vi "project.vi"() -> ()   [LabVIEW 2017]
panel:
  in  "aOK Button 75":bool
  in  "aOK Button 74":bool
  in  "aOK Button 65":bool
  in  "aOK Button 73":bool
  in  "aOK Button 72":bool
  in  "aOK Button 71":bool
  in  "aOK Button 70":bool
  in  "aOK Button 69":bool
  in  "aOK Button 68":bool
  in  "aOK Button 67":bool
  in  "aOK Button 66":bool
  in  "aOK Button 64":bool
  in  "aOK Button 63":bool
  in  "aOK Button 62":bool
  in  "aOK Button 61":bool
  in  "aOK Button 60":bool
  in  "aOK Button 59":bool
  in  "aOK Button 58":bool
  in  "aOK Button 56":bool
  in  "aOK Button 55":bool
  in  "aOK Button 54":bool
  in  "aOK Button 53":bool
  in  "aOK Button 52":bool
  in  "aOK Button 51":bool
  in  "aOK Button 50":bool
  in  "aOK Button 49":bool
  in  "aOK Button 48":bool
  in  "aOK Button 47":bool
  in  "aOK Button 46":bool
  in  "aOK Button 45":bool
  in  "aOK Button 44":bool
  in  "aOK Button 42":bool
  in  "aOK Button 41":bool
  in  "aOK Button 40":bool
  in  "aOK Button 39":bool
  in  "aOK Button 38":bool
  in  "aOK Button 37":bool
  in  "aOK Button 36":bool
  in  "aOK Button 30":bool
  in  "aOK Button 27":bool
  in  "aOK Button 34":bool
  in  "aOK Button 35":bool
  in  "aOK Button 33":bool
  in  "aOK Button 32":bool
  in  "aOK Button 31":bool
  in  "aOK Button 29":bool
  in  "aOK Button 28":bool
  in  "aOK Button 26":bool
  in  "aOK Button 25":bool
  in  "aOK Button 24":bool
  in  "aOK Button 23":bool
  in  "aOK Button 22":bool
  in  "aOK Button 21":bool
  in  "aOK Button 20":bool
  in  "aOK Button 19":bool
  in  "aOK Button 18":bool
  in  "aOK Button 17":bool
  in  "aOK Button 15":bool
  in  "aOK Button 14":bool
  in  "aOK Button 13":bool
  in  "aOK Button 12":bool
  in  "aOK Button 11":bool
  in  "aOK Button 10":bool
  in  "aOK Button 9":bool
  in  "aOK Button 8":bool
  in  "aOK Button 7":bool
  in  "aOK Button 6":bool
  in  "aOK Button 5":bool
  in  "aOK Button 4":bool
  in  "aOK Button 3":bool
  in  "aOK Button 2":bool
  in  "aOK Button":bool
  out "Boolean 143":bool
  in  "Array 2":bool[][](array[boolean])
  in  "OK Button 165":bool
  in  "OK Button 164":bool
  in  "OK Button 163":bool
  in  "OK Button 162":bool
  in  "OK Button 161":bool
  in  "OK Button 160":bool
  in  "OK Button 159":bool
  in  "OK Button 158":bool
  in  "OK Button 157":bool
  in  "OK Button 156":bool
  in  "OK Button 155":bool
  in  "OK Button 154":bool
  in  "OK Button 153":bool
  in  "OK Button 152":bool
  in  "OK Button 151":bool
  in  "OK Button 150":bool
  in  "OK Button 149":bool
  in  "OK Button 148":bool
  in  "OK Button 147":bool
  in  "OK Button 146":bool
  in  "OK Button 145":bool
  in  "OK Button 144":bool
  in  "OK Button 143":bool
  in  "OK Button 142":bool
  in  "OK Button 141":bool
  in  "OK Button 140":bool
  in  "OK Button 139":bool
  in  "OK Button 138":bool
  in  "OK Button 137":bool
  in  "OK Button 136":bool
  in  "OK Button 135":bool
  in  "OK Button 134":bool
  in  "OK Button 133":bool
  in  "OK Button 132":bool
  in  "OK Button 131":bool
  in  "OK Button 130":bool
  in  "OK Button 129":bool
  in  "OK Button 128":bool
  in  "OK Button 127":bool
  in  "OK Button 126":bool
  in  "OK Button 125":bool
  in  "OK Button 124":bool
  in  "OK Button 122":bool
  in  "OK Button 118":bool
  in  "OK Button 113":bool
  in  "OK Button 104":bool
  in  "OK Button 89":bool
  in  "OK Button 121":bool
  in  "OK Button 117":bool
  in  "OK Button 112":bool
  in  "OK Button 103":bool
  in  "OK Button 88":bool
  in  "OK Button 123":bool
  in  "OK Button 120":bool
  in  "OK Button 119":bool
  in  "OK Button 116":bool
  in  "OK Button 115":bool
  in  "OK Button 114":bool
  in  "OK Button 111":bool
  in  "OK Button 110":bool
  in  "OK Button 109":bool
  in  "OK Button 108":bool
  in  "OK Button 107":bool
  in  "OK Button 105":bool
  in  "OK Button 102":bool
  in  "OK Button 101":bool
  in  "OK Button 100":bool
  in  "OK Button 99":bool
  in  "OK Button 97":bool
  in  "OK Button 96":bool
  in  "OK Button 95":bool
  in  "OK Button 93":bool
  in  "OK Button 92":bool
  in  "OK Button 91":bool
  in  "OK Button 90":bool
  in  "OK Button 87":bool
  in  "OK Button 86":bool
  in  "OK Button 85":bool
  in  "OK Button 84":bool
  in  "OK Button 83":bool
  in  "OK Button 82":bool
  in  "OK Button 81":bool
  in  "OK Button 80":bool
  in  "OK Button 79":bool
  in  "OK Button 78":bool
  in  "OK Button 77":bool
  in  "Array":bool[][](array[boolean])
  out "Boolean 142":bool
  in  "OK Button 76":bool
  in  "OK Button 75":bool
  in  "OK Button 74":bool
  in  "OK Button 73":bool
  in  "OK Button 72":bool
  in  "OK Button 71":bool
  in  "OK Button 70":bool
  in  "OK Button 69":bool
  in  "OK Button 68":bool
  in  "OK Button 59":bool
  in  "OK Button 50":bool
  in  "OK Button 49":bool
  in  "OK Button 67":bool
  in  "OK Button 58":bool
  in  "OK Button 66":bool
  in  "OK Button 48":bool
  in  "OK Button 65":bool
  in  "OK Button 46":bool
  in  "OK Button 45":bool
  in  "OK Button 64":bool
  in  "OK Button 57":bool
  in  "OK Button 44":bool
  in  "OK Button 63":bool
  in  "OK Button 62":bool
  in  "OK Button 61":bool
  in  "OK Button 60":bool
  out "Boolean 141":bool
  in  "OK Button 56":bool
  in  "OK Button 55":bool
  in  "OK Button 54":bool
  in  "OK Button 53":bool
  in  "OK Button 52":bool
  in  "OK Button 51":bool
  in  "OK Button 47":bool
  in  "OK Button 43":bool
  in  "OK Button 42":bool
  in  "OK Button 41":bool
  in  "OK Button 40":bool
  in  "OK Button 39":bool
  in  "OK Button 38":bool
  in  "OK Button 37":bool
  in  "OK Button 36":bool
  in  "OK Button 35":bool
  in  "OK Button 34":bool
  in  "OK Button 33":bool
  in  "OK Button 32":bool
  in  "OK Button 31":bool
  in  "Boolean 140":bool
  in  "Boolean 139":bool
  in  "Boolean 138":bool
  in  "Boolean 137":bool
  in  "Boolean 136":bool
  in  "Boolean 135":bool
  in  "Boolean 134":bool
  in  "Boolean 133":bool
  in  "Boolean 132":bool
  in  "Boolean 131":bool
  in  "Boolean 130":bool
  in  "OK Button 28":bool
  in  "OK Button 27":bool
  in  "OK Button 26":bool
  in  "OK Button 25":bool
  in  "OK Button 24":bool
  in  "OK Button 23":bool
  in  "OK Button 22":bool
  in  "OK Button 21":bool
  in  "OK Button 17":bool
  in  "OK Butto":bool
  in  "Boolean 129":bool
  in  "Boolean 128":bool
  in  "Boolean 127":bool
  in  "Boolean 126":bool
  in  "Boolean 125":bool
  in  "Boolean 124":bool
  in  "Boolean 123":bool
  in  "Boolean 122":bool
  in  "Boolean 121":bool
  in  "Boolean 120":bool
  in  "Boolean 119":bool
  in  "Boolean 118":bool
  in  "Boolean 117":bool
  in  "Boolean 116":bool
  in  "Boolean 115":bool
  in  "Boolean 114":bool
  in  "Boolean 113":bool
  in  "Boolean 112":bool
  in  "Boolean 111":bool
  in  "Boolean 110":bool
  in  "Boolean 109":bool
  in  "Boolean 108":bool
  in  "Boolean 107":bool
  in  "Boolean 106":bool
  in  "Boolean 105":bool
  in  "Boolean 104":bool
  in  "Boolean 103":bool
  in  "Boolean 102":bool
  in  "Boolean 101":bool
  in  "Boolean 100":bool
  in  "Boolean 99":bool
  in  "Boolean 98":bool
  in  "Boolean 97":bool
  in  "Boolean 96":bool
  in  "Boolean 95":bool
  in  "Boolean 94":bool
  in  "Boolean 93":bool
  in  "Boolean 92":bool
  in  "Boolean 91":bool
  in  "Boolean 90":bool
  in  "Boolean 89":bool
  in  "Boolean 88":bool
  in  "Boolean 87":bool
  in  "Boolean 86":bool
  in  "Boolean 85":bool
  in  "Boolean 84":bool
  in  "Boolean 83":bool
  in  "Boolean 82":bool
  in  "Boolean 81":bool
  in  "Boolean 80":bool
  in  "Boolean 79":bool
  in  "Boolean 78":bool
  in  "Boolean 77":bool
  in  "Boolean 76":bool
  in  "Boolean 75":bool
  in  "Boolean 74":bool
  in  "Boolean 73":bool
  in  "Boolean 72":bool
  in  "Boolean 71":bool
  in  "Boolean 70":bool
  in  "Boolean 69":bool
  in  "Boolean 68":bool
  in  "Boolean 67":bool
  in  "Boolean 66":bool
  in  "Boolean 65":bool
  in  "Boolean 64":bool
  in  "Boolean 63":bool
  in  "Boolean 62":bool
  in  "Boolean 61":bool
  in  "Boolean 60":bool
  in  "Boolean 59":bool
  in  "Boolean 58":bool
  in  "Boolean 57":bool
  in  "Boolean 56":bool
  in  "Boolean 55":bool
  in  "Boolean 54":bool
  in  "Boolean 53":bool
  in  "Boolean 52":bool
  in  "Boolean 51":bool
  in  "Boolean 50":bool
  in  "Boolean 49":bool
  in  "Boolean 48":bool
  in  "Boolean 47":bool
  in  "Boolean 46":bool
  in  "Boolean 45":bool
  in  "Boolean 44":bool
  in  "Boolean 41":bool
  in  "Boolean":bool
  out "Boolean 43":bool
  in  "OK Button 16":bool
  in  "OK Button 15":bool
  in  "OK Button 14":bool
  in  "OK Button 13":bool
  in  "OK Button 12":bool
  in  "OK Button 11":bool
  in  "OK Button 10":bool
  in  "OK Button 9":bool
  in  "OK Button 8":bool
  in  "OK Button 7":bool
  in  "OK Button 6":bool
  in  "OK Button 5":bool
  in  "OK Button 4":bool
  in  "OK Button 3":bool
  in  "OK Button 2":bool
  in  "OK Button":bool
  in  "Boolean 42":bool
  in  "Boolean 40":bool
  in  "Boolean 39":bool
  in  "Boolean 38":bool
  in  "Boolean 37":bool
  in  "Boolean 36":bool
  in  "Boolean 35":bool
  in  "Boolean 34":bool
  in  "Boolean 33":bool
  in  "Boolean 32":bool
  in  "Boolean 31":bool
  in  "Boolean 30":bool
  in  "Boolean 29":bool
  in  "Boolean 28":bool
  in  "Boolean 27":bool
  in  "Boolean 26":bool
  in  "Boolean 25":bool
  in  "Boolean 24":bool
  in  "Boolean 23":bool
  in  "Boolean 22":bool
  in  "Boolean 21":bool
  in  "Boolean 20":bool
  in  "Boolean 19":bool
  in  "Boolean 18":bool
  in  "Boolean 17":bool
  in  "Boolean 16":bool
  in  "Boolean 15":bool
  in  "Boolean 14":bool
  in  "Boolean 13":bool
  in  "Boolean 12":bool
  in  "Boolean 11":bool
  in  "Boolean 10":bool
  in  "Boolean 9":bool
  in  "Boolean 8":bool
  in  "Boolean 7":bool
  in  "Boolean 6":bool
  in  "Boolean 5":bool
  in  "Boolean 4":bool
  in  "Boolean 3":bool
  in  "Boolean 2":bool
types:
  T1 = enum16{"menu", "latwy", "trudny", "8x5", "11x9", "12x15", "13x14", "powrot", "koniec"}
  T2 = enum16{"menu", "latwy", "trudny", "8x5", "11x9", "12x15", "13x14", "powrot"}
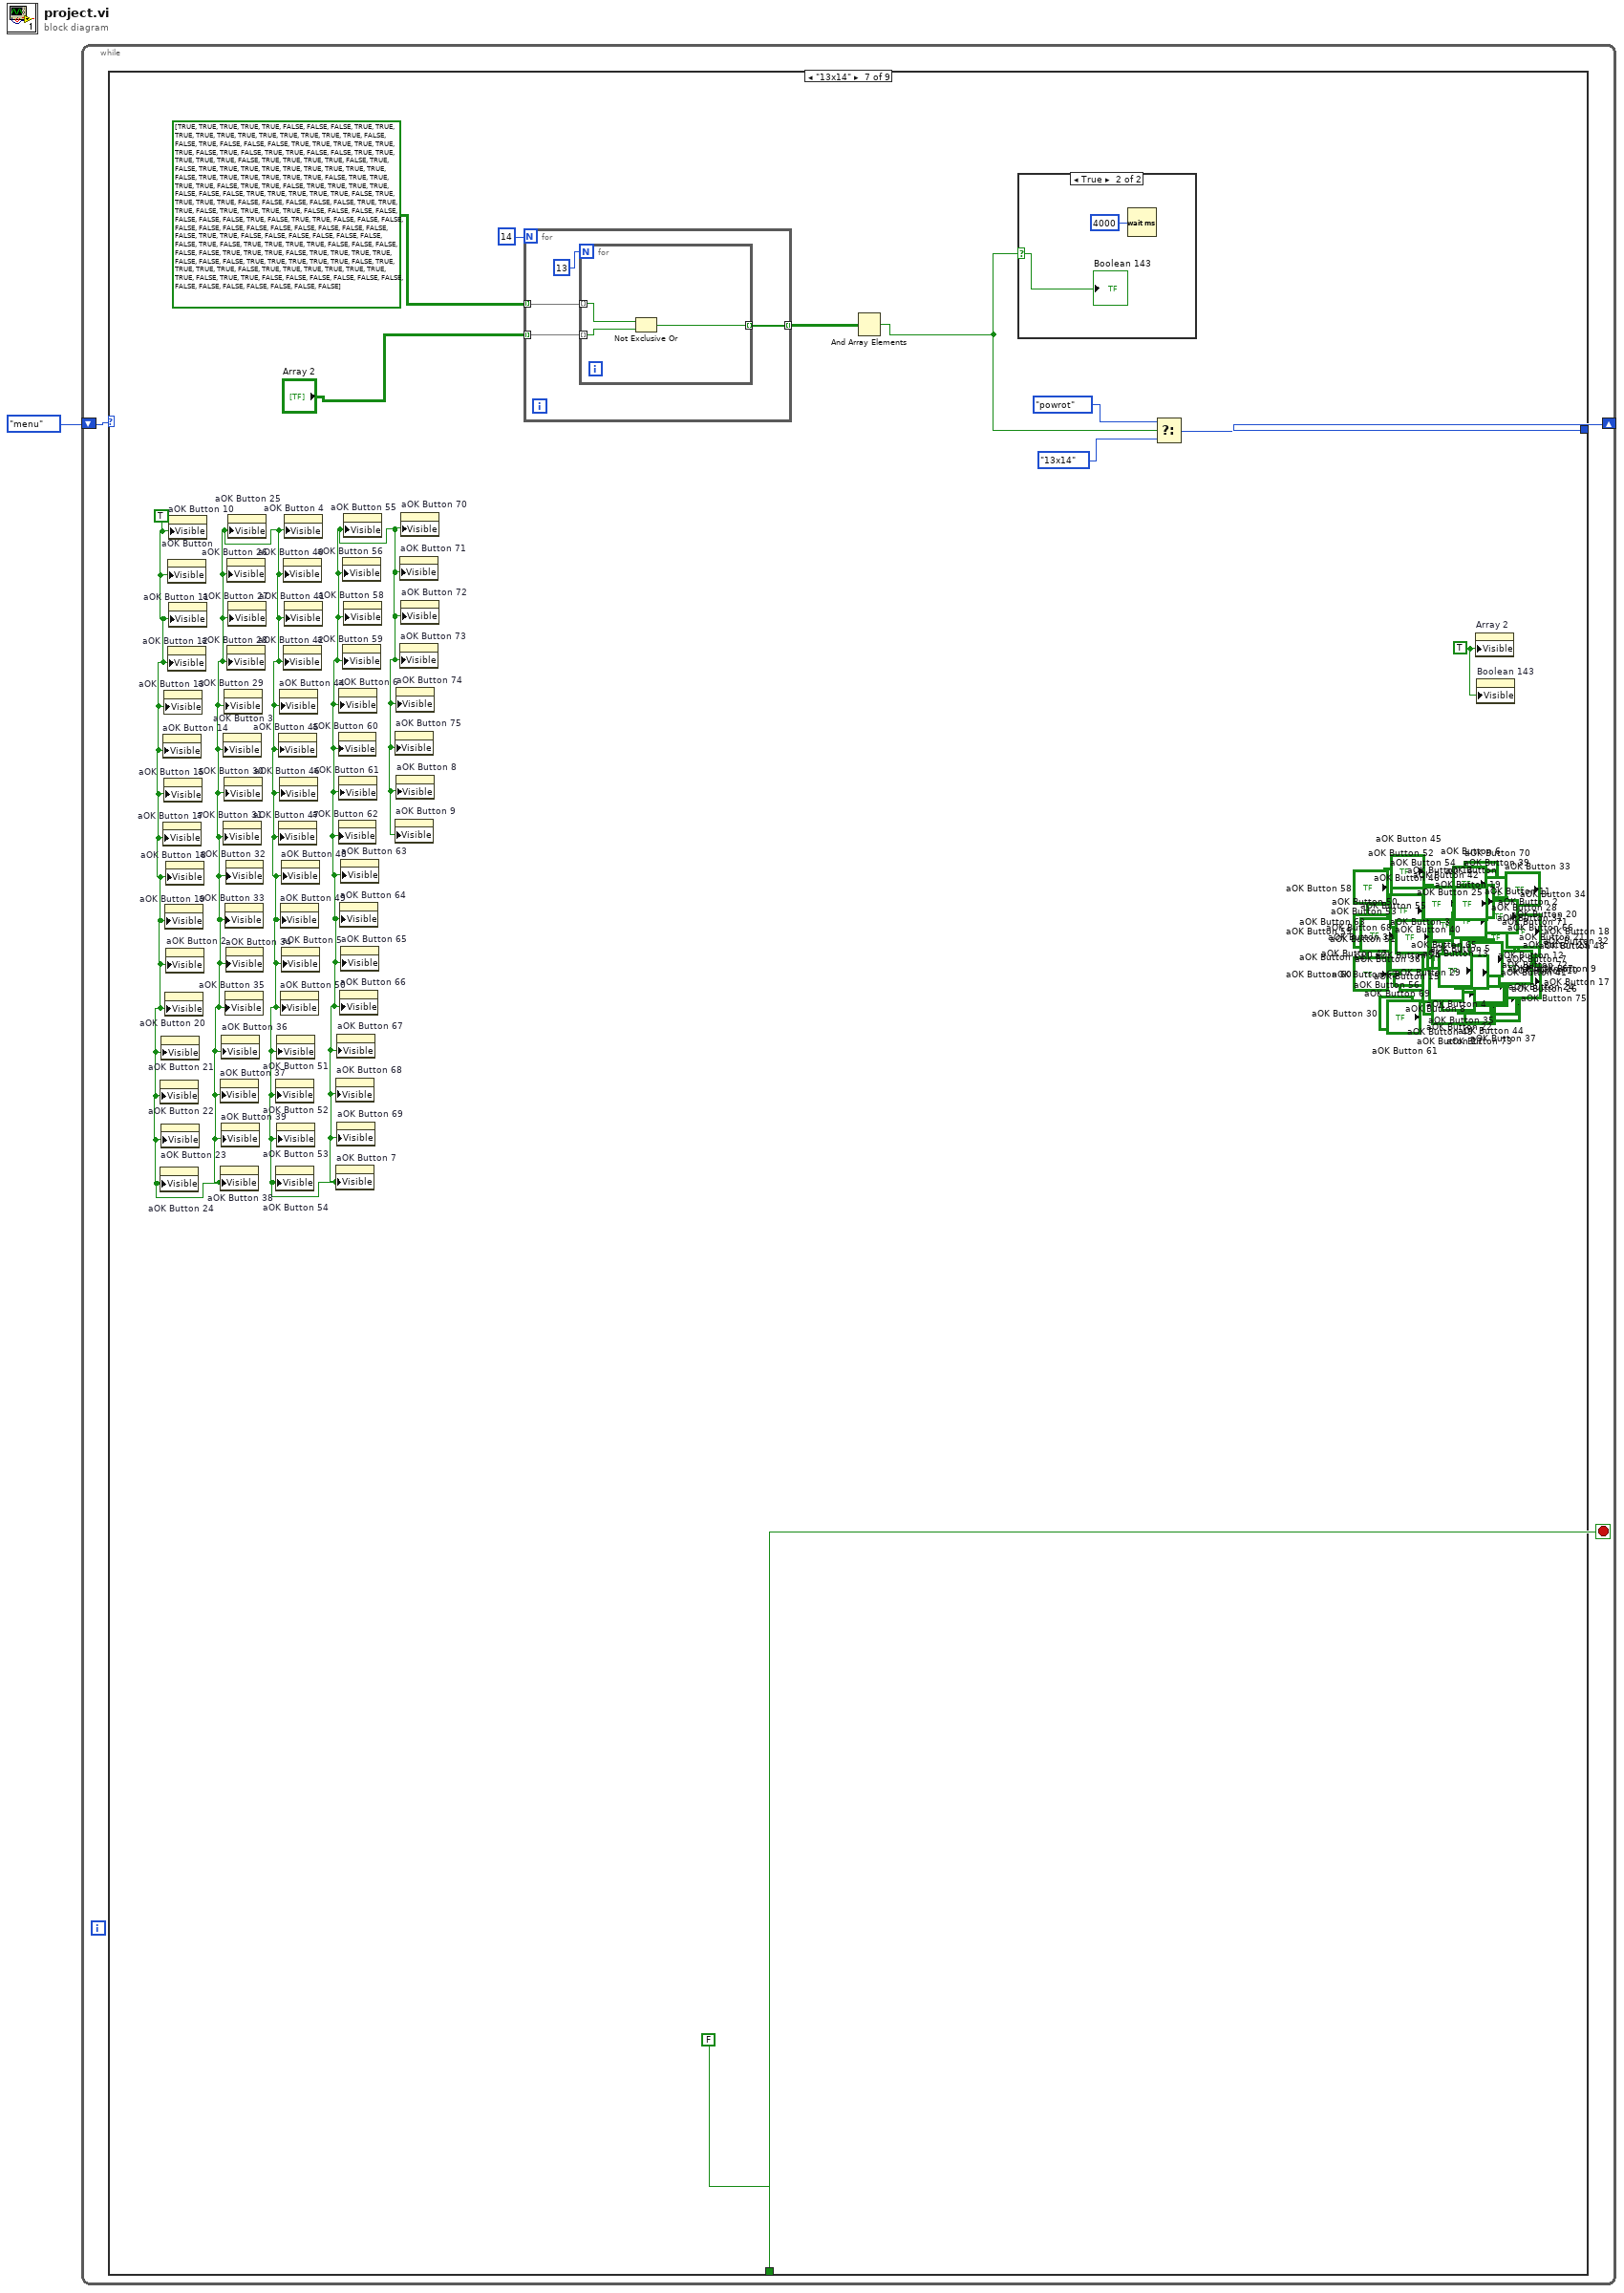
[diagram p0: block diagram]
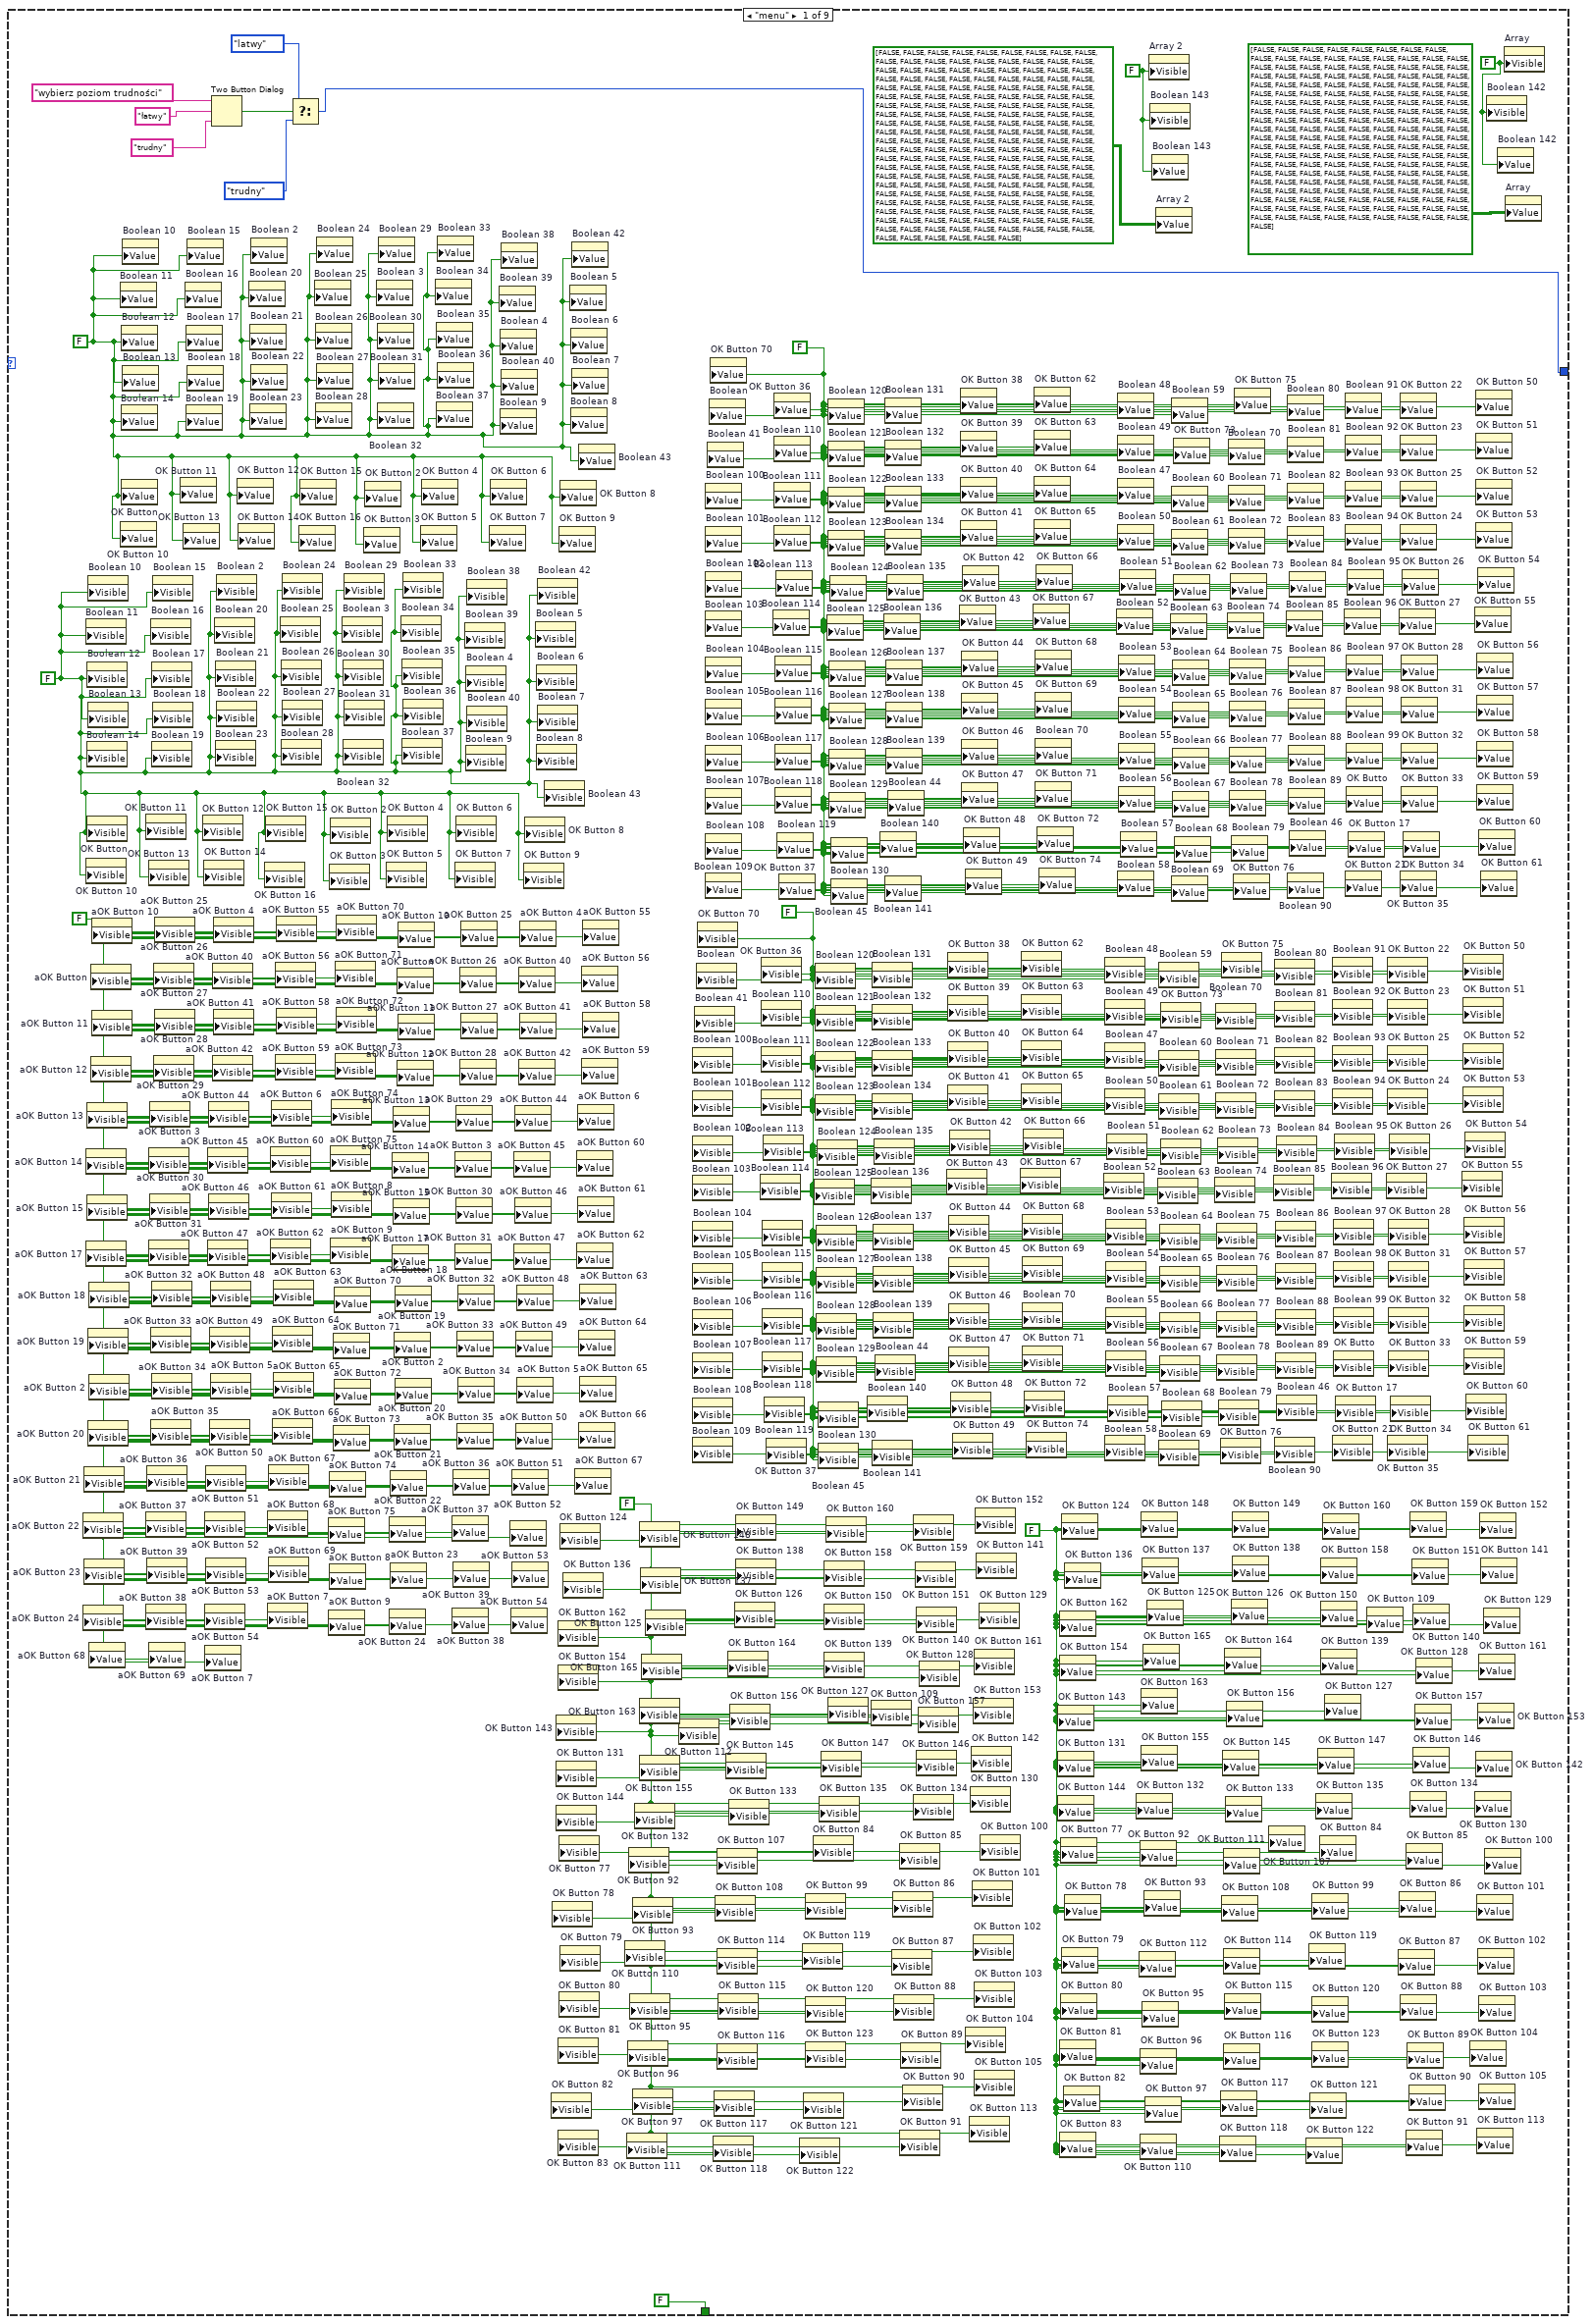
[diagram p2: hidden frame]
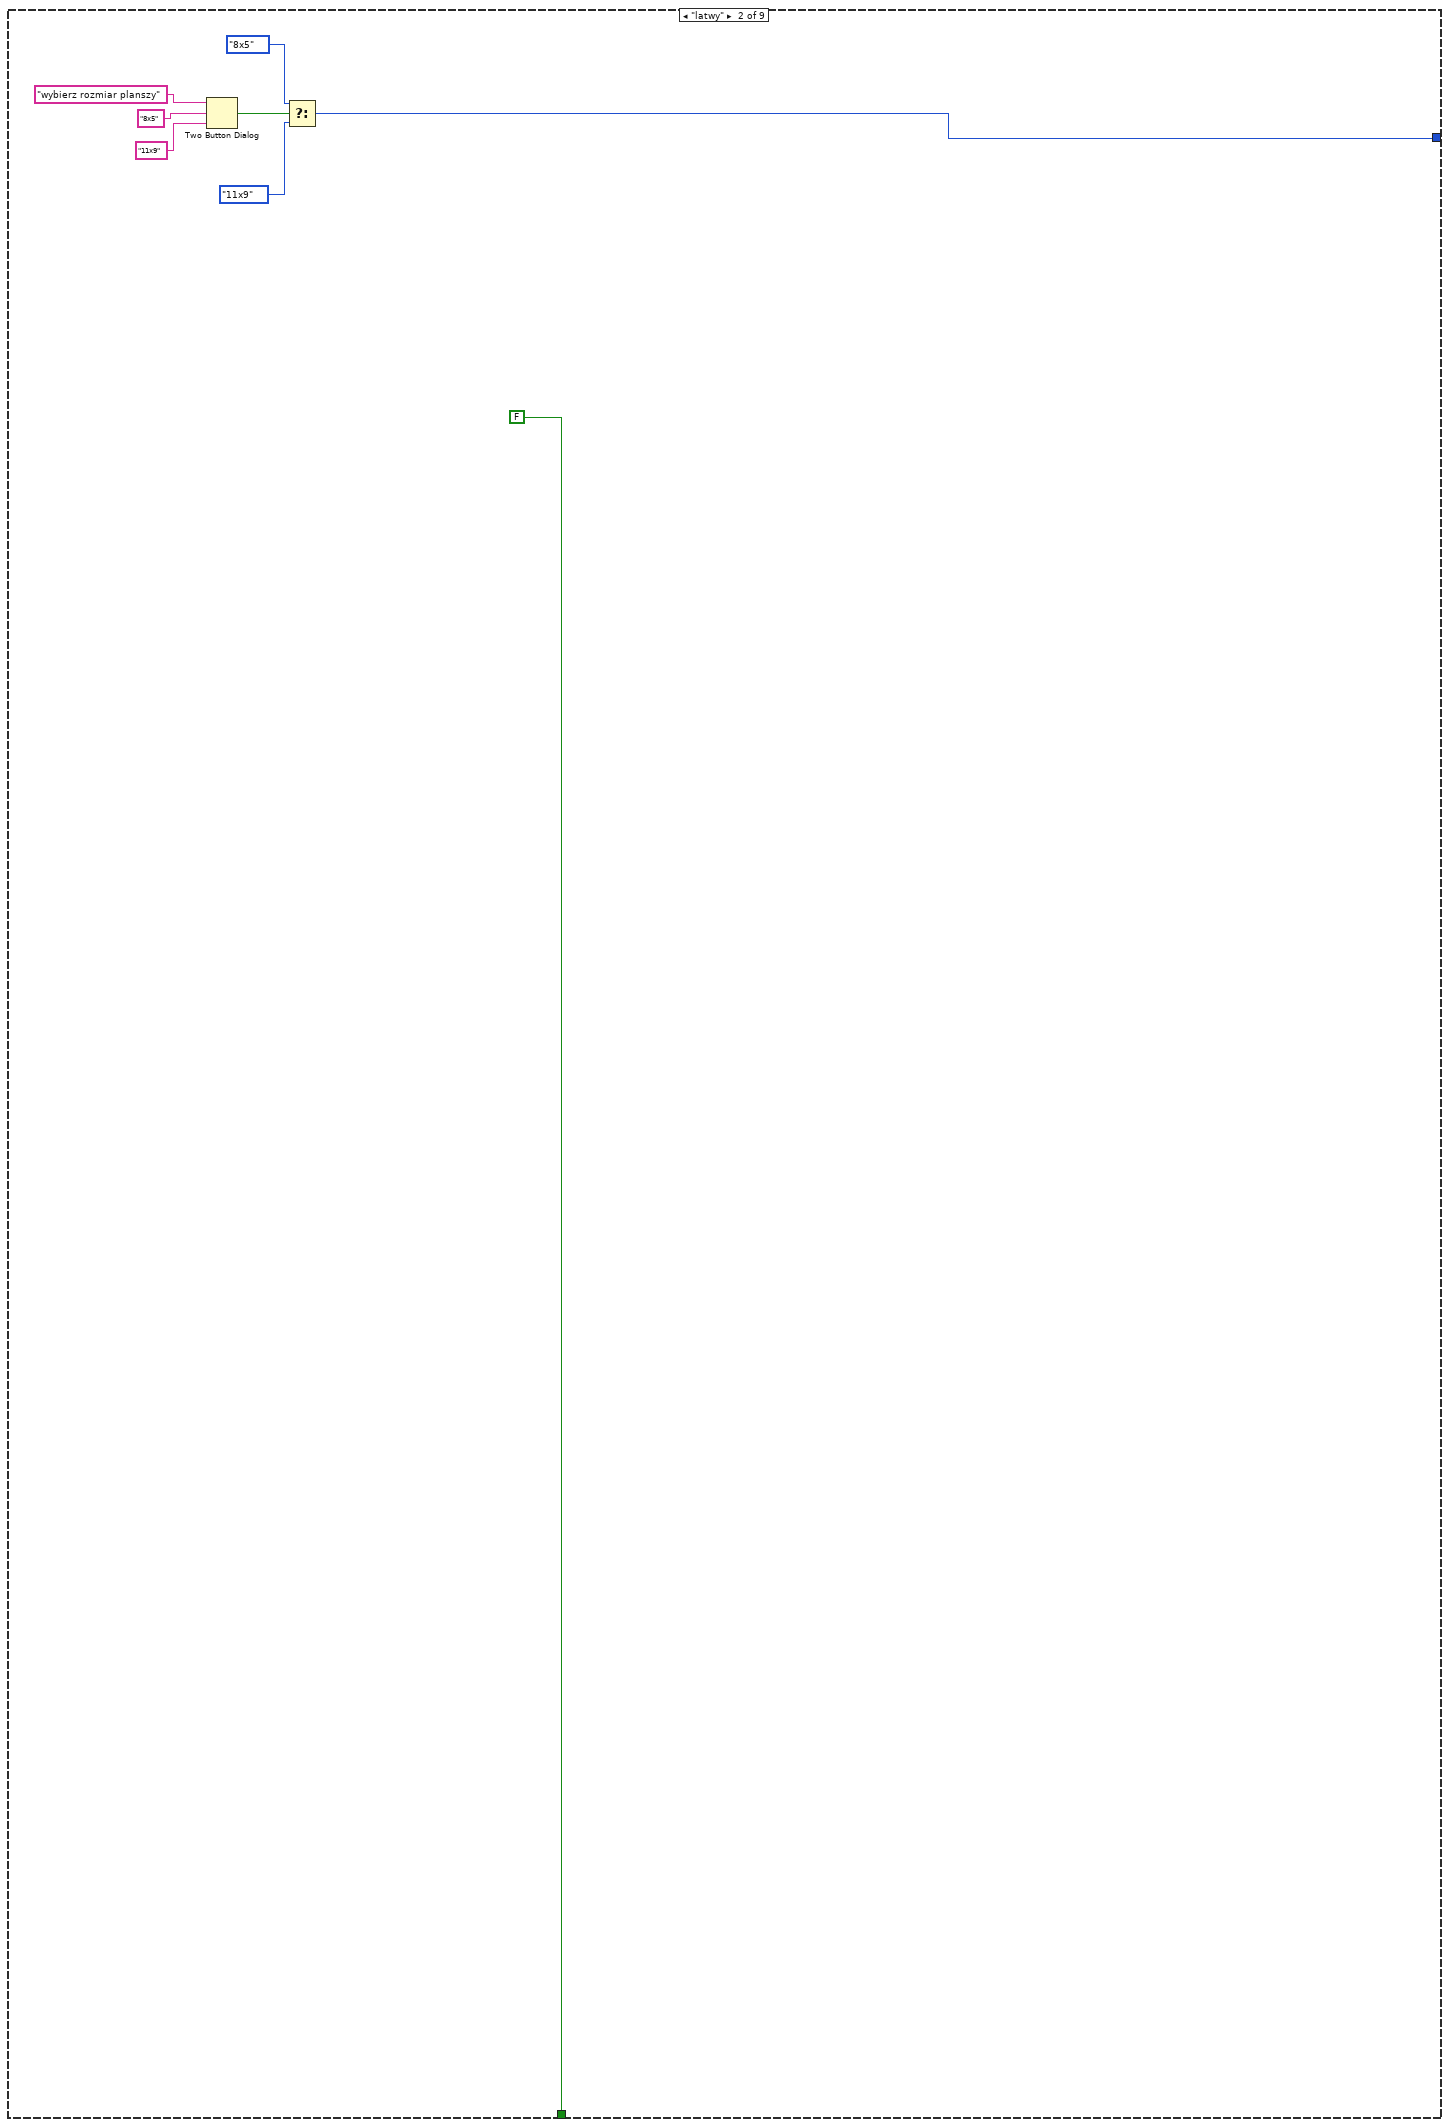
[diagram p3: hidden frame]
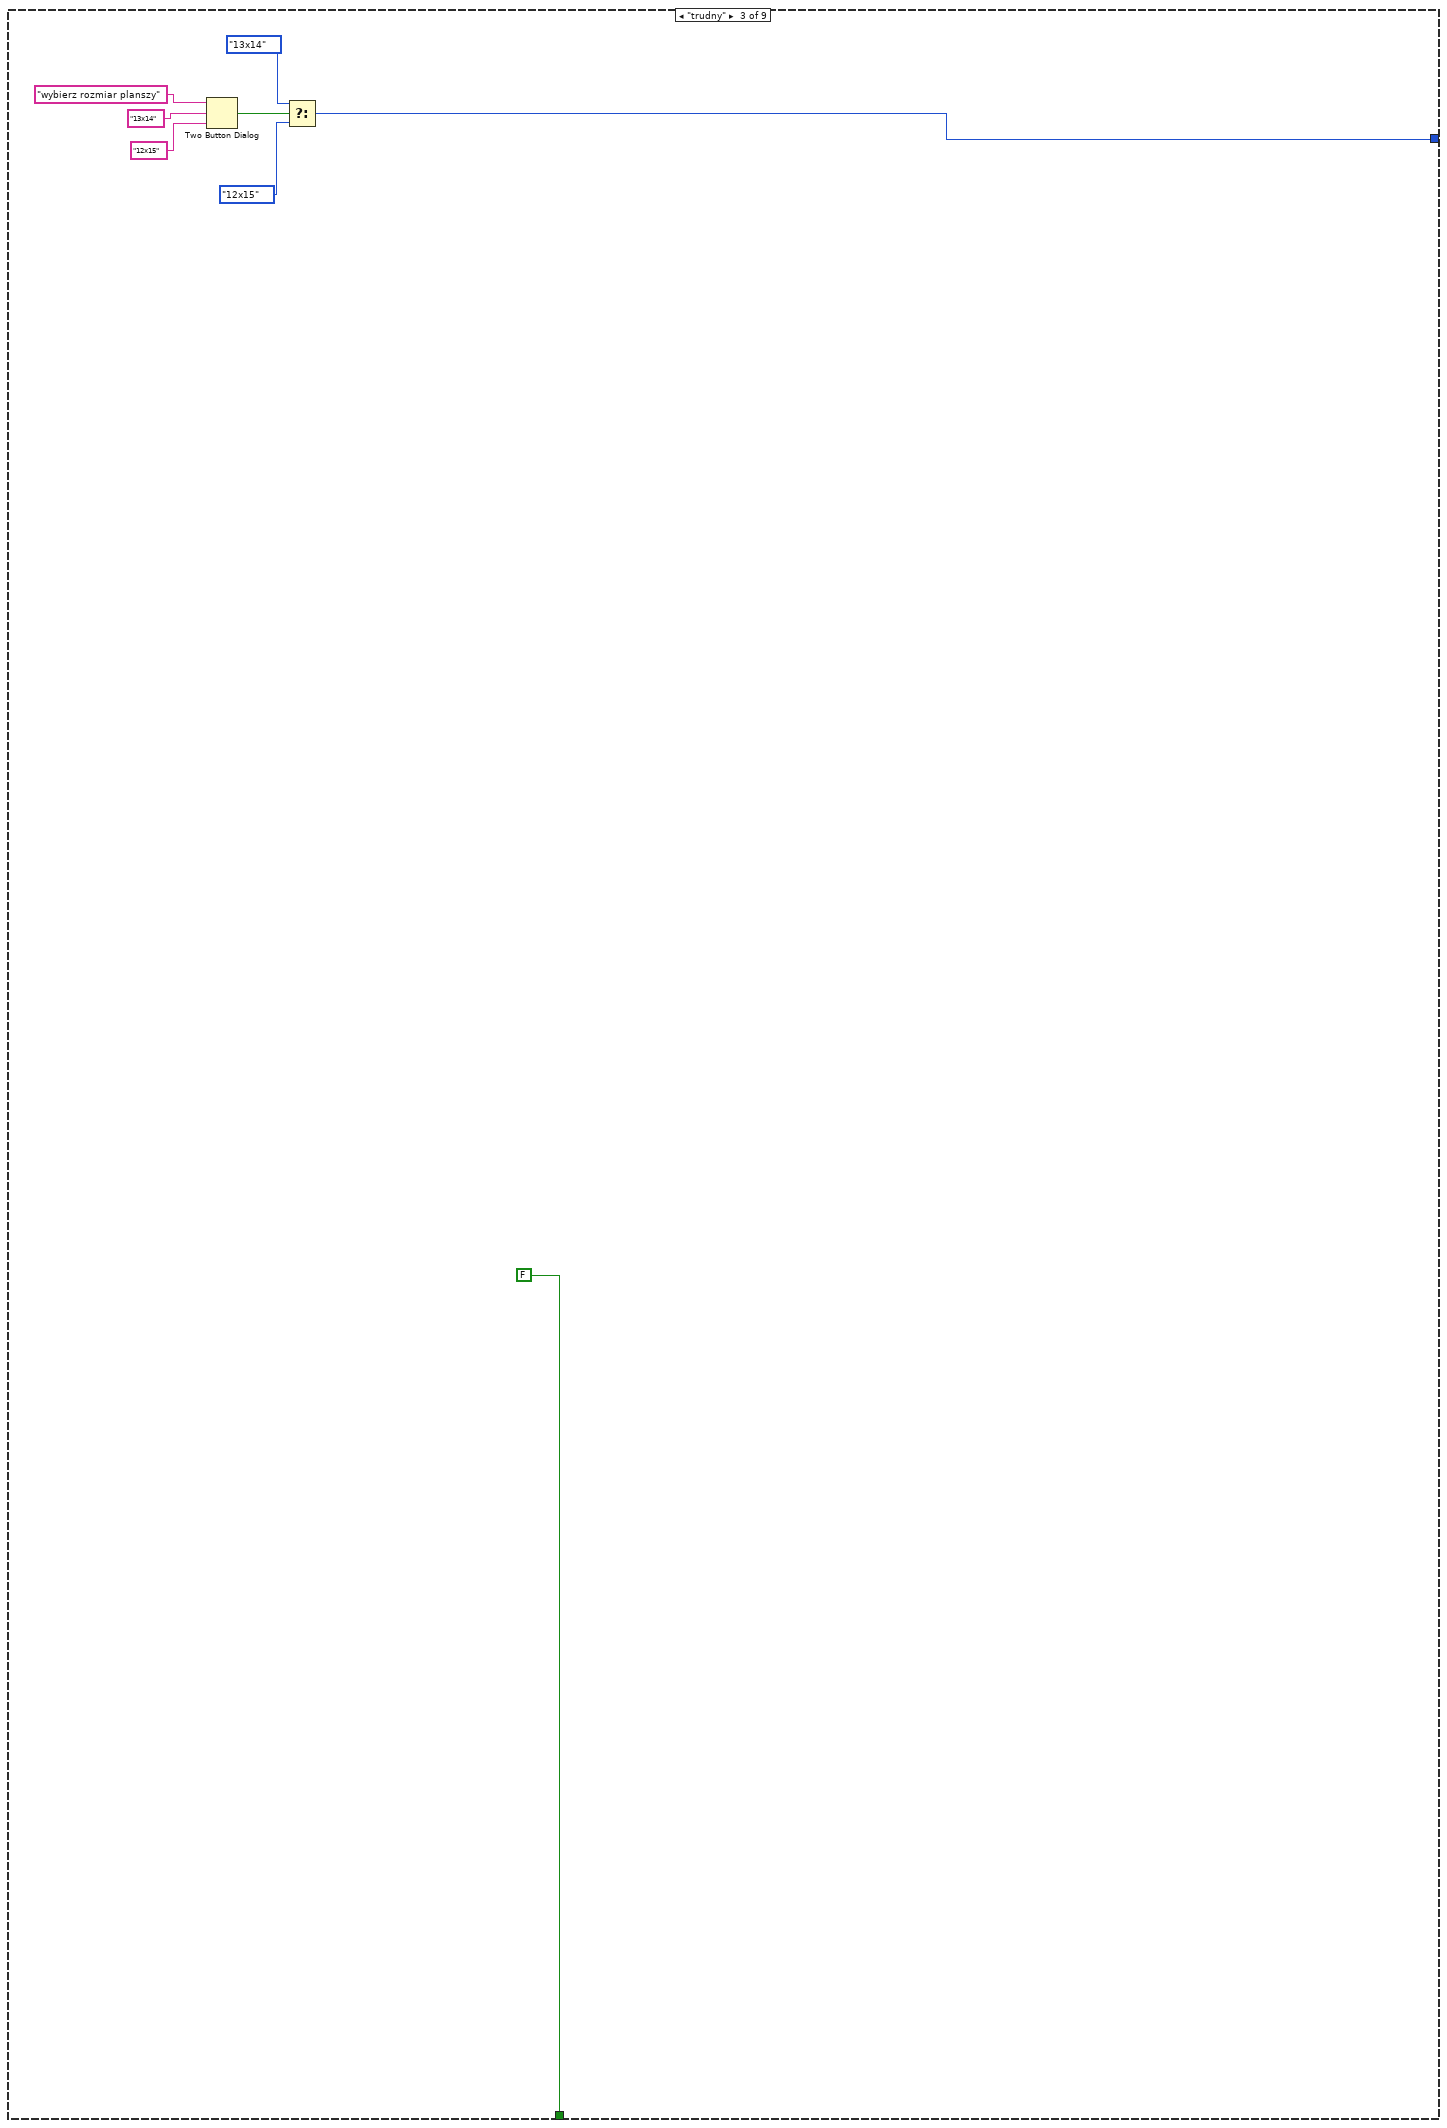
[diagram p4: hidden frame]
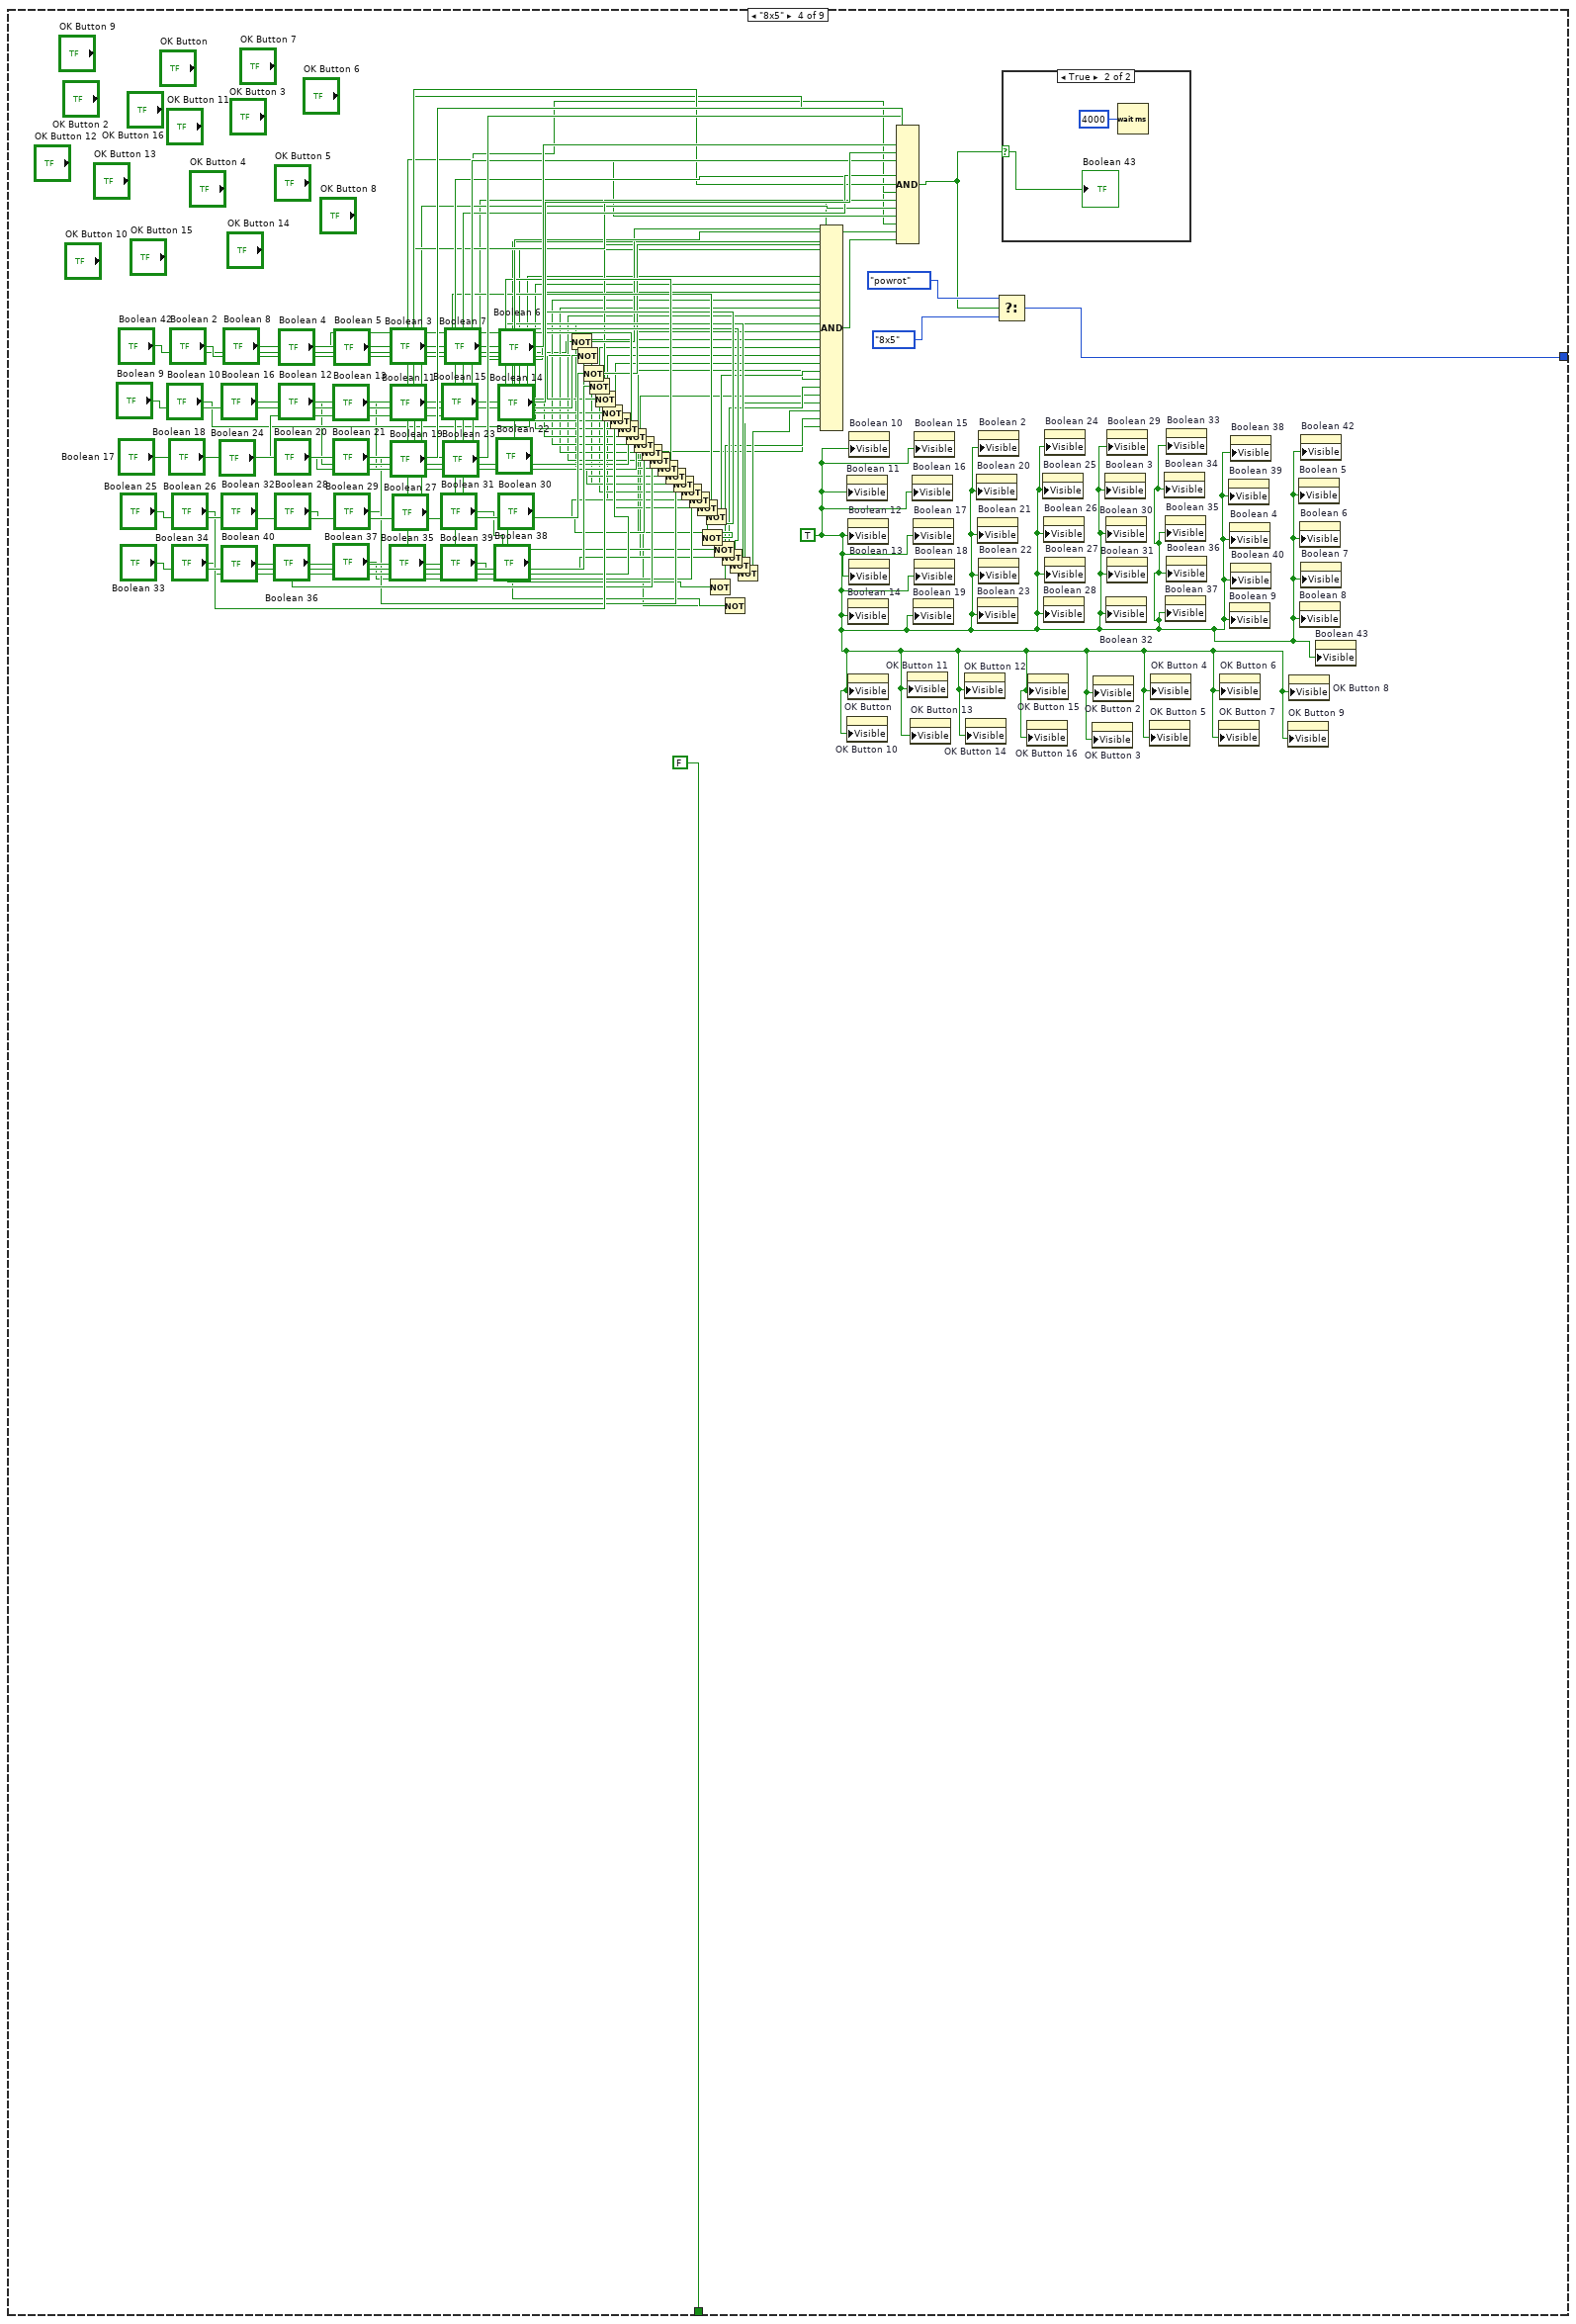
[diagram p5: hidden frame]
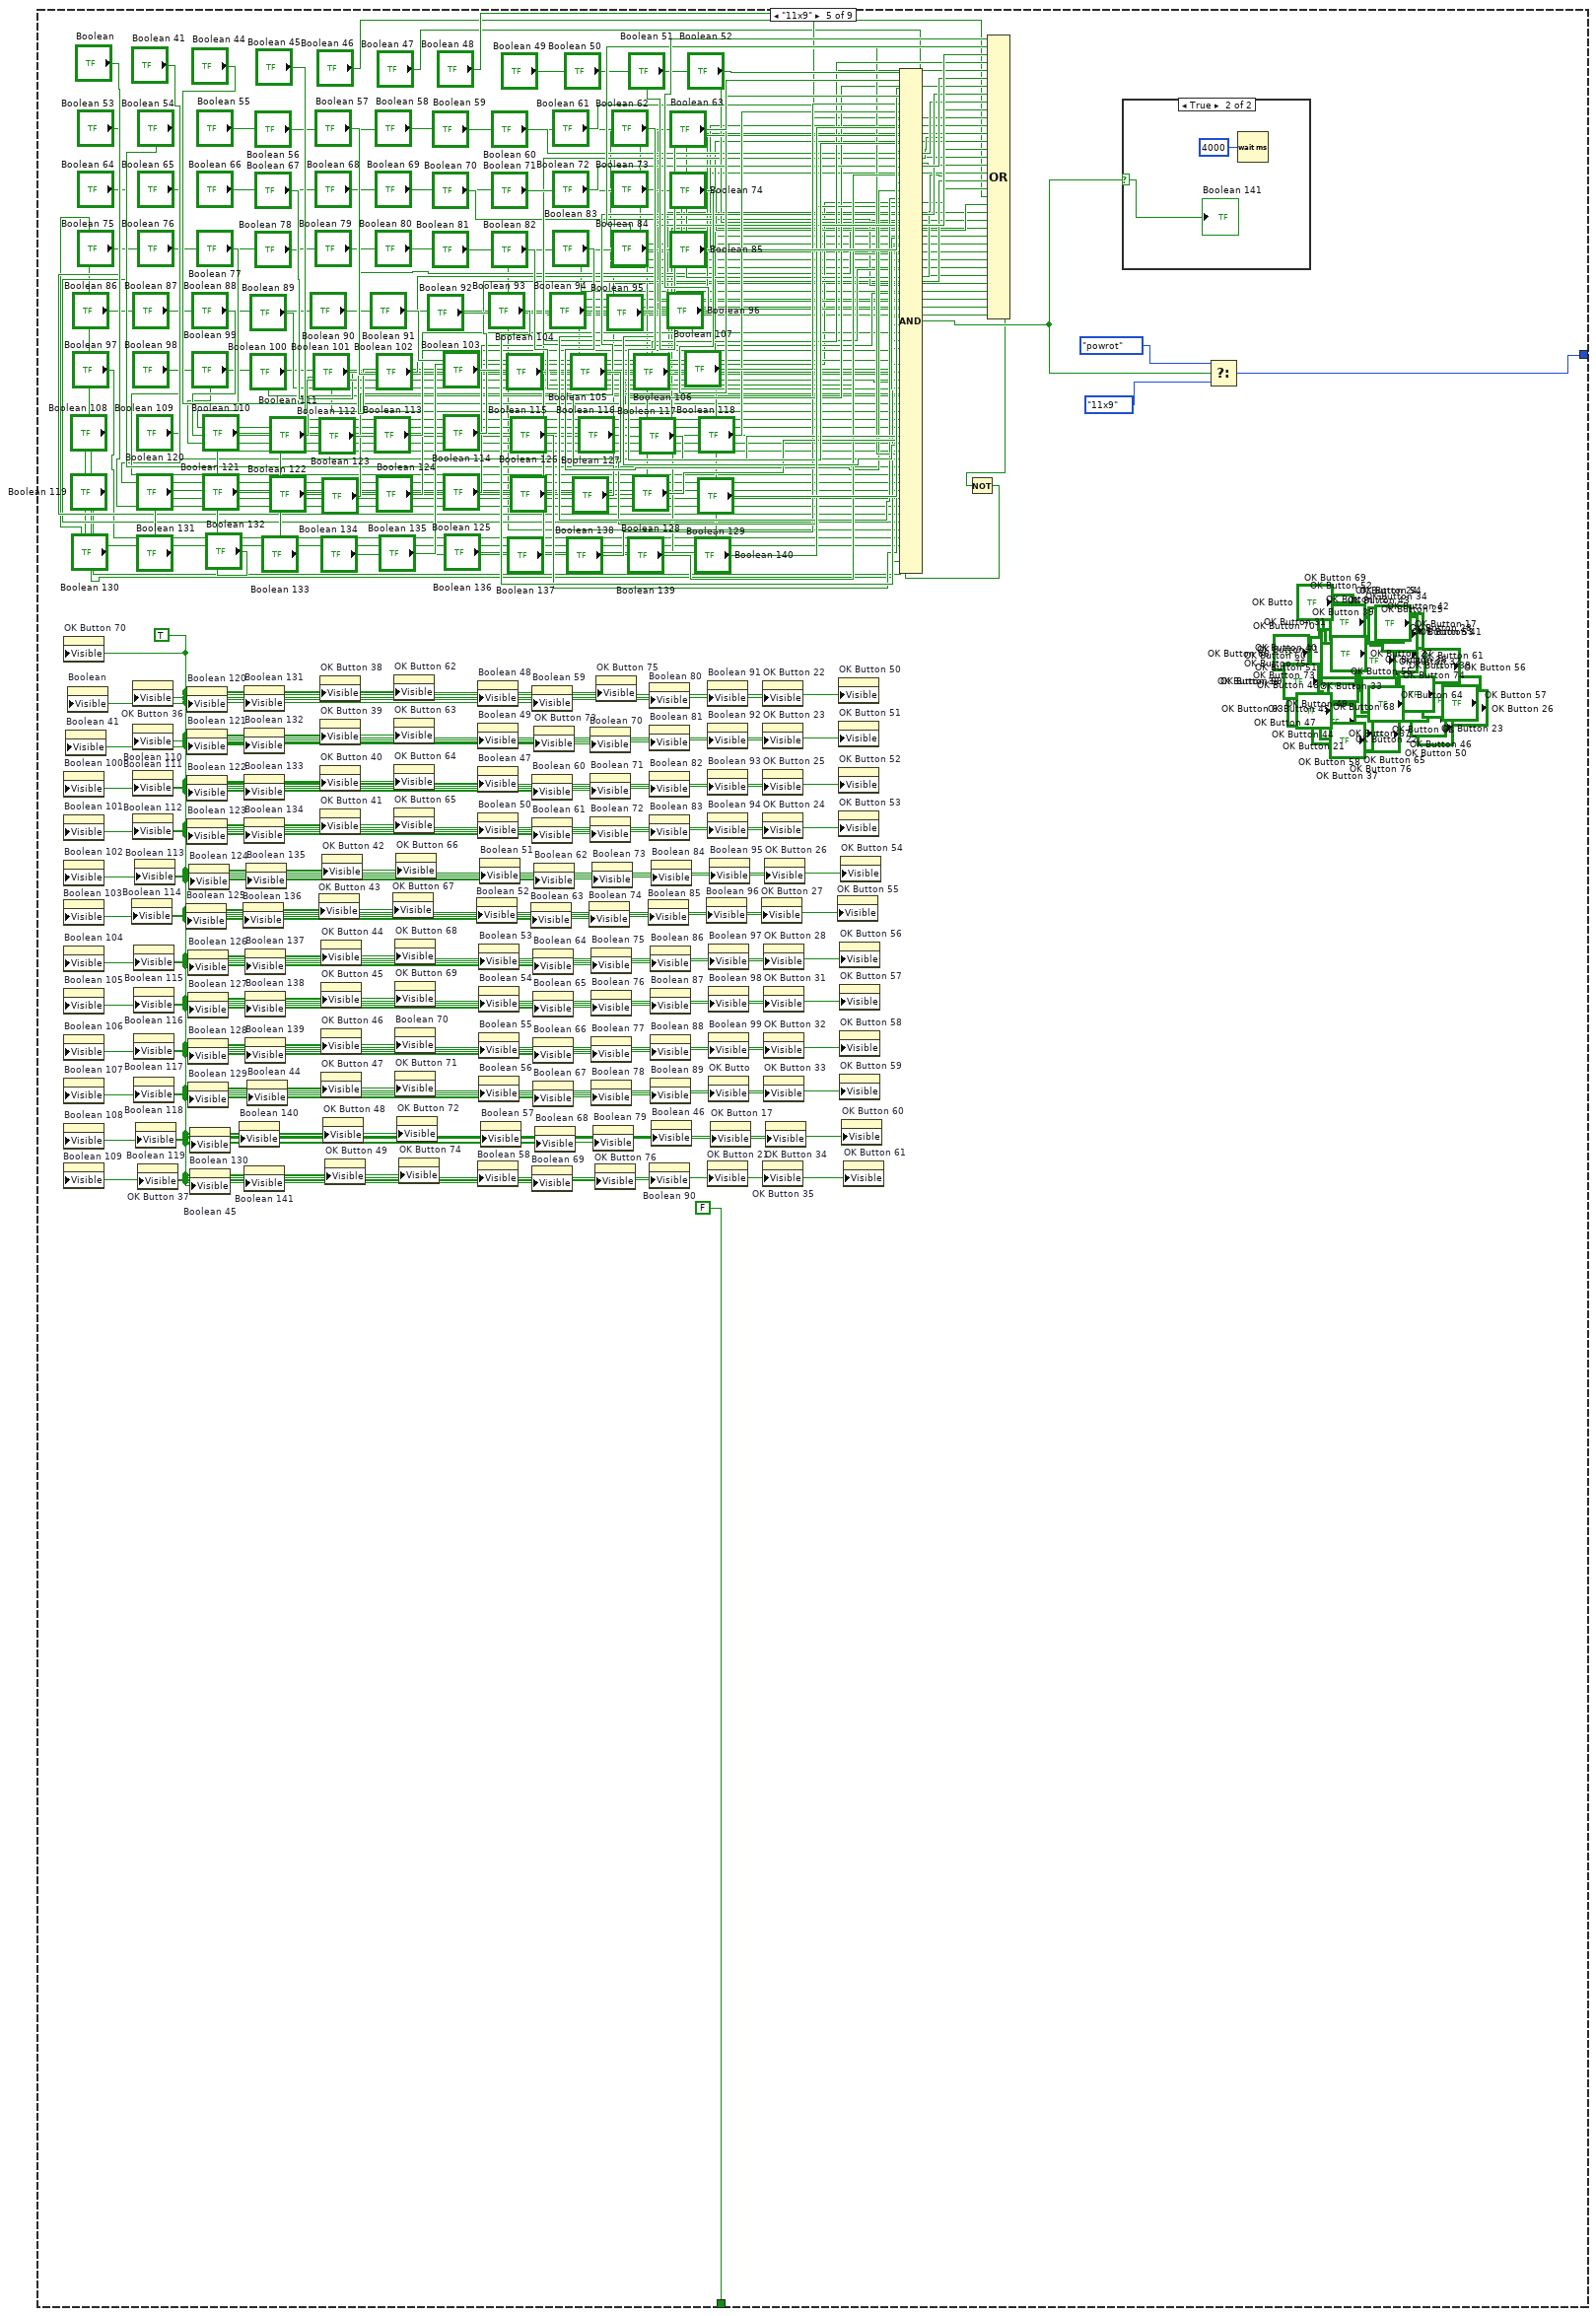
[diagram p7: hidden frame]
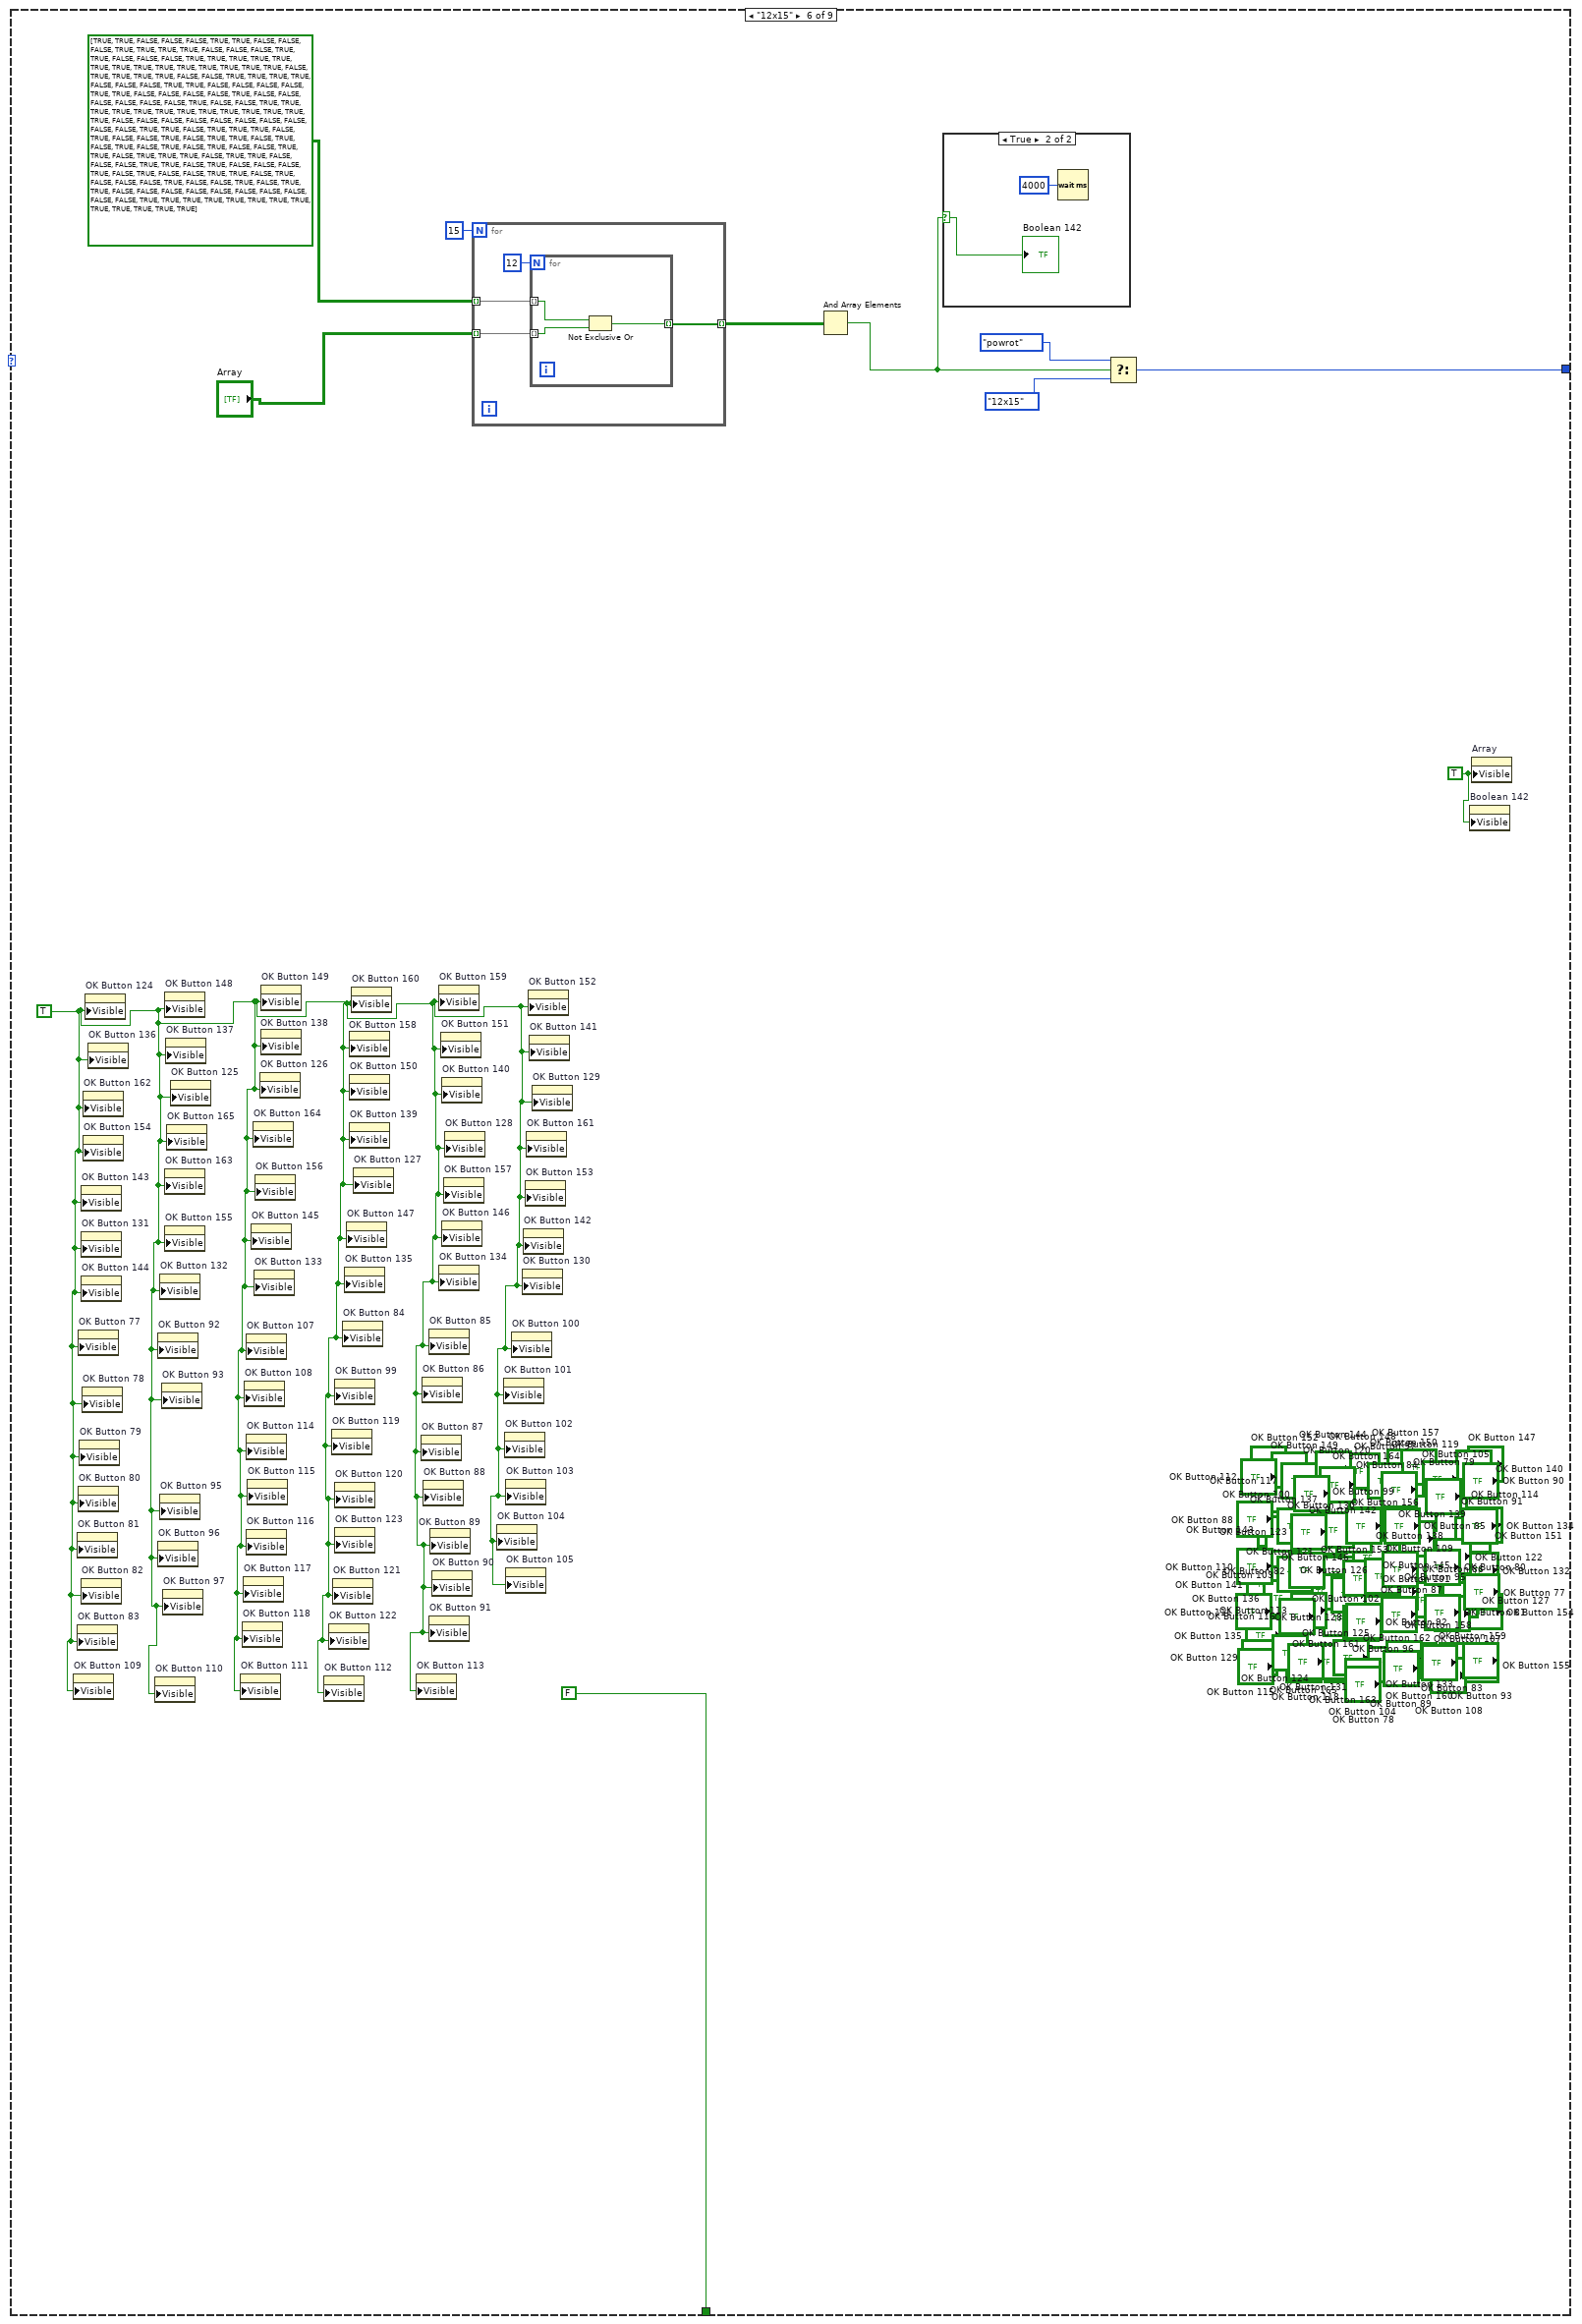
[diagram p9: hidden frame]
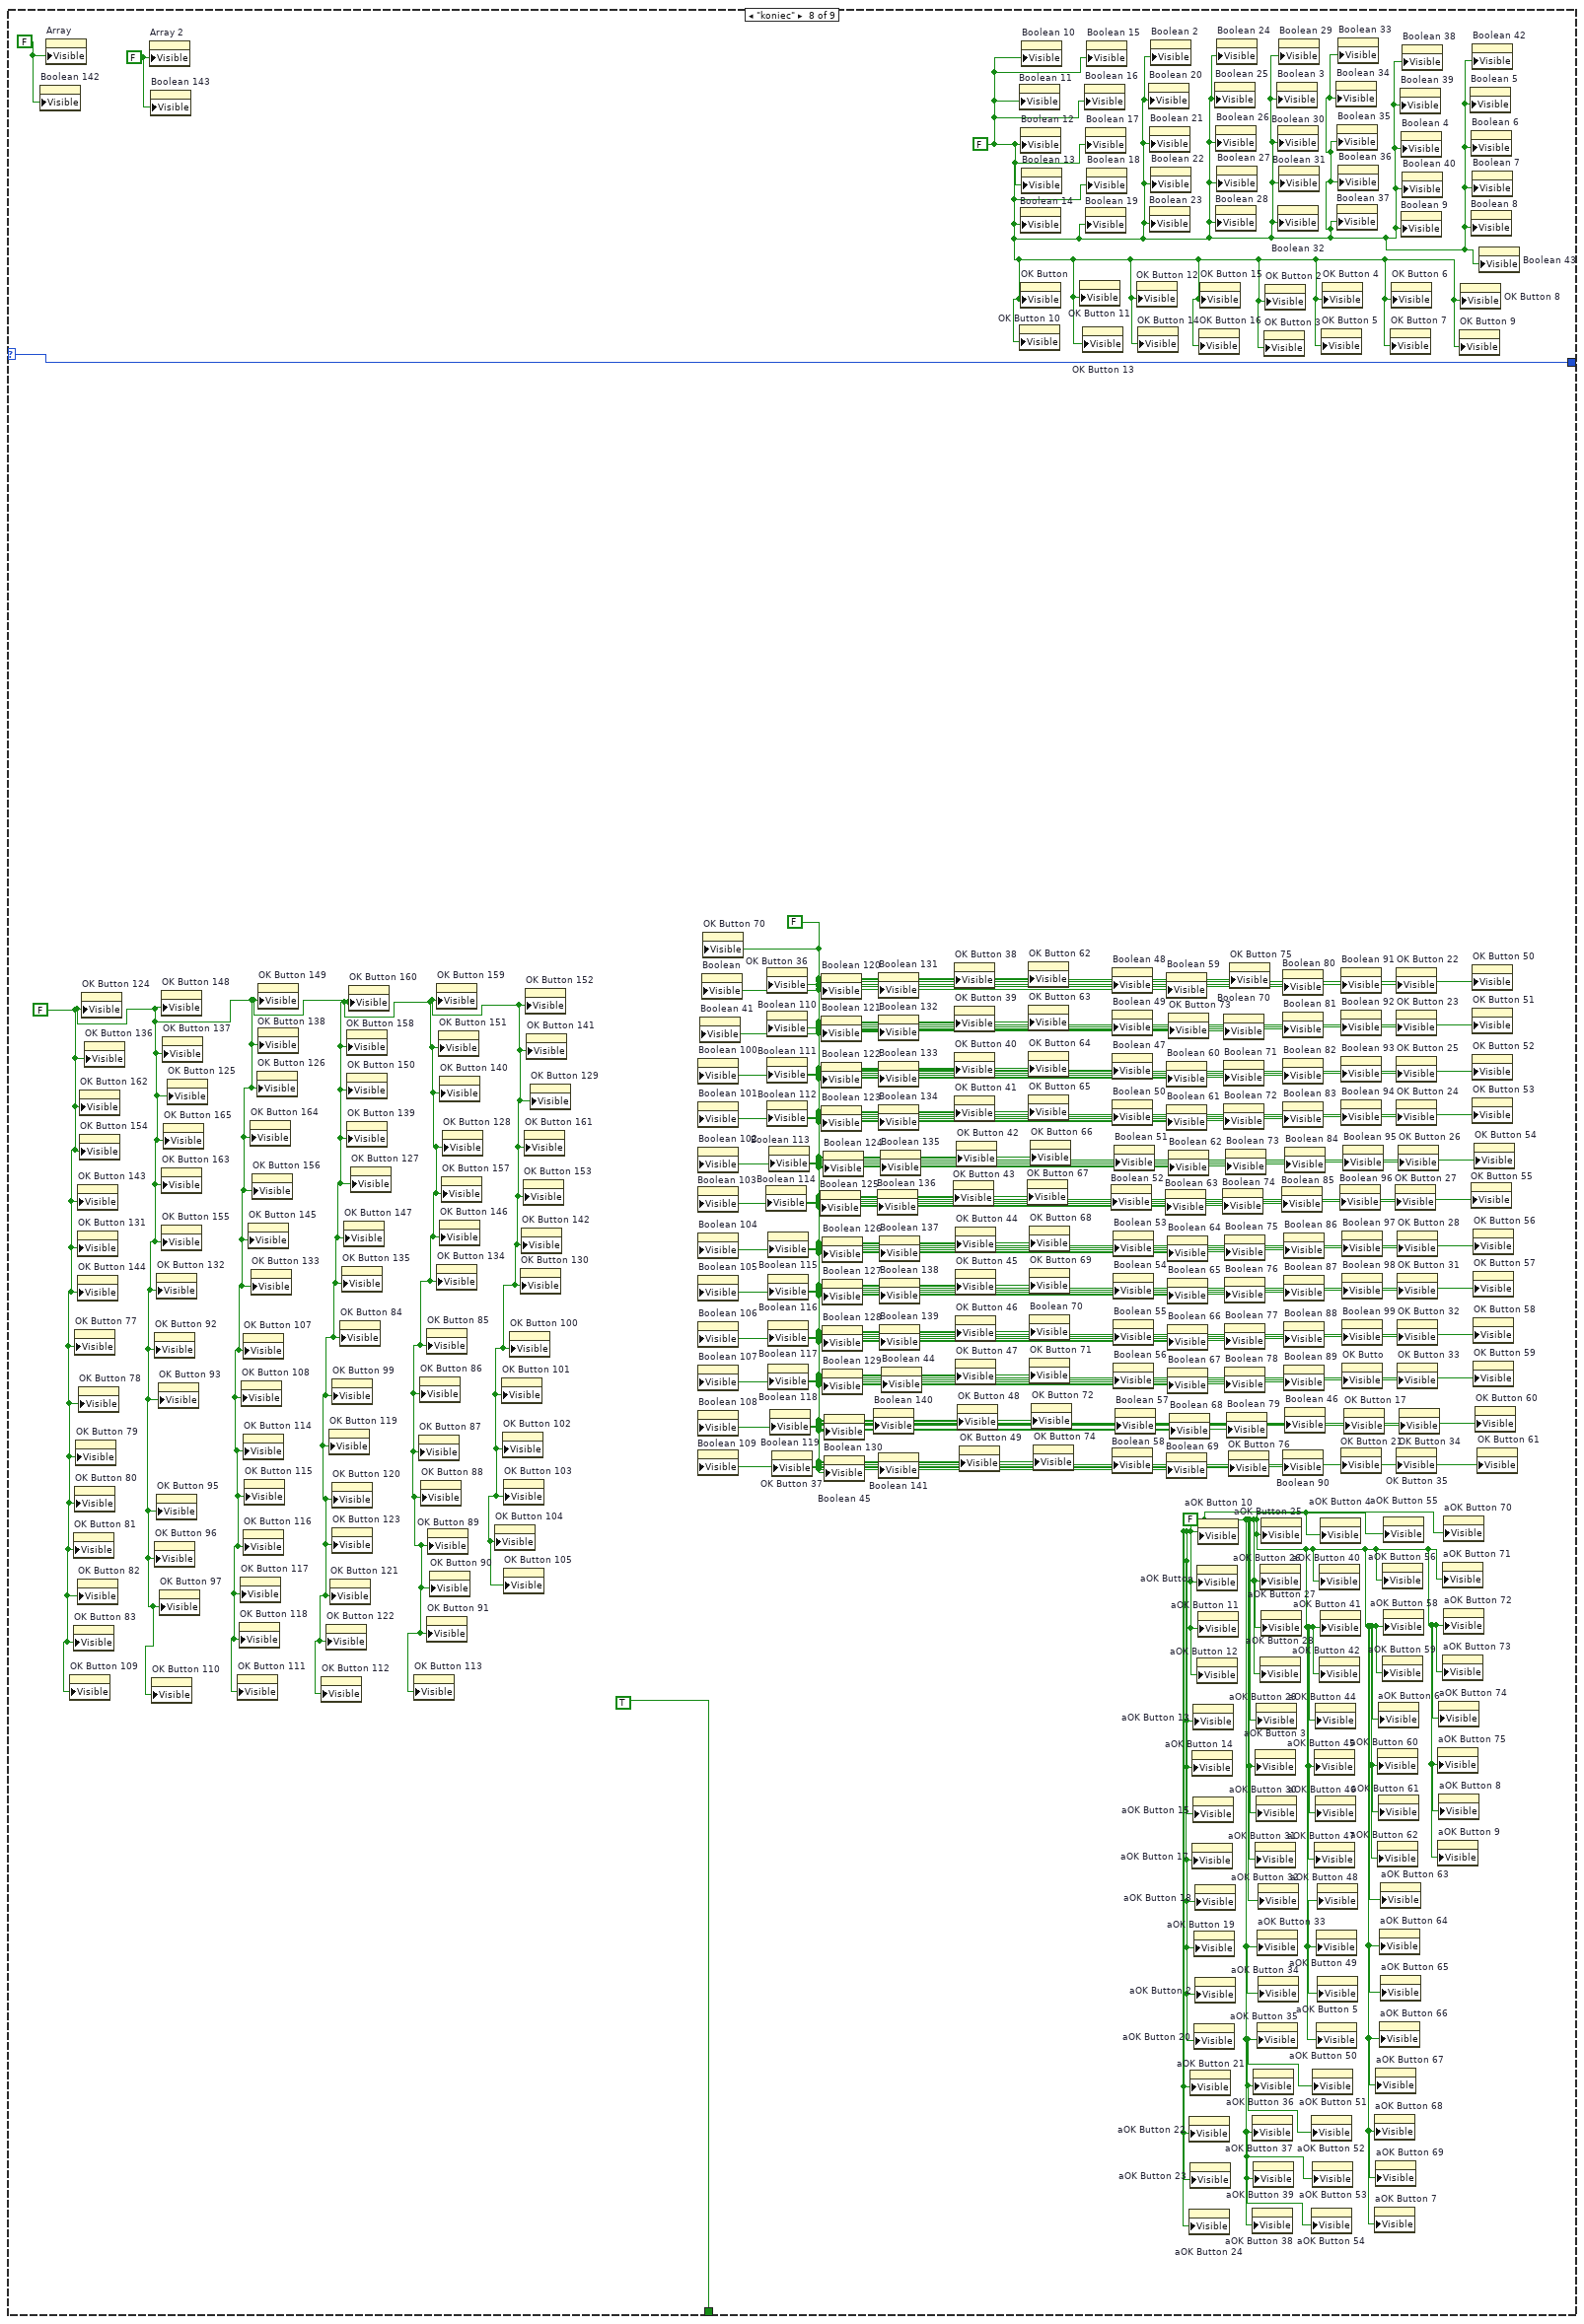
[diagram p12: hidden frame]
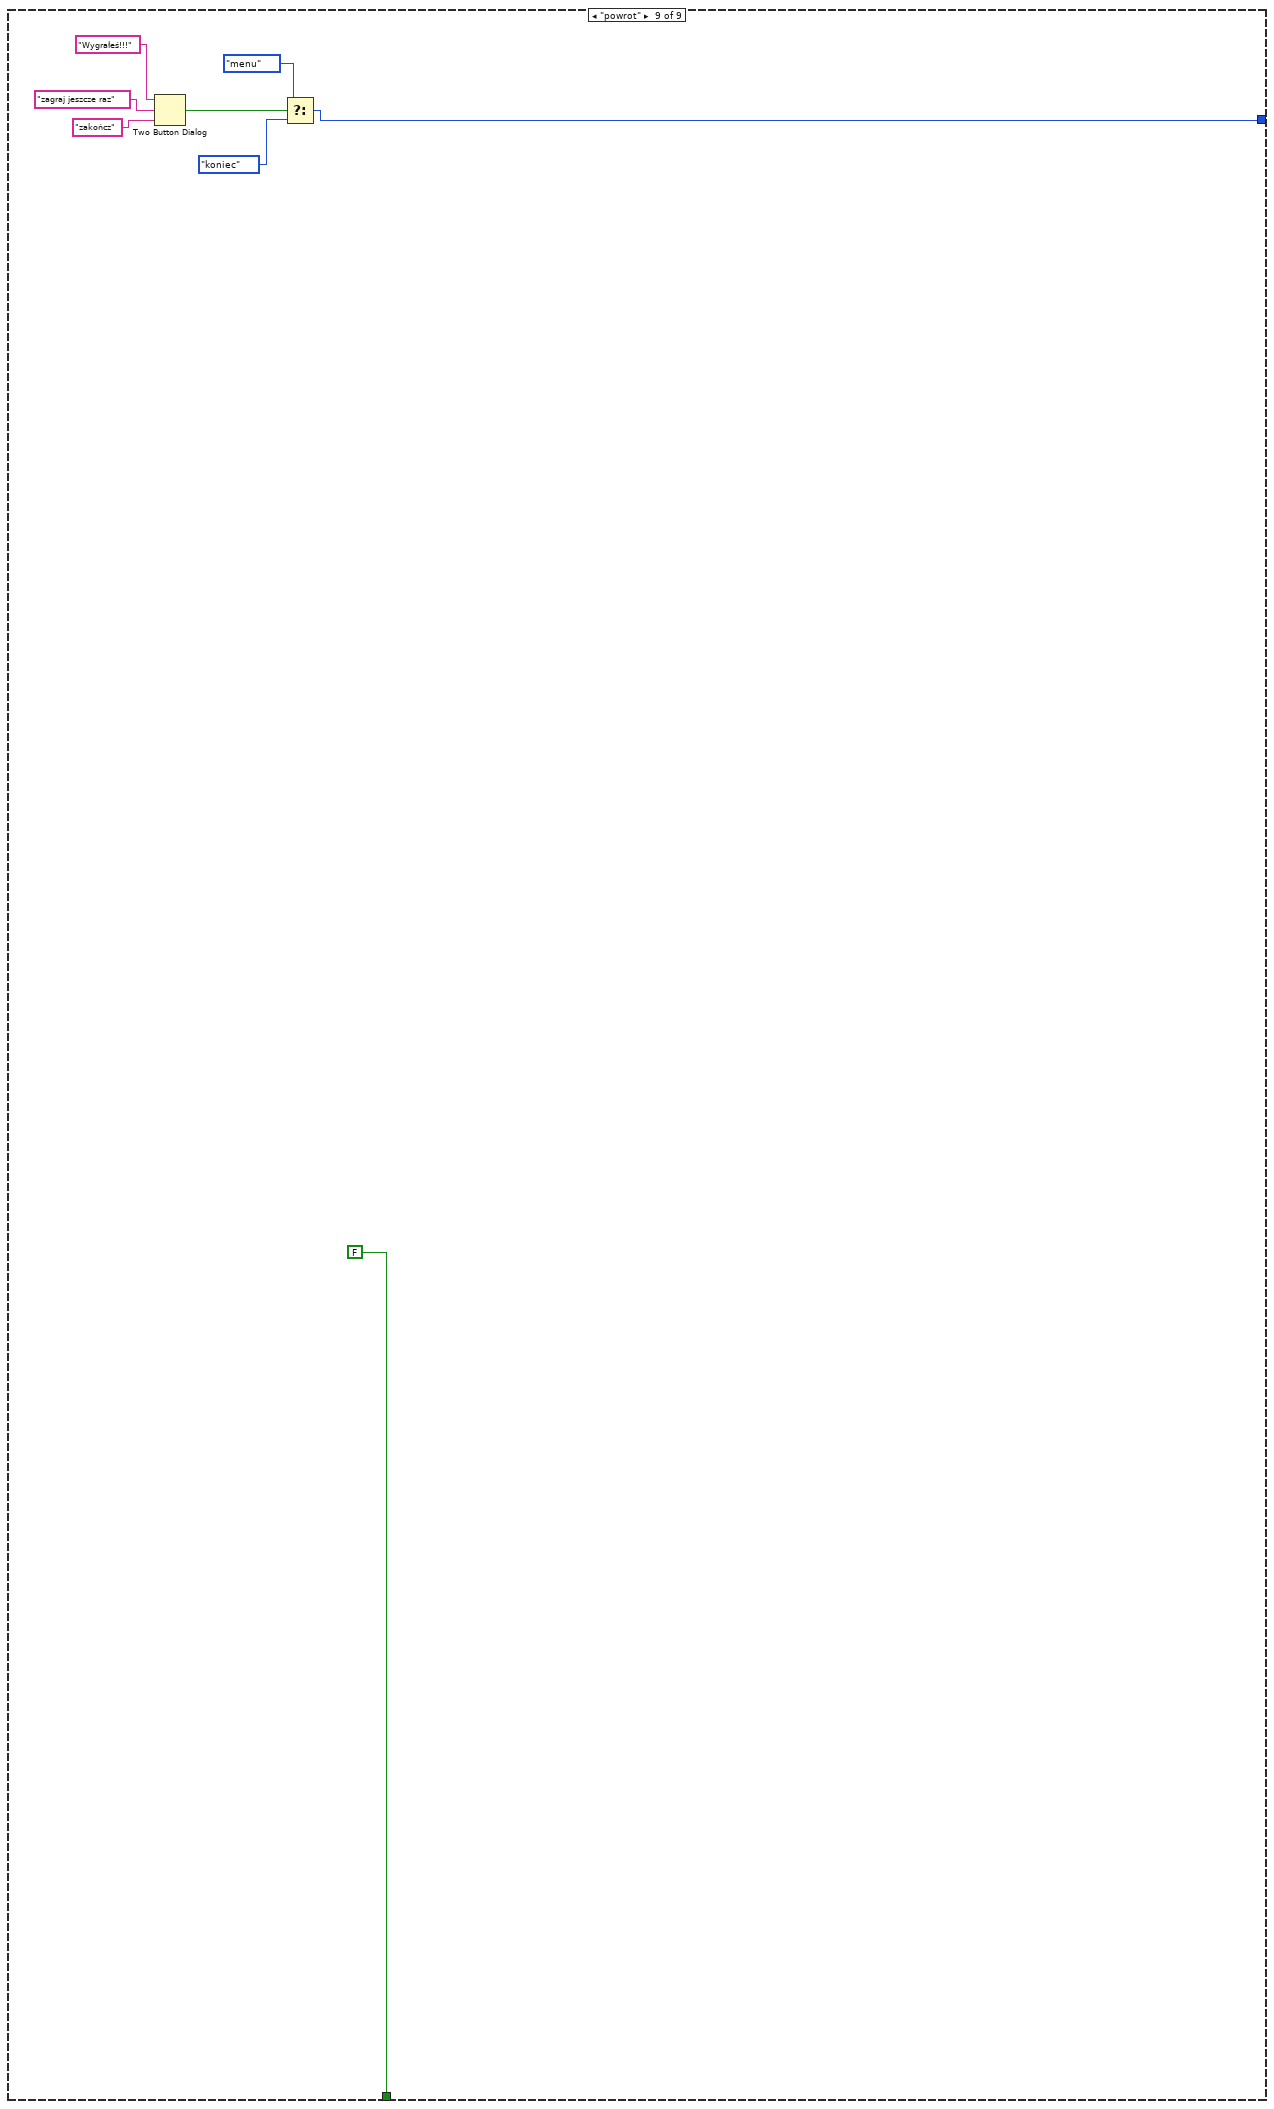
[diagram p13: hidden frame]
diagram:
  n1 = while {
    shift-right: [w3] -> _
    shift-left: T1."menu" -> [w4]
    stop <- w2 stop-if-true
    n2 = case shown="\"13x14\"" w4 {
      selector: w4 -> [_ _ _ _ _ _ _ w271 _]
      tunnel: [w13 w25 w33 w42 w119 w228 w247 w271 w273] -> w3
      tunnel: [FALSE FALSE FALSE FALSE FALSE FALSE FALSE TRUE FALSE] -> w2
      frame "menu" {
        w5 = FALSE ("Visible")
        w7 = FALSE ("Visible")
        w8 = FALSE ("Visible")
        w9 = FALSE ("Visible")
        w10 = FALSE ("Visible")
        w12 = FALSE
        w14 = FALSE
        w15 = FALSE
        w16 = FALSE
        n3 = property on="aOK Button 22" class="Bool (strict)"("Visible"=w5) -> ()  [unwired: 2 in, 2 out]
        n4 = property on="aOK Button 24" class="Bool (strict)"("Visible"=w5) -> ()  [unwired: 2 in, 2 out]
        n5 = property on="aOK Button 21" class="Bool (strict)"("Visible"=w5) -> ()  [unwired: 2 in, 2 out]
        n6 = property on="aOK Button 23" class="Bool (strict)"("Visible"=w5) -> ()  [unwired: 2 in, 2 out]
        n7 = property on="Boolean 11" class="Bool (strict)"("Visible"=w16) -> ()  [unwired: 2 in, 2 out]
        n8 = property on="OK Button 10" class="Bool (strict)"("Visible"=w16) -> ()  [unwired: 2 in, 2 out]
        n9 = property on="aOK Button 14" class="Bool (strict)"("Visible"=w5) -> ()  [unwired: 2 in, 2 out]
        n10 = property on="aOK Button 17" class="Bool (strict)"("Visible"=w5) -> ()  [unwired: 2 in, 2 out]
        n11 = property on="Boolean 12" class="Bool (strict)"("Visible"=w16) -> ()  [unwired: 2 in, 2 out]
        n12 = property on="Boolean 14" class="Bool (strict)"("Visible"=w16) -> ()  [unwired: 2 in, 2 out]
        n13 = property on="OK Button" class="Bool (strict)"("Visible"=w16) -> ()  [unwired: 2 in, 2 out]
        n14 = property on="aOK Button 13" class="Bool (strict)"("Visible"=w5) -> ()  [unwired: 2 in, 2 out]
        n15 = property on="aOK Button 15" class="Bool (strict)"("Visible"=w5) -> ()  [unwired: 2 in, 2 out]
        n16 = property on="Boolean 10" class="Bool (strict)"("Visible"=w16) -> ()  [unwired: 2 in, 2 out]
        n17 = property on="Boolean 13" class="Bool (strict)"("Visible"=w16) -> ()  [unwired: 2 in, 2 out]
        n18 = property on="aOK Button 19" class="Bool (strict)"("Visible"=w5) -> ()  [unwired: 2 in, 2 out]
        n19 = property on="aOK Button 20" class="Bool (strict)"("Visible"=w5) -> ()  [unwired: 2 in, 2 out]
        n20 = property on="aOK Button 18" class="Bool (strict)"("Visible"=w5) -> ()  [unwired: 2 in, 2 out]
        n21 = property on="aOK Button 2" class="Bool (strict)"("Visible"=w5) -> ()  [unwired: 2 in, 2 out]
        n22 = property on="aOK Button 68" class="Bool (strict)"("Value"=w5) -> ()  [unwired: 2 in, 2 out]
        n23 = property on="aOK Button" class="Bool (strict)"("Visible"=w5) -> ()  [unwired: 2 in, 2 out]
        n24 = property on="aOK Button 12" class="Bool (strict)"("Visible"=w5) -> ()  [unwired: 2 in, 2 out]
        n25 = property on="aOK Button 10" class="Bool (strict)"("Visible"=w5) -> ()  [unwired: 2 in, 2 out]
        n26 = property on="aOK Button 11" class="Bool (strict)"("Visible"=w5) -> ()  [unwired: 2 in, 2 out]
        n27 = property on="Boolean 11" class="Bool (strict)"("Value"=w12) -> ()  [unwired: 2 in, 2 out]
        n28 = property on="OK Button 10" class="Bool (strict)"("Value"=w12) -> ()  [unwired: 2 in, 2 out]
        n29 = property on="Boolean 12" class="Bool (strict)"("Value"=w12) -> ()  [unwired: 2 in, 2 out]
        n30 = property on="Boolean 14" class="Bool (strict)"("Value"=w12) -> ()  [unwired: 2 in, 2 out]
        n31 = property on="OK Button" class="Bool (strict)"("Value"=w12) -> ()  [unwired: 2 in, 2 out]
        n32 = property on="Boolean 10" class="Bool (strict)"("Value"=w12) -> ()  [unwired: 2 in, 2 out]
        n33 = property on="Boolean 13" class="Bool (strict)"("Value"=w12) -> ()  [unwired: 2 in, 2 out]
        n34 = property on="OK Button 11" class="Bool (strict)"("Visible"=w16) -> ()  [unwired: 2 in, 2 out]
        n35 = property on="aOK Button 37" class="Bool (strict)"("Visible"=w5) -> ()  [unwired: 2 in, 2 out]
        n36 = property on="aOK Button 38" class="Bool (strict)"("Visible"=w5) -> ()  [unwired: 2 in, 2 out]
        n37 = property on="aOK Button 36" class="Bool (strict)"("Visible"=w5) -> ()  [unwired: 2 in, 2 out]
        n38 = property on="aOK Button 39" class="Bool (strict)"("Visible"=w5) -> ()  [unwired: 2 in, 2 out]
        n39 = property on="OK Button 13" class="Bool (strict)"("Visible"=w16) -> ()  [unwired: 2 in, 2 out]
        n40 = property on="aOK Button 3" class="Bool (strict)"("Visible"=w5) -> ()  [unwired: 2 in, 2 out]
        n41 = property on="aOK Button 31" class="Bool (strict)"("Visible"=w5) -> ()  [unwired: 2 in, 2 out]
        n42 = property on="aOK Button 69" class="Bool (strict)"("Value"=w5) -> ()  [unwired: 2 in, 2 out]
        n43 = property on="aOK Button 29" class="Bool (strict)"("Visible"=w5) -> ()  [unwired: 2 in, 2 out]
        n44 = property on="aOK Button 30" class="Bool (strict)"("Visible"=w5) -> ()  [unwired: 2 in, 2 out]
        n45 = property on="Boolean 16" class="Bool (strict)"("Visible"=w16) -> ()  [unwired: 2 in, 2 out]
        n46 = property on="aOK Button 33" class="Bool (strict)"("Visible"=w5) -> ()  [unwired: 2 in, 2 out]
        n47 = property on="aOK Button 35" class="Bool (strict)"("Visible"=w5) -> ()  [unwired: 2 in, 2 out]
        n48 = property on="Boolean 17" class="Bool (strict)"("Visible"=w16) -> ()  [unwired: 2 in, 2 out]
        n49 = property on="Boolean 19" class="Bool (strict)"("Visible"=w16) -> ()  [unwired: 2 in, 2 out]
        n50 = property on="aOK Button 32" class="Bool (strict)"("Visible"=w5) -> ()  [unwired: 2 in, 2 out]
        n51 = property on="aOK Button 34" class="Bool (strict)"("Visible"=w5) -> ()  [unwired: 2 in, 2 out]
        n52 = property on="Boolean 15" class="Bool (strict)"("Visible"=w16) -> ()  [unwired: 2 in, 2 out]
        n53 = property on="Boolean 18" class="Bool (strict)"("Visible"=w16) -> ()  [unwired: 2 in, 2 out]
        n54 = property on="aOK Button 26" class="Bool (strict)"("Visible"=w5) -> ()  [unwired: 2 in, 2 out]
        n55 = property on="aOK Button 28" class="Bool (strict)"("Visible"=w5) -> ()  [unwired: 2 in, 2 out]
        n56 = property on="aOK Button 25" class="Bool (strict)"("Visible"=w5) -> ()  [unwired: 2 in, 2 out]
        n57 = property on="aOK Button 27" class="Bool (strict)"("Visible"=w5) -> ()  [unwired: 2 in, 2 out]
        n58 = property on="OK Button 11" class="Bool (strict)"("Value"=w12) -> ()  [unwired: 2 in, 2 out]
        n59 = property on="OK Button 13" class="Bool (strict)"("Value"=w12) -> ()  [unwired: 2 in, 2 out]
        n60 = property on="Boolean 16" class="Bool (strict)"("Value"=w12) -> ()  [unwired: 2 in, 2 out]
        n61 = property on="Boolean 17" class="Bool (strict)"("Value"=w12) -> ()  [unwired: 2 in, 2 out]
        n62 = property on="Boolean 19" class="Bool (strict)"("Value"=w12) -> ()  [unwired: 2 in, 2 out]
        n63 = property on="Boolean 15" class="Bool (strict)"("Value"=w12) -> ()  [unwired: 2 in, 2 out]
        n64 = property on="Boolean 18" class="Bool (strict)"("Value"=w12) -> ()  [unwired: 2 in, 2 out]
        n65 = property on="OK Button 12" class="Bool (strict)"("Visible"=w16) -> ()  [unwired: 2 in, 2 out]
        n66 = property on="OK Button 14" class="Bool (strict)"("Visible"=w16) -> ()  [unwired: 2 in, 2 out]
        n67 = property on="aOK Button 52" class="Bool (strict)"("Visible"=w5) -> ()  [unwired: 2 in, 2 out]
        n68 = property on="aOK Button 54" class="Bool (strict)"("Visible"=w5) -> ()  [unwired: 2 in, 2 out]
        n69 = property on="aOK Button 7" class="Bool (strict)"("Value"=w5) -> ()  [unwired: 2 in, 2 out]
        n70 = property on="aOK Button 51" class="Bool (strict)"("Visible"=w5) -> ()  [unwired: 2 in, 2 out]
        n71 = property on="aOK Button 53" class="Bool (strict)"("Visible"=w5) -> ()  [unwired: 2 in, 2 out]
        n72 = property on="aOK Button 45" class="Bool (strict)"("Visible"=w5) -> ()  [unwired: 2 in, 2 out]
        n73 = property on="aOK Button 47" class="Bool (strict)"("Visible"=w5) -> ()  [unwired: 2 in, 2 out]
        n74 = property on="aOK Button 44" class="Bool (strict)"("Visible"=w5) -> ()  [unwired: 2 in, 2 out]
        n75 = property on="aOK Button 46" class="Bool (strict)"("Visible"=w5) -> ()  [unwired: 2 in, 2 out]
        n76 = property on="aOK Button 49" class="Bool (strict)"("Visible"=w5) -> ()  [unwired: 2 in, 2 out]
        n77 = property on="aOK Button 50" class="Bool (strict)"("Visible"=w5) -> ()  [unwired: 2 in, 2 out]
        n78 = property on="aOK Button 48" class="Bool (strict)"("Visible"=w5) -> ()  [unwired: 2 in, 2 out]
        n79 = property on="aOK Button 5" class="Bool (strict)"("Visible"=w5) -> ()  [unwired: 2 in, 2 out]
        n80 = Two Button Dialog(message="wybierz poziom trudności", 1:"trudny" ("message"), 2:"łatwy" ("message")) -> (T button?=w20:bool)
        n81 = property on="aOK Button 40" class="Bool (strict)"("Visible"=w5) -> ()  [unwired: 2 in, 2 out]
        n82 = property on="aOK Button 42" class="Bool (strict)"("Visible"=w5) -> ()  [unwired: 2 in, 2 out]
        n83 = property on="aOK Button 4" class="Bool (strict)"("Visible"=w5) -> ()  [unwired: 2 in, 2 out]
        n84 = property on="aOK Button 41" class="Bool (strict)"("Visible"=w5) -> ()  [unwired: 2 in, 2 out]
        n85 = property on="Boolean 20" class="Bool (strict)"("Visible"=w16) -> ()  [unwired: 2 in, 2 out]
        n86 = property on="Boolean 21" class="Bool (strict)"("Visible"=w16) -> ()  [unwired: 2 in, 2 out]
        n87 = property on="Boolean 23" class="Bool (strict)"("Visible"=w16) -> ()  [unwired: 2 in, 2 out]
        n88 = property on="Boolean 2" class="Bool (strict)"("Visible"=w16) -> ()  [unwired: 2 in, 2 out]
        n89 = property on="Boolean 22" class="Bool (strict)"("Visible"=w16) -> ()  [unwired: 2 in, 2 out]
        n90 = property on="OK Button 12" class="Bool (strict)"("Value"=w12) -> ()  [unwired: 2 in, 2 out]
        n91 = property on="OK Button 14" class="Bool (strict)"("Value"=w12) -> ()  [unwired: 2 in, 2 out]
        n92 = property on="Boolean 20" class="Bool (strict)"("Value"=w12) -> ()  [unwired: 2 in, 2 out]
        n93 = property on="Boolean 21" class="Bool (strict)"("Value"=w12) -> ()  [unwired: 2 in, 2 out]
        n94 = property on="Boolean 23" class="Bool (strict)"("Value"=w12) -> ()  [unwired: 2 in, 2 out]
        n95 = property on="Boolean 2" class="Bool (strict)"("Value"=w12) -> ()  [unwired: 2 in, 2 out]
        n96 = property on="Boolean 22" class="Bool (strict)"("Value"=w12) -> ()  [unwired: 2 in, 2 out]
        n97 = property on="OK Button 16" class="Bool (strict)"("Visible"=w16) -> ()  [unwired: 2 in, 2 out]
        n98 = property on="OK Button 15" class="Bool (strict)"("Visible"=w16) -> ()  [unwired: 2 in, 2 out]
        n99 = property on="aOK Button 68" class="Bool (strict)"("Visible"=w5) -> ()  [unwired: 2 in, 2 out]
        n100 = property on="aOK Button 7" class="Bool (strict)"("Visible"=w5) -> ()  [unwired: 2 in, 2 out]
        n101 = property on="aOK Button 67" class="Bool (strict)"("Visible"=w5) -> ()  [unwired: 2 in, 2 out]
        n102 = property on="aOK Button 69" class="Bool (strict)"("Visible"=w5) -> ()  [unwired: 2 in, 2 out]
        n103 = property on="aOK Button 60" class="Bool (strict)"("Visible"=w5) -> ()  [unwired: 2 in, 2 out]
        n104 = property on="aOK Button 62" class="Bool (strict)"("Visible"=w5) -> ()  [unwired: 2 in, 2 out]
        n105 = property on="aOK Button 6" class="Bool (strict)"("Visible"=w5) -> ()  [unwired: 2 in, 2 out]
        n106 = property on="aOK Button 61" class="Bool (strict)"("Visible"=w5) -> ()  [unwired: 2 in, 2 out]
        n107 = property on="aOK Button 64" class="Bool (strict)"("Visible"=w5) -> ()  [unwired: 2 in, 2 out]
        n108 = property on="aOK Button 66" class="Bool (strict)"("Visible"=w5) -> ()  [unwired: 2 in, 2 out]
        n109 = property on="aOK Button 63" class="Bool (strict)"("Visible"=w5) -> ()  [unwired: 2 in, 2 out]
        n110 = property on="aOK Button 65" class="Bool (strict)"("Visible"=w5) -> ()  [unwired: 2 in, 2 out]
        n111 = property on="aOK Button 56" class="Bool (strict)"("Visible"=w5) -> ()  [unwired: 2 in, 2 out]
        n112 = property on="aOK Button 59" class="Bool (strict)"("Visible"=w5) -> ()  [unwired: 2 in, 2 out]
        n113 = property on="aOK Button 55" class="Bool (strict)"("Visible"=w5) -> ()  [unwired: 2 in, 2 out]
        n114 = property on="aOK Button 58" class="Bool (strict)"("Visible"=w5) -> ()  [unwired: 2 in, 2 out]
        n115 = property on="Boolean 25" class="Bool (strict)"("Visible"=w16) -> ()  [unwired: 2 in, 2 out]
        n116 = property on="Boolean 26" class="Bool (strict)"("Visible"=w16) -> ()  [unwired: 2 in, 2 out]
        n117 = property on="Boolean 28" class="Bool (strict)"("Visible"=w16) -> ()  [unwired: 2 in, 2 out]
        n118 = property on="Boolean 24" class="Bool (strict)"("Visible"=w16) -> ()  [unwired: 2 in, 2 out]
        n119 = property on="Boolean 27" class="Bool (strict)"("Visible"=w16) -> ()  [unwired: 2 in, 2 out]
        n120 = Select(t=T2."latwy", s=w20, f=T2."trudny") -> (s? t:f=w13:T2)
        n121 = property on="OK Button 16" class="Bool (strict)"("Value"=w12) -> ()  [unwired: 2 in, 2 out]
        n122 = property on="OK Button 15" class="Bool (strict)"("Value"=w12) -> ()  [unwired: 2 in, 2 out]
        n123 = property on="Boolean 25" class="Bool (strict)"("Value"=w12) -> ()  [unwired: 2 in, 2 out]
        n124 = property on="Boolean 26" class="Bool (strict)"("Value"=w12) -> ()  [unwired: 2 in, 2 out]
        n125 = property on="Boolean 28" class="Bool (strict)"("Value"=w12) -> ()  [unwired: 2 in, 2 out]
        n126 = property on="Boolean 24" class="Bool (strict)"("Value"=w12) -> ()  [unwired: 2 in, 2 out]
        n127 = property on="Boolean 27" class="Bool (strict)"("Value"=w12) -> ()  [unwired: 2 in, 2 out]
        n128 = property on="aOK Button 75" class="Bool (strict)"("Value"=w5) -> ()  [unwired: 2 in, 2 out]
        n129 = property on="aOK Button 9" class="Bool (strict)"("Value"=w5) -> ()  [unwired: 2 in, 2 out]
        n130 = property on="OK Button 3" class="Bool (strict)"("Visible"=w16) -> ()  [unwired: 2 in, 2 out]
        n131 = property on="aOK Button 74" class="Bool (strict)"("Value"=w5) -> ()  [unwired: 2 in, 2 out]
        n132 = property on="aOK Button 8" class="Bool (strict)"("Value"=w5) -> ()  [unwired: 2 in, 2 out]
        n133 = property on="OK Button 2" class="Bool (strict)"("Visible"=w16) -> ()  [unwired: 2 in, 2 out]
        n134 = property on="aOK Button 75" class="Bool (strict)"("Visible"=w5) -> ()  [unwired: 2 in, 2 out]
        n135 = property on="aOK Button 9" class="Bool (strict)"("Visible"=w5) -> ()  [unwired: 2 in, 2 out]
        n136 = property on="aOK Button 74" class="Bool (strict)"("Visible"=w5) -> ()  [unwired: 2 in, 2 out]
        n137 = property on="aOK Button 8" class="Bool (strict)"("Visible"=w5) -> ()  [unwired: 2 in, 2 out]
        n138 = property on="aOK Button 71" class="Bool (strict)"("Value"=w5) -> ()  [unwired: 2 in, 2 out]
        n139 = property on="aOK Button 73" class="Bool (strict)"("Value"=w5) -> ()  [unwired: 2 in, 2 out]
        n140 = property on="aOK Button 70" class="Bool (strict)"("Value"=w5) -> ()  [unwired: 2 in, 2 out]
        n141 = property on="aOK Button 72" class="Bool (strict)"("Value"=w5) -> ()  [unwired: 2 in, 2 out]
        n142 = property on="aOK Button 71" class="Bool (strict)"("Visible"=w5) -> ()  [unwired: 2 in, 2 out]
        n143 = property on="aOK Button 73" class="Bool (strict)"("Visible"=w5) -> ()  [unwired: 2 in, 2 out]
        n144 = property on="aOK Button 70" class="Bool (strict)"("Visible"=w5) -> ()  [unwired: 2 in, 2 out]
        n145 = property on="aOK Button 72" class="Bool (strict)"("Visible"=w5) -> ()  [unwired: 2 in, 2 out]
        n146 = property on="Boolean 3" class="Bool (strict)"("Visible"=w16) -> ()  [unwired: 2 in, 2 out]
        n147 = property on="Boolean 30" class="Bool (strict)"("Visible"=w16) -> ()  [unwired: 2 in, 2 out]
        n148 = property on="Boolean 32" class="Bool (strict)"("Visible"=w16) -> ()  [unwired: 2 in, 2 out]
        n149 = property on="Boolean 29" class="Bool (strict)"("Visible"=w16) -> ()  [unwired: 2 in, 2 out]
        n150 = property on="Boolean 31" class="Bool (strict)"("Visible"=w16) -> ()  [unwired: 2 in, 2 out]
        n151 = property on="OK Button 3" class="Bool (strict)"("Value"=w12) -> ()  [unwired: 2 in, 2 out]
        n152 = property on="OK Button 2" class="Bool (strict)"("Value"=w12) -> ()  [unwired: 2 in, 2 out]
        n153 = property on="Boolean 3" class="Bool (strict)"("Value"=w12) -> ()  [unwired: 2 in, 2 out]
        n154 = property on="Boolean 30" class="Bool (strict)"("Value"=w12) -> ()  [unwired: 2 in, 2 out]
        n155 = property on="Boolean 32" class="Bool (strict)"("Value"=w12) -> ()  [unwired: 2 in, 2 out]
        n156 = property on="Boolean 29" class="Bool (strict)"("Value"=w12) -> ()  [unwired: 2 in, 2 out]
        n157 = property on="Boolean 31" class="Bool (strict)"("Value"=w12) -> ()  [unwired: 2 in, 2 out]
        n158 = property on="OK Button 5" class="Bool (strict)"("Visible"=w16) -> ()  [unwired: 2 in, 2 out]
        n159 = property on="OK Button 4" class="Bool (strict)"("Visible"=w16) -> ()  [unwired: 2 in, 2 out]
        n160 = property on="aOK Button 22" class="Bool (strict)"("Value"=w5) -> ()  [unwired: 2 in, 2 out]
        n161 = property on="aOK Button 24" class="Bool (strict)"("Value"=w5) -> ()  [unwired: 2 in, 2 out]
        n162 = property on="aOK Button 21" class="Bool (strict)"("Value"=w5) -> ()  [unwired: 2 in, 2 out]
        n163 = property on="aOK Button 23" class="Bool (strict)"("Value"=w5) -> ()  [unwired: 2 in, 2 out]
        n164 = property on="aOK Button 14" class="Bool (strict)"("Value"=w5) -> ()  [unwired: 2 in, 2 out]
        n165 = property on="aOK Button 17" class="Bool (strict)"("Value"=w5) -> ()  [unwired: 2 in, 2 out]
        n166 = property on="aOK Button 13" class="Bool (strict)"("Value"=w5) -> ()  [unwired: 2 in, 2 out]
        n167 = property on="aOK Button 15" class="Bool (strict)"("Value"=w5) -> ()  [unwired: 2 in, 2 out]
        n168 = property on="aOK Button 19" class="Bool (strict)"("Value"=w5) -> ()  [unwired: 2 in, 2 out]
        n169 = property on="aOK Button 20" class="Bool (strict)"("Value"=w5) -> ()  [unwired: 2 in, 2 out]
        n170 = property on="aOK Button 18" class="Bool (strict)"("Value"=w5) -> ()  [unwired: 2 in, 2 out]
        n171 = property on="aOK Button 2" class="Bool (strict)"("Value"=w5) -> ()  [unwired: 2 in, 2 out]
        n172 = property on="aOK Button" class="Bool (strict)"("Value"=w5) -> ()  [unwired: 2 in, 2 out]
        n173 = property on="aOK Button 12" class="Bool (strict)"("Value"=w5) -> ()  [unwired: 2 in, 2 out]
        n174 = property on="aOK Button 10" class="Bool (strict)"("Value"=w5) -> ()  [unwired: 2 in, 2 out]
        n175 = property on="aOK Button 11" class="Bool (strict)"("Value"=w5) -> ()  [unwired: 2 in, 2 out]
        n176 = property on="Boolean 34" class="Bool (strict)"("Visible"=w16) -> ()  [unwired: 2 in, 2 out]
        n177 = property on="Boolean 35" class="Bool (strict)"("Visible"=w16) -> ()  [unwired: 2 in, 2 out]
        n178 = property on="Boolean 37" class="Bool (strict)"("Visible"=w16) -> ()  [unwired: 2 in, 2 out]
        n179 = property on="Boolean 33" class="Bool (strict)"("Visible"=w16) -> ()  [unwired: 2 in, 2 out]
        n180 = property on="Boolean 36" class="Bool (strict)"("Visible"=w16) -> ()  [unwired: 2 in, 2 out]
        n181 = property on="OK Button 5" class="Bool (strict)"("Value"=w12) -> ()  [unwired: 2 in, 2 out]
        n182 = property on="OK Button 4" class="Bool (strict)"("Value"=w12) -> ()  [unwired: 2 in, 2 out]
        n183 = property on="Boolean 34" class="Bool (strict)"("Value"=w12) -> ()  [unwired: 2 in, 2 out]
        n184 = property on="Boolean 35" class="Bool (strict)"("Value"=w12) -> ()  [unwired: 2 in, 2 out]
        n185 = property on="Boolean 37" class="Bool (strict)"("Value"=w12) -> ()  [unwired: 2 in, 2 out]
        n186 = property on="Boolean 33" class="Bool (strict)"("Value"=w12) -> ()  [unwired: 2 in, 2 out]
        n187 = property on="Boolean 36" class="Bool (strict)"("Value"=w12) -> ()  [unwired: 2 in, 2 out]
        n188 = property on="aOK Button 37" class="Bool (strict)"("Value"=w5) -> ()  [unwired: 2 in, 2 out]
        n189 = property on="aOK Button 38" class="Bool (strict)"("Value"=w5) -> ()  [unwired: 2 in, 2 out]
        n190 = property on="aOK Button 36" class="Bool (strict)"("Value"=w5) -> ()  [unwired: 2 in, 2 out]
        n191 = property on="aOK Button 39" class="Bool (strict)"("Value"=w5) -> ()  [unwired: 2 in, 2 out]
        n192 = property on="OK Button 7" class="Bool (strict)"("Visible"=w16) -> ()  [unwired: 2 in, 2 out]
        n193 = property on="aOK Button 3" class="Bool (strict)"("Value"=w5) -> ()  [unwired: 2 in, 2 out]
        n194 = property on="aOK Button 31" class="Bool (strict)"("Value"=w5) -> ()  [unwired: 2 in, 2 out]
        n195 = property on="OK Button 6" class="Bool (strict)"("Visible"=w16) -> ()  [unwired: 2 in, 2 out]
        n196 = property on="aOK Button 29" class="Bool (strict)"("Value"=w5) -> ()  [unwired: 2 in, 2 out]
        n197 = property on="aOK Button 30" class="Bool (strict)"("Value"=w5) -> ()  [unwired: 2 in, 2 out]
        n198 = property on="aOK Button 33" class="Bool (strict)"("Value"=w5) -> ()  [unwired: 2 in, 2 out]
        n199 = property on="aOK Button 35" class="Bool (strict)"("Value"=w5) -> ()  [unwired: 2 in, 2 out]
        n200 = property on="aOK Button 32" class="Bool (strict)"("Value"=w5) -> ()  [unwired: 2 in, 2 out]
        n201 = property on="aOK Button 34" class="Bool (strict)"("Value"=w5) -> ()  [unwired: 2 in, 2 out]
        n202 = property on="aOK Button 26" class="Bool (strict)"("Value"=w5) -> ()  [unwired: 2 in, 2 out]
        n203 = property on="aOK Button 28" class="Bool (strict)"("Value"=w5) -> ()  [unwired: 2 in, 2 out]
        n204 = property on="aOK Button 25" class="Bool (strict)"("Value"=w5) -> ()  [unwired: 2 in, 2 out]
        n205 = property on="aOK Button 27" class="Bool (strict)"("Value"=w5) -> ()  [unwired: 2 in, 2 out]
        n206 = property on="Boolean 39" class="Bool (strict)"("Visible"=w16) -> ()  [unwired: 2 in, 2 out]
        n207 = property on="Boolean 4" class="Bool (strict)"("Visible"=w16) -> ()  [unwired: 2 in, 2 out]
        n208 = property on="Boolean 9" class="Bool (strict)"("Visible"=w16) -> ()  [unwired: 2 in, 2 out]
        n209 = property on="Boolean 38" class="Bool (strict)"("Visible"=w16) -> ()  [unwired: 2 in, 2 out]
        n210 = property on="Boolean 40" class="Bool (strict)"("Visible"=w16) -> ()  [unwired: 2 in, 2 out]
        n211 = property on="OK Button 7" class="Bool (strict)"("Value"=w12) -> ()  [unwired: 2 in, 2 out]
        n212 = property on="OK Button 6" class="Bool (strict)"("Value"=w12) -> ()  [unwired: 2 in, 2 out]
        n213 = property on="Boolean 39" class="Bool (strict)"("Value"=w12) -> ()  [unwired: 2 in, 2 out]
        n214 = property on="Boolean 4" class="Bool (strict)"("Value"=w12) -> ()  [unwired: 2 in, 2 out]
        n215 = property on="Boolean 9" class="Bool (strict)"("Value"=w12) -> ()  [unwired: 2 in, 2 out]
        n216 = property on="Boolean 38" class="Bool (strict)"("Value"=w12) -> ()  [unwired: 2 in, 2 out]
        n217 = property on="Boolean 40" class="Bool (strict)"("Value"=w12) -> ()  [unwired: 2 in, 2 out]
        n218 = property on="aOK Button 52" class="Bool (strict)"("Value"=w5) -> ()  [unwired: 2 in, 2 out]
        n219 = property on="aOK Button 54" class="Bool (strict)"("Value"=w5) -> ()  [unwired: 2 in, 2 out]
        n220 = property on="aOK Button 51" class="Bool (strict)"("Value"=w5) -> ()  [unwired: 2 in, 2 out]
        n221 = property on="aOK Button 53" class="Bool (strict)"("Value"=w5) -> ()  [unwired: 2 in, 2 out]
        n222 = property on="aOK Button 45" class="Bool (strict)"("Value"=w5) -> ()  [unwired: 2 in, 2 out]
        n223 = property on="aOK Button 47" class="Bool (strict)"("Value"=w5) -> ()  [unwired: 2 in, 2 out]
        n224 = property on="aOK Button 44" class="Bool (strict)"("Value"=w5) -> ()  [unwired: 2 in, 2 out]
        n225 = property on="aOK Button 46" class="Bool (strict)"("Value"=w5) -> ()  [unwired: 2 in, 2 out]
        n226 = property on="aOK Button 49" class="Bool (strict)"("Value"=w5) -> ()  [unwired: 2 in, 2 out]
        n227 = property on="aOK Button 50" class="Bool (strict)"("Value"=w5) -> ()  [unwired: 2 in, 2 out]
        n228 = property on="aOK Button 48" class="Bool (strict)"("Value"=w5) -> ()  [unwired: 2 in, 2 out]
        n229 = property on="aOK Button 5" class="Bool (strict)"("Value"=w5) -> ()  [unwired: 2 in, 2 out]
        n230 = property on="aOK Button 40" class="Bool (strict)"("Value"=w5) -> ()  [unwired: 2 in, 2 out]
        n231 = property on="aOK Button 42" class="Bool (strict)"("Value"=w5) -> ()  [unwired: 2 in, 2 out]
        n232 = property on="aOK Button 4" class="Bool (strict)"("Value"=w5) -> ()  [unwired: 2 in, 2 out]
        n233 = property on="aOK Button 41" class="Bool (strict)"("Value"=w5) -> ()  [unwired: 2 in, 2 out]
        n234 = property on="OK Button 9" class="Bool (strict)"("Visible"=w16) -> ()  [unwired: 2 in, 2 out]
        n235 = property on="OK Button 8" class="Bool (strict)"("Visible"=w16) -> ()  [unwired: 2 in, 2 out]
        n236 = property on="Boolean 5" class="Bool (strict)"("Visible"=w16) -> ()  [unwired: 2 in, 2 out]
        n237 = property on="Boolean 6" class="Bool (strict)"("Visible"=w16) -> ()  [unwired: 2 in, 2 out]
        n238 = property on="Boolean 8" class="Bool (strict)"("Visible"=w16) -> ()  [unwired: 2 in, 2 out]
        n239 = property on="Boolean 42" class="Bool (strict)"("Visible"=w16) -> ()  [unwired: 2 in, 2 out]
        n240 = property on="Boolean 7" class="Bool (strict)"("Visible"=w16) -> ()  [unwired: 2 in, 2 out]
        n241 = property on="Boolean 43" class="Bool (strict)"("Visible"=w16) -> ()  [unwired: 2 in, 2 out]
        n242 = property on="OK Button 82" class="Bool (strict)"("Visible"=w9) -> ()  [unwired: 2 in, 2 out]
        n243 = property on="OK Button 78" class="Bool (strict)"("Visible"=w9) -> ()  [unwired: 2 in, 2 out]
        n244 = property on="OK Button 143" class="Bool (strict)"("Visible"=w9) -> ()  [unwired: 2 in, 2 out]
        n245 = property on="OK Button 131" class="Bool (strict)"("Visible"=w9) -> ()  [unwired: 2 in, 2 out]
        n246 = property on="OK Button 144" class="Bool (strict)"("Visible"=w9) -> ()  [unwired: 2 in, 2 out]
        n247 = property on="OK Button 162" class="Bool (strict)"("Visible"=w9) -> ()  [unwired: 2 in, 2 out]
        n248 = property on="OK Button 154" class="Bool (strict)"("Visible"=w9) -> ()  [unwired: 2 in, 2 out]
        n249 = property on="OK Button 81" class="Bool (strict)"("Visible"=w9) -> ()  [unwired: 2 in, 2 out]
        n250 = property on="OK Button 83" class="Bool (strict)"("Visible"=w9) -> ()  [unwired: 2 in, 2 out]
        n251 = property on="OK Button 9" class="Bool (strict)"("Value"=w12) -> ()  [unwired: 2 in, 2 out]
        n252 = property on="OK Button 77" class="Bool (strict)"("Visible"=w9) -> ()  [unwired: 2 in, 2 out]
        n253 = property on="OK Button 80" class="Bool (strict)"("Visible"=w9) -> ()  [unwired: 2 in, 2 out]
        n254 = property on="OK Button 8" class="Bool (strict)"("Value"=w12) -> ()  [unwired: 2 in, 2 out]
        n255 = property on="OK Button 124" class="Bool (strict)"("Visible"=w9) -> ()  [unwired: 2 in, 2 out]
        n256 = property on="OK Button 79" class="Bool (strict)"("Visible"=w9) -> ()  [unwired: 2 in, 2 out]
        n257 = property on="OK Button 136" class="Bool (strict)"("Visible"=w9) -> ()  [unwired: 2 in, 2 out]
        n258 = property on="Boolean 5" class="Bool (strict)"("Value"=w12) -> ()  [unwired: 2 in, 2 out]
        n259 = property on="Boolean 6" class="Bool (strict)"("Value"=w12) -> ()  [unwired: 2 in, 2 out]
        n260 = property on="Boolean 8" class="Bool (strict)"("Value"=w12) -> ()  [unwired: 2 in, 2 out]
        n261 = property on="Boolean 42" class="Bool (strict)"("Value"=w12) -> ()  [unwired: 2 in, 2 out]
        n262 = property on="Boolean 7" class="Bool (strict)"("Value"=w12) -> ()  [unwired: 2 in, 2 out]
        n263 = property on="aOK Button 67" class="Bool (strict)"("Value"=w5) -> ()  [unwired: 2 in, 2 out]
        n264 = property on="aOK Button 60" class="Bool (strict)"("Value"=w5) -> ()  [unwired: 2 in, 2 out]
        n265 = property on="aOK Button 62" class="Bool (strict)"("Value"=w5) -> ()  [unwired: 2 in, 2 out]
        n266 = property on="aOK Button 6" class="Bool (strict)"("Value"=w5) -> ()  [unwired: 2 in, 2 out]
        n267 = property on="aOK Button 61" class="Bool (strict)"("Value"=w5) -> ()  [unwired: 2 in, 2 out]
        n268 = property on="Boolean 43" class="Bool (strict)"("Value"=w12) -> ()  [unwired: 2 in, 2 out]
        n269 = property on="aOK Button 64" class="Bool (strict)"("Value"=w5) -> ()  [unwired: 2 in, 2 out]
        n270 = property on="aOK Button 66" class="Bool (strict)"("Value"=w5) -> ()  [unwired: 2 in, 2 out]
        n271 = property on="aOK Button 63" class="Bool (strict)"("Value"=w5) -> ()  [unwired: 2 in, 2 out]
        n272 = property on="aOK Button 65" class="Bool (strict)"("Value"=w5) -> ()  [unwired: 2 in, 2 out]
        n273 = property on="aOK Button 56" class="Bool (strict)"("Value"=w5) -> ()  [unwired: 2 in, 2 out]
        n274 = property on="aOK Button 59" class="Bool (strict)"("Value"=w5) -> ()  [unwired: 2 in, 2 out]
        n275 = property on="aOK Button 55" class="Bool (strict)"("Value"=w5) -> ()  [unwired: 2 in, 2 out]
        n276 = property on="aOK Button 58" class="Bool (strict)"("Value"=w5) -> ()  [unwired: 2 in, 2 out]
        n277 = property on="OK Button 110" class="Bool (strict)"("Visible"=w9) -> ()  [unwired: 2 in, 2 out]
        n278 = property on="OK Button 111" class="Bool (strict)"("Visible"=w9) -> ()  [unwired: 2 in, 2 out]
        n279 = property on="OK Button 96" class="Bool (strict)"("Visible"=w9) -> ()  [unwired: 2 in, 2 out]
        n280 = property on="OK Button 92" class="Bool (strict)"("Visible"=w9) -> ()  [unwired: 2 in, 2 out]
        n281 = property on="OK Button 95" class="Bool (strict)"("Visible"=w9) -> ()  [unwired: 2 in, 2 out]
        n282 = property on="OK Button 93" class="Bool (strict)"("Visible"=w9) -> ()  [unwired: 2 in, 2 out]
        n283 = property on="OK Button 97" class="Bool (strict)"("Visible"=w9) -> ()  [unwired: 2 in, 2 out]
        n284 = property on="OK Button 132" class="Bool (strict)"("Visible"=w9) -> ()  [unwired: 2 in, 2 out]
        n285 = property on="OK Button 148" class="Bool (strict)"("Visible"=w9) -> ()  [unwired: 2 in, 2 out]
        n286 = property on="OK Button 163" class="Bool (strict)"("Visible"=w9) -> ()  [unwired: 2 in, 2 out]
        n287 = property on="OK Button 155" class="Bool (strict)"("Visible"=w9) -> ()  [unwired: 2 in, 2 out]
        n288 = property on="OK Button 137" class="Bool (strict)"("Visible"=w9) -> ()  [unwired: 2 in, 2 out]
        n289 = property on="OK Button 165" class="Bool (strict)"("Visible"=w9) -> ()  [unwired: 2 in, 2 out]
        n290 = property on="OK Button 125" class="Bool (strict)"("Visible"=w9) -> ()  [unwired: 2 in, 2 out]
        n291 = property on="OK Button 112" class="Bool (strict)"("Visible"=w9) -> ()  [unwired: 2 in, 2 out]
        n292 = property on="Boolean 100" class="Bool (strict)"("Visible"=w15) -> ()  [unwired: 2 in, 2 out]
        n293 = property on="Boolean 101" class="Bool (strict)"("Visible"=w15) -> ()  [unwired: 2 in, 2 out]
        n294 = property on="Boolean 102" class="Bool (strict)"("Visible"=w15) -> ()  [unwired: 2 in, 2 out]
        n295 = property on="Boolean 103" class="Bool (strict)"("Visible"=w15) -> ()  [unwired: 2 in, 2 out]
        n296 = property on="Boolean 104" class="Bool (strict)"("Visible"=w15) -> ()  [unwired: 2 in, 2 out]
        n297 = property on="Boolean 105" class="Bool (strict)"("Visible"=w15) -> ()  [unwired: 2 in, 2 out]
        n298 = property on="Boolean 106" class="Bool (strict)"("Visible"=w15) -> ()  [unwired: 2 in, 2 out]
        n299 = property on="Boolean 107" class="Bool (strict)"("Visible"=w15) -> ()  [unwired: 2 in, 2 out]
        n300 = property on="Boolean 108" class="Bool (strict)"("Visible"=w15) -> ()  [unwired: 2 in, 2 out]
        n301 = property on="Boolean 109" class="Bool (strict)"("Visible"=w15) -> ()  [unwired: 2 in, 2 out]
        n302 = property on="Boolean 41" class="Bool (strict)"("Visible"=w15) -> ()  [unwired: 2 in, 2 out]
        n303 = property on="Boolean" class="Bool (strict)"("Visible"=w15) -> ()  [unwired: 2 in, 2 out]
        n304 = property on="OK Button 70" class="Bool (strict)"("Visible"=w15) -> ()  [unwired: 2 in, 2 out]
        n305 = property on="Boolean 100" class="Bool (strict)"("Value"=w14) -> ()  [unwired: 2 in, 2 out]
        n306 = property on="Boolean 101" class="Bool (strict)"("Value"=w14) -> ()  [unwired: 2 in, 2 out]
        n307 = property on="Boolean 102" class="Bool (strict)"("Value"=w14) -> ()  [unwired: 2 in, 2 out]
        n308 = property on="Boolean 103" class="Bool (strict)"("Value"=w14) -> ()  [unwired: 2 in, 2 out]
        n309 = property on="Boolean 104" class="Bool (strict)"("Value"=w14) -> ()  [unwired: 2 in, 2 out]
        n310 = property on="Boolean 105" class="Bool (strict)"("Value"=w14) -> ()  [unwired: 2 in, 2 out]
        n311 = property on="Boolean 106" class="Bool (strict)"("Value"=w14) -> ()  [unwired: 2 in, 2 out]
        n312 = property on="Boolean 107" class="Bool (strict)"("Value"=w14) -> ()  [unwired: 2 in, 2 out]
        n313 = property on="Boolean 108" class="Bool (strict)"("Value"=w14) -> ()  [unwired: 2 in, 2 out]
        n314 = property on="Boolean 109" class="Bool (strict)"("Value"=w14) -> ()  [unwired: 2 in, 2 out]
        n315 = property on="Boolean 41" class="Bool (strict)"("Value"=w14) -> ()  [unwired: 2 in, 2 out]
        n316 = property on="Boolean" class="Bool (strict)"("Value"=w14) -> ()  [unwired: 2 in, 2 out]
        n317 = property on="OK Button 70" class="Bool (strict)"("Value"=w14) -> ()  [unwired: 2 in, 2 out]
        n318 = property on="OK Button 118" class="Bool (strict)"("Visible"=w9) -> ()  [unwired: 2 in, 2 out]
        n319 = property on="OK Button 117" class="Bool (strict)"("Visible"=w9) -> ()  [unwired: 2 in, 2 out]
        n320 = property on="OK Button 108" class="Bool (strict)"("Visible"=w9) -> ()  [unwired: 2 in, 2 out]
        n321 = property on="OK Button 107" class="Bool (strict)"("Visible"=w9) -> ()  [unwired: 2 in, 2 out]
        n322 = property on="OK Button 114" class="Bool (strict)"("Visible"=w9) -> ()  [unwired: 2 in, 2 out]
        n323 = property on="OK Button 116" class="Bool (strict)"("Visible"=w9) -> ()  [unwired: 2 in, 2 out]
        n324 = property on="OK Button 115" class="Bool (strict)"("Visible"=w9) -> ()  [unwired: 2 in, 2 out]
        n325 = property on="OK Button 145" class="Bool (strict)"("Visible"=w9) -> ()  [unwired: 2 in, 2 out]
        n326 = property on="OK Button 164" class="Bool (strict)"("Visible"=w9) -> ()  [unwired: 2 in, 2 out]
        n327 = property on="OK Button 133" class="Bool (strict)"("Visible"=w9) -> ()  [unwired: 2 in, 2 out]
        n328 = property on="OK Button 156" class="Bool (strict)"("Visible"=w9) -> ()  [unwired: 2 in, 2 out]
        n329 = property on="OK Button 126" class="Bool (strict)"("Visible"=w9) -> ()  [unwired: 2 in, 2 out]
        n330 = property on="OK Button 149" class="Bool (strict)"("Visible"=w9) -> ()  [unwired: 2 in, 2 out]
        n331 = property on="OK Button 138" class="Bool (strict)"("Visible"=w9) -> ()  [unwired: 2 in, 2 out]
        n332 = property on="Boolean 114" class="Bool (strict)"("Visible"=w15) -> ()  [unwired: 2 in, 2 out]
        n333 = property on="OK Button 36" class="Bool (strict)"("Visible"=w15) -> ()  [unwired: 2 in, 2 out]
        n334 = property on="Boolean 110" class="Bool (strict)"("Visible"=w15) -> ()  [unwired: 2 in, 2 out]
        n335 = property on="Boolean 111" class="Bool (strict)"("Visible"=w15) -> ()  [unwired: 2 in, 2 out]
        n336 = property on="Boolean 112" class="Bool (strict)"("Visible"=w15) -> ()  [unwired: 2 in, 2 out]
        n337 = property on="Boolean 115" class="Bool (strict)"("Visible"=w15) -> ()  [unwired: 2 in, 2 out]
        n338 = property on="Boolean 116" class="Bool (strict)"("Visible"=w15) -> ()  [unwired: 2 in, 2 out]
        n339 = property on="Boolean 117" class="Bool (strict)"("Visible"=w15) -> ()  [unwired: 2 in, 2 out]
        n340 = property on="Boolean 118" class="Bool (strict)"("Visible"=w15) -> ()  [unwired: 2 in, 2 out]
        n341 = property on="Boolean 113" class="Bool (strict)"("Visible"=w15) -> ()  [unwired: 2 in, 2 out]
        n342 = property on="Boolean 119" class="Bool (strict)"("Visible"=w15) -> ()  [unwired: 2 in, 2 out]
        n343 = property on="OK Button 37" class="Bool (strict)"("Visible"=w15) -> ()  [unwired: 2 in, 2 out]
        n344 = property on="Boolean 114" class="Bool (strict)"("Value"=w14) -> ()  [unwired: 2 in, 2 out]
        n345 = property on="OK Button 36" class="Bool (strict)"("Value"=w14) -> ()  [unwired: 2 in, 2 out]
        n346 = property on="Boolean 110" class="Bool (strict)"("Value"=w14) -> ()  [unwired: 2 in, 2 out]
        n347 = property on="Boolean 111" class="Bool (strict)"("Value"=w14) -> ()  [unwired: 2 in, 2 out]
        n348 = property on="Boolean 112" class="Bool (strict)"("Value"=w14) -> ()  [unwired: 2 in, 2 out]
        n349 = property on="Boolean 115" class="Bool (strict)"("Value"=w14) -> ()  [unwired: 2 in, 2 out]
        n350 = property on="Boolean 116" class="Bool (strict)"("Value"=w14) -> ()  [unwired: 2 in, 2 out]
        n351 = property on="Boolean 117" class="Bool (strict)"("Value"=w14) -> ()  [unwired: 2 in, 2 out]
        n352 = property on="Boolean 118" class="Bool (strict)"("Value"=w14) -> ()  [unwired: 2 in, 2 out]
        n353 = property on="Boolean 113" class="Bool (strict)"("Value"=w14) -> ()  [unwired: 2 in, 2 out]
        n354 = property on="Boolean 119" class="Bool (strict)"("Value"=w14) -> ()  [unwired: 2 in, 2 out]
        n355 = property on="OK Button 37" class="Bool (strict)"("Value"=w14) -> ()  [unwired: 2 in, 2 out]
        n356 = property on="OK Button 122" class="Bool (strict)"("Visible"=w9) -> ()  [unwired: 2 in, 2 out]
        n357 = property on="OK Button 119" class="Bool (strict)"("Visible"=w9) -> ()  [unwired: 2 in, 2 out]
        n358 = property on="OK Button 121" class="Bool (strict)"("Visible"=w9) -> ()  [unwired: 2 in, 2 out]
        n359 = property on="OK Button 99" class="Bool (strict)"("Visible"=w9) -> ()  [unwired: 2 in, 2 out]
        n360 = property on="OK Button 120" class="Bool (strict)"("Visible"=w9) -> ()  [unwired: 2 in, 2 out]
        n361 = property on="OK Button 123" class="Bool (strict)"("Visible"=w9) -> ()  [unwired: 2 in, 2 out]
        n362 = property on="OK Button 84" class="Bool (strict)"("Visible"=w9) -> ()  [unwired: 2 in, 2 out]
        n363 = property on="Boolean 125" class="Bool (strict)"("Visible"=w15) -> ()  [unwired: 2 in, 2 out]
        n364 = property on="Boolean 120" class="Bool (strict)"("Visible"=w15) -> ()  [unwired: 2 in, 2 out]
        n365 = property on="Boolean 121" class="Bool (strict)"("Visible"=w15) -> ()  [unwired: 2 in, 2 out]
        n366 = property on="Boolean 122" class="Bool (strict)"("Visible"=w15) -> ()  [unwired: 2 in, 2 out]
        n367 = property on="Boolean 123" class="Bool (strict)"("Visible"=w15) -> ()  [unwired: 2 in, 2 out]
        n368 = property on="Boolean 126" class="Bool (strict)"("Visible"=w15) -> ()  [unwired: 2 in, 2 out]
        n369 = property on="Boolean 127" class="Bool (strict)"("Visible"=w15) -> ()  [unwired: 2 in, 2 out]
        n370 = property on="Boolean 128" class="Bool (strict)"("Visible"=w15) -> ()  [unwired: 2 in, 2 out]
        n371 = property on="Boolean 129" class="Bool (strict)"("Visible"=w15) -> ()  [unwired: 2 in, 2 out]
        n372 = property on="Boolean 124" class="Bool (strict)"("Visible"=w15) -> ()  [unwired: 2 in, 2 out]
        n373 = property on="Boolean 130" class="Bool (strict)"("Visible"=w15) -> ()  [unwired: 2 in, 2 out]
        n374 = property on="Boolean 45" class="Bool (strict)"("Visible"=w15) -> ()  [unwired: 2 in, 2 out]
        n375 = property on="OK Button 135" class="Bool (strict)"("Visible"=w9) -> ()  [unwired: 2 in, 2 out]
        n376 = property on="OK Button 147" class="Bool (strict)"("Visible"=w9) -> ()  [unwired: 2 in, 2 out]
        n377 = property on="OK Button 158" class="Bool (strict)"("Visible"=w9) -> ()  [unwired: 2 in, 2 out]
        n378 = property on="OK Button 150" class="Bool (strict)"("Visible"=w9) -> ()  [unwired: 2 in, 2 out]
        n379 = property on="OK Button 139" class="Bool (strict)"("Visible"=w9) -> ()  [unwired: 2 in, 2 out]
        n380 = property on="OK Button 160" class="Bool (strict)"("Visible"=w9) -> ()  [unwired: 2 in, 2 out]
        n381 = property on="Boolean 125" class="Bool (strict)"("Value"=w14) -> ()  [unwired: 2 in, 2 out]
        n382 = property on="Boolean 120" class="Bool (strict)"("Value"=w14) -> ()  [unwired: 2 in, 2 out]
        n383 = property on="Boolean 121" class="Bool (strict)"("Value"=w14) -> ()  [unwired: 2 in, 2 out]
        n384 = property on="Boolean 122" class="Bool (strict)"("Value"=w14) -> ()  [unwired: 2 in, 2 out]
        n385 = property on="Boolean 123" class="Bool (strict)"("Value"=w14) -> ()  [unwired: 2 in, 2 out]
        n386 = property on="OK Button 127" class="Bool (strict)"("Visible"=w9) -> ()  [unwired: 2 in, 2 out]
        n387 = property on="Boolean 126" class="Bool (strict)"("Value"=w14) -> ()  [unwired: 2 in, 2 out]
        n388 = property on="Boolean 127" class="Bool (strict)"("Value"=w14) -> ()  [unwired: 2 in, 2 out]
        n389 = property on="Boolean 128" class="Bool (strict)"("Value"=w14) -> ()  [unwired: 2 in, 2 out]
        n390 = property on="Boolean 129" class="Bool (strict)"("Value"=w14) -> ()  [unwired: 2 in, 2 out]
        n391 = property on="Boolean 124" class="Bool (strict)"("Value"=w14) -> ()  [unwired: 2 in, 2 out]
        n392 = property on="Boolean 130" class="Bool (strict)"("Value"=w14) -> ()  [unwired: 2 in, 2 out]
        n393 = property on="Boolean 45" class="Bool (strict)"("Value"=w14) -> ()  [unwired: 2 in, 2 out]
        n394 = property on="Boolean 140" class="Bool (strict)"("Visible"=w15) -> ()  [unwired: 2 in, 2 out]
        n395 = property on="Boolean 136" class="Bool (strict)"("Visible"=w15) -> ()  [unwired: 2 in, 2 out]
        n396 = property on="OK Button 109" class="Bool (strict)"("Visible"=w9) -> ()  [unwired: 2 in, 2 out]
        n397 = property on="Boolean 131" class="Bool (strict)"("Visible"=w15) -> ()  [unwired: 2 in, 2 out]
        n398 = property on="Boolean 132" class="Bool (strict)"("Visible"=w15) -> ()  [unwired: 2 in, 2 out]
        n399 = property on="Boolean 133" class="Bool (strict)"("Visible"=w15) -> ()  [unwired: 2 in, 2 out]
        n400 = property on="Boolean 134" class="Bool (strict)"("Visible"=w15) -> ()  [unwired: 2 in, 2 out]
        n401 = property on="Boolean 141" class="Bool (strict)"("Visible"=w15) -> ()  [unwired: 2 in, 2 out]
        n402 = property on="Boolean 137" class="Bool (strict)"("Visible"=w15) -> ()  [unwired: 2 in, 2 out]
        n403 = property on="Boolean 138" class="Bool (strict)"("Visible"=w15) -> ()  [unwired: 2 in, 2 out]
        n404 = property on="Boolean 139" class="Bool (strict)"("Visible"=w15) -> ()  [unwired: 2 in, 2 out]
        n405 = property on="Boolean 135" class="Bool (strict)"("Visible"=w15) -> ()  [unwired: 2 in, 2 out]
        n406 = property on="Boolean 44" class="Bool (strict)"("Visible"=w15) -> ()  [unwired: 2 in, 2 out]
        n407 = property on="Boolean 140" class="Bool (strict)"("Value"=w14) -> ()  [unwired: 2 in, 2 out]
        n408 = property on="Boolean 136" class="Bool (strict)"("Value"=w14) -> ()  [unwired: 2 in, 2 out]
        n409 = property on="Boolean 131" class="Bool (strict)"("Value"=w14) -> ()  [unwired: 2 in, 2 out]
        n410 = property on="Boolean 132" class="Bool (strict)"("Value"=w14) -> ()  [unwired: 2 in, 2 out]
        n411 = property on="Boolean 133" class="Bool (strict)"("Value"=w14) -> ()  [unwired: 2 in, 2 out]
        n412 = property on="Boolean 134" class="Bool (strict)"("Value"=w14) -> ()  [unwired: 2 in, 2 out]
        n413 = property on="Boolean 141" class="Bool (strict)"("Value"=w14) -> ()  [unwired: 2 in, 2 out]
        n414 = property on="Boolean 137" class="Bool (strict)"("Value"=w14) -> ()  [unwired: 2 in, 2 out]
        n415 = property on="Boolean 138" class="Bool (strict)"("Value"=w14) -> ()  [unwired: 2 in, 2 out]
        n416 = property on="Boolean 139" class="Bool (strict)"("Value"=w14) -> ()  [unwired: 2 in, 2 out]
        n417 = property on="Boolean 135" class="Bool (strict)"("Value"=w14) -> ()  [unwired: 2 in, 2 out]
        n418 = property on="Boolean 44" class="Bool (strict)"("Value"=w14) -> ()  [unwired: 2 in, 2 out]
        n419 = property on="OK Button 87" class="Bool (strict)"("Visible"=w9) -> ()  [unwired: 2 in, 2 out]
        n420 = property on="OK Button 86" class="Bool (strict)"("Visible"=w9) -> ()  [unwired: 2 in, 2 out]
        n421 = property on="OK Button 88" class="Bool (strict)"("Visible"=w9) -> ()  [unwired: 2 in, 2 out]
        n422 = property on="OK Button 85" class="Bool (strict)"("Visible"=w9) -> ()  [unwired: 2 in, 2 out]
        n423 = property on="OK Button 91" class="Bool (strict)"("Visible"=w9) -> ()  [unwired: 2 in, 2 out]
        n424 = property on="OK Button 89" class="Bool (strict)"("Visible"=w9) -> ()  [unwired: 2 in, 2 out]
        n425 = property on="OK Button 90" class="Bool (strict)"("Visible"=w9) -> ()  [unwired: 2 in, 2 out]
        n426 = property on="OK Button 159" class="Bool (strict)"("Visible"=w9) -> ()  [unwired: 2 in, 2 out]
        n427 = property on="OK Button 134" class="Bool (strict)"("Visible"=w9) -> ()  [unwired: 2 in, 2 out]
        n428 = property on="OK Button 151" class="Bool (strict)"("Visible"=w9) -> ()  [unwired: 2 in, 2 out]
        n429 = property on="OK Button 140" class="Bool (strict)"("Visible"=w9) -> ()  [unwired: 2 in, 2 out]
        n430 = property on="OK Button 146" class="Bool (strict)"("Visible"=w9) -> ()  [unwired: 2 in, 2 out]
        n431 = property on="OK Button 157" class="Bool (strict)"("Visible"=w9) -> ()  [unwired: 2 in, 2 out]
        n432 = property on="OK Button 128" class="Bool (strict)"("Visible"=w9) -> ()  [unwired: 2 in, 2 out]
        n433 = property on="OK Button 43" class="Bool (strict)"("Visible"=w15) -> ()  [unwired: 2 in, 2 out]
        n434 = property on="OK Button 38" class="Bool (strict)"("Visible"=w15) -> ()  [unwired: 2 in, 2 out]
        n435 = property on="OK Button 39" class="Bool (strict)"("Visible"=w15) -> ()  [unwired: 2 in, 2 out]
        n436 = property on="OK Button 40" class="Bool (strict)"("Visible"=w15) -> ()  [unwired: 2 in, 2 out]
        n437 = property on="OK Button 41" class="Bool (strict)"("Visible"=w15) -> ()  [unwired: 2 in, 2 out]
        n438 = property on="OK Button 44" class="Bool (strict)"("Visible"=w15) -> ()  [unwired: 2 in, 2 out]
        n439 = property on="OK Button 45" class="Bool (strict)"("Visible"=w15) -> ()  [unwired: 2 in, 2 out]
        n440 = property on="OK Button 46" class="Bool (strict)"("Visible"=w15) -> ()  [unwired: 2 in, 2 out]
        n441 = property on="OK Button 47" class="Bool (strict)"("Visible"=w15) -> ()  [unwired: 2 in, 2 out]
        n442 = property on="OK Button 42" class="Bool (strict)"("Visible"=w15) -> ()  [unwired: 2 in, 2 out]
        n443 = property on="OK Button 48" class="Bool (strict)"("Visible"=w15) -> ()  [unwired: 2 in, 2 out]
        n444 = property on="OK Button 49" class="Bool (strict)"("Visible"=w15) -> ()  [unwired: 2 in, 2 out]
        n445 = property on="OK Button 43" class="Bool (strict)"("Value"=w14) -> ()  [unwired: 2 in, 2 out]
        n446 = property on="OK Button 38" class="Bool (strict)"("Value"=w14) -> ()  [unwired: 2 in, 2 out]
        n447 = property on="OK Button 39" class="Bool (strict)"("Value"=w14) -> ()  [unwired: 2 in, 2 out]
        n448 = property on="OK Button 40" class="Bool (strict)"("Value"=w14) -> ()  [unwired: 2 in, 2 out]
        n449 = property on="OK Button 41" class="Bool (strict)"("Value"=w14) -> ()  [unwired: 2 in, 2 out]
        n450 = property on="OK Button 44" class="Bool (strict)"("Value"=w14) -> ()  [unwired: 2 in, 2 out]
        n451 = property on="OK Button 45" class="Bool (strict)"("Value"=w14) -> ()  [unwired: 2 in, 2 out]
        n452 = property on="OK Button 46" class="Bool (strict)"("Value"=w14) -> ()  [unwired: 2 in, 2 out]
        n453 = property on="OK Button 47" class="Bool (strict)"("Value"=w14) -> ()  [unwired: 2 in, 2 out]
        n454 = property on="OK Button 42" class="Bool (strict)"("Value"=w14) -> ()  [unwired: 2 in, 2 out]
        n455 = property on="OK Button 48" class="Bool (strict)"("Value"=w14) -> ()  [unwired: 2 in, 2 out]
        n456 = property on="OK Button 49" class="Bool (strict)"("Value"=w14) -> ()  [unwired: 2 in, 2 out]
        n457 = property on="OK Button 104" class="Bool (strict)"("Visible"=w9) -> ()  [unwired: 2 in, 2 out]
        n458 = property on="OK Button 113" class="Bool (strict)"("Visible"=w9) -> ()  [unwired: 2 in, 2 out]
        n459 = property on="OK Button 130" class="Bool (strict)"("Visible"=w9) -> ()  [unwired: 2 in, 2 out]
        n460 = property on="OK Button 142" class="Bool (strict)"("Visible"=w9) -> ()  [unwired: 2 in, 2 out]
        n461 = property on="OK Button 101" class="Bool (strict)"("Visible"=w9) -> ()  [unwired: 2 in, 2 out]
        n462 = property on="OK Button 153" class="Bool (strict)"("Visible"=w9) -> ()  [unwired: 2 in, 2 out]
        n463 = property on="OK Button 102" class="Bool (strict)"("Visible"=w9) -> ()  [unwired: 2 in, 2 out]
        n464 = property on="OK Button 161" class="Bool (strict)"("Visible"=w9) -> ()  [unwired: 2 in, 2 out]
        n465 = property on="OK Button 103" class="Bool (strict)"("Visible"=w9) -> ()  [unwired: 2 in, 2 out]
        n466 = property on="OK Button 105" class="Bool (strict)"("Visible"=w9) -> ()  [unwired: 2 in, 2 out]
        n467 = property on="OK Button 152" class="Bool (strict)"("Visible"=w9) -> ()  [unwired: 2 in, 2 out]
        n468 = property on="OK Button 141" class="Bool (strict)"("Visible"=w9) -> ()  [unwired: 2 in, 2 out]
        n469 = property on="OK Button 129" class="Bool (strict)"("Visible"=w9) -> ()  [unwired: 2 in, 2 out]
        n470 = property on="OK Button 100" class="Bool (strict)"("Visible"=w9) -> ()  [unwired: 2 in, 2 out]
        n471 = property on="OK Button 67" class="Bool (strict)"("Visible"=w15) -> ()  [unwired: 2 in, 2 out]
        n472 = property on="OK Button 62" class="Bool (strict)"("Visible"=w15) -> ()  [unwired: 2 in, 2 out]
        n473 = property on="OK Button 63" class="Bool (strict)"("Visible"=w15) -> ()  [unwired: 2 in, 2 out]
        n474 = property on="OK Button 64" class="Bool (strict)"("Visible"=w15) -> ()  [unwired: 2 in, 2 out]
        n475 = property on="OK Button 65" class="Bool (strict)"("Visible"=w15) -> ()  [unwired: 2 in, 2 out]
        n476 = property on="OK Button 68" class="Bool (strict)"("Visible"=w15) -> ()  [unwired: 2 in, 2 out]
        n477 = property on="OK Button 69" class="Bool (strict)"("Visible"=w15) -> ()  [unwired: 2 in, 2 out]
        n478 = property on="Boolean 70" class="Bool (strict)"("Visible"=w15) -> ()  [unwired: 2 in, 2 out]
        n479 = property on="OK Button 71" class="Bool (strict)"("Visible"=w15) -> ()  [unwired: 2 in, 2 out]
        n480 = property on="OK Button 66" class="Bool (strict)"("Visible"=w15) -> ()  [unwired: 2 in, 2 out]
        n481 = property on="OK Button 72" class="Bool (strict)"("Visible"=w15) -> ()  [unwired: 2 in, 2 out]
        n482 = property on="OK Button 74" class="Bool (strict)"("Visible"=w15) -> ()  [unwired: 2 in, 2 out]
        n483 = property on="OK Button 67" class="Bool (strict)"("Value"=w14) -> ()  [unwired: 2 in, 2 out]
        n484 = property on="OK Button 62" class="Bool (strict)"("Value"=w14) -> ()  [unwired: 2 in, 2 out]
        n485 = property on="OK Button 63" class="Bool (strict)"("Value"=w14) -> ()  [unwired: 2 in, 2 out]
        n486 = property on="OK Button 64" class="Bool (strict)"("Value"=w14) -> ()  [unwired: 2 in, 2 out]
        n487 = property on="OK Button 65" class="Bool (strict)"("Value"=w14) -> ()  [unwired: 2 in, 2 out]
        n488 = property on="OK Button 68" class="Bool (strict)"("Value"=w14) -> ()  [unwired: 2 in, 2 out]
        n489 = property on="OK Button 69" class="Bool (strict)"("Value"=w14) -> ()  [unwired: 2 in, 2 out]
        n490 = property on="Boolean 70" class="Bool (strict)"("Value"=w14) -> ()  [unwired: 2 in, 2 out]
        n491 = property on="OK Button 71" class="Bool (strict)"("Value"=w14) -> ()  [unwired: 2 in, 2 out]
        n492 = property on="OK Button 66" class="Bool (strict)"("Value"=w14) -> ()  [unwired: 2 in, 2 out]
        n493 = property on="OK Button 72" class="Bool (strict)"("Value"=w14) -> ()  [unwired: 2 in, 2 out]
        n494 = property on="OK Button 74" class="Bool (strict)"("Value"=w14) -> ()  [unwired: 2 in, 2 out]
        n495 = property on="OK Button 143" class="Bool (strict)"("Value"=w8) -> ()  [unwired: 2 in, 2 out]
        n496 = property on="OK Button 131" class="Bool (strict)"("Value"=w8) -> ()  [unwired: 2 in, 2 out]
        n497 = property on="OK Button 144" class="Bool (strict)"("Value"=w8) -> ()  [unwired: 2 in, 2 out]
        n498 = property on="OK Button 162" class="Bool (strict)"("Value"=w8) -> ()  [unwired: 2 in, 2 out]
        n499 = property on="OK Button 154" class="Bool (strict)"("Value"=w8) -> ()  [unwired: 2 in, 2 out]
        n500 = property on="OK Button 81" class="Bool (strict)"("Value"=w8) -> ()  [unwired: 2 in, 2 out]
        n501 = property on="OK Button 83" class="Bool (strict)"("Value"=w8) -> ()  [unwired: 2 in, 2 out]
        n502 = property on="OK Button 77" class="Bool (strict)"("Value"=w8) -> ()  [unwired: 2 in, 2 out]
        n503 = property on="OK Button 80" class="Bool (strict)"("Value"=w8) -> ()  [unwired: 2 in, 2 out]
        n504 = property on="OK Button 124" class="Bool (strict)"("Value"=w8) -> ()  [unwired: 2 in, 2 out]
        n505 = property on="OK Button 79" class="Bool (strict)"("Value"=w8) -> ()  [unwired: 2 in, 2 out]
        n506 = property on="OK Button 82" class="Bool (strict)"("Value"=w8) -> ()  [unwired: 2 in, 2 out]
        n507 = property on="OK Button 136" class="Bool (strict)"("Value"=w8) -> ()  [unwired: 2 in, 2 out]
        n508 = property on="OK Button 78" class="Bool (strict)"("Value"=w8) -> ()  [unwired: 2 in, 2 out]
        n509 = property on="Boolean 52" class="Bool (strict)"("Visible"=w15) -> ()  [unwired: 2 in, 2 out]
        n510 = property on="Boolean 48" class="Bool (strict)"("Visible"=w15) -> ()  [unwired: 2 in, 2 out]
        n511 = property on="Boolean 49" class="Bool (strict)"("Visible"=w15) -> ()  [unwired: 2 in, 2 out]
        n512 = property on="Boolean 47" class="Bool (strict)"("Visible"=w15) -> ()  [unwired: 2 in, 2 out]
        n513 = property on="Boolean 50" class="Bool (strict)"("Visible"=w15) -> ()  [unwired: 2 in, 2 out]
        n514 = property on="Boolean 58" class="Bool (strict)"("Visible"=w15) -> ()  [unwired: 2 in, 2 out]
        n515 = property on="Boolean 53" class="Bool (strict)"("Visible"=w15) -> ()  [unwired: 2 in, 2 out]
        n516 = property on="Boolean 54" class="Bool (strict)"("Visible"=w15) -> ()  [unwired: 2 in, 2 out]
        n517 = property on="Boolean 55" class="Bool (strict)"("Visible"=w15) -> ()  [unwired: 2 in, 2 out]
        n518 = property on="Boolean 56" class="Bool (strict)"("Visible"=w15) -> ()  [unwired: 2 in, 2 out]
        n519 = property on="Boolean 51" class="Bool (strict)"("Visible"=w15) -> ()  [unwired: 2 in, 2 out]
        n520 = property on="Boolean 57" class="Bool (strict)"("Visible"=w15) -> ()  [unwired: 2 in, 2 out]
        n521 = property on="Boolean 52" class="Bool (strict)"("Value"=w14) -> ()  [unwired: 2 in, 2 out]
        n522 = property on="Boolean 48" class="Bool (strict)"("Value"=w14) -> ()  [unwired: 2 in, 2 out]
        n523 = property on="Boolean 49" class="Bool (strict)"("Value"=w14) -> ()  [unwired: 2 in, 2 out]
        n524 = property on="Boolean 47" class="Bool (strict)"("Value"=w14) -> ()  [unwired: 2 in, 2 out]
        n525 = property on="Boolean 50" class="Bool (strict)"("Value"=w14) -> ()  [unwired: 2 in, 2 out]
        n526 = property on="Boolean 58" class="Bool (strict)"("Value"=w14) -> ()  [unwired: 2 in, 2 out]
        n527 = property on="Boolean 53" class="Bool (strict)"("Value"=w14) -> ()  [unwired: 2 in, 2 out]
        n528 = property on="Boolean 54" class="Bool (strict)"("Value"=w14) -> ()  [unwired: 2 in, 2 out]
        n529 = property on="Boolean 55" class="Bool (strict)"("Value"=w14) -> ()  [unwired: 2 in, 2 out]
        n530 = property on="Boolean 56" class="Bool (strict)"("Value"=w14) -> ()  [unwired: 2 in, 2 out]
        n531 = property on="Boolean 51" class="Bool (strict)"("Value"=w14) -> ()  [unwired: 2 in, 2 out]
        n532 = property on="Boolean 57" class="Bool (strict)"("Value"=w14) -> ()  [unwired: 2 in, 2 out]
        n533 = property on="OK Button 132" class="Bool (strict)"("Value"=w8) -> ()  [unwired: 2 in, 2 out]
        n534 = property on="OK Button 112" class="Bool (strict)"("Value"=w8) -> ()  [unwired: 2 in, 2 out]
        n535 = property on="OK Button 92" class="Bool (strict)"("Value"=w8) -> ()  [unwired: 2 in, 2 out]
        n536 = property on="OK Button 96" class="Bool (strict)"("Value"=w8) -> ()  [unwired: 2 in, 2 out]
        n537 = property on="OK Button 110" class="Bool (strict)"("Value"=w8) -> ()  [unwired: 2 in, 2 out]
        n538 = property on="OK Button 148" class="Bool (strict)"("Value"=w8) -> ()  [unwired: 2 in, 2 out]
        n539 = property on="OK Button 163" class="Bool (strict)"("Value"=w8) -> ()  [unwired: 2 in, 2 out]
        n540 = property on="OK Button 155" class="Bool (strict)"("Value"=w8) -> ()  [unwired: 2 in, 2 out]
        n541 = property on="OK Button 137" class="Bool (strict)"("Value"=w8) -> ()  [unwired: 2 in, 2 out]
        n542 = property on="OK Button 95" class="Bool (strict)"("Value"=w8) -> ()  [unwired: 2 in, 2 out]
        n543 = property on="OK Button 165" class="Bool (strict)"("Value"=w8) -> ()  [unwired: 2 in, 2 out]
        n544 = property on="OK Button 93" class="Bool (strict)"("Value"=w8) -> ()  [unwired: 2 in, 2 out]
        n545 = property on="OK Button 97" class="Bool (strict)"("Value"=w8) -> ()  [unwired: 2 in, 2 out]
        n546 = property on="OK Button 125" class="Bool (strict)"("Value"=w8) -> ()  [unwired: 2 in, 2 out]
        n547 = property on="Array 2" class="Arr (strict)"("Visible"=w7) -> ()  [unwired: 2 in, 2 out]
        n548 = property on="Boolean 143" class="Bool (strict)"("Visible"=w7) -> ()  [unwired: 2 in, 2 out]
        n549 = property on="Boolean 143" class="Bool (strict)"("Value"=w7) -> ()  [unwired: 2 in, 2 out]
        n550 = property on="Array 2" class="Arr (strict)"("Value"=bool[][] [[FALSE, FALSE, FALSE, FALSE, FALSE, FALSE, FALSE, FALSE, FALSE, FALSE, FALSE, FALSE, FALSE], [FALSE, FALSE, FALSE, FALSE, FALSE, FALSE, FALSE, FALSE, FALSE, FALSE, FALSE, FALSE, FALSE], [FALSE, FALSE, FALSE, FALSE, FALSE, FALSE, FALSE, FALSE, FALSE, FALSE, FALSE, FALSE, FALSE], [FALSE, FALSE, FALSE, FALSE, FALSE, FALSE, FALSE, FALSE, FALSE, FALSE, FALSE, FALSE, FALSE], [FALSE, FALSE, FALSE, FALSE, FALSE, FALSE, FALSE, FALSE, FALSE, FALSE, FALSE, FALSE, FALSE], [FALSE, FALSE, FALSE, FALSE, FALSE, FALSE, FALSE, FALSE, FALSE, FALSE, FALSE, FALSE, FALSE], [FALSE, FALSE, FALSE, FALSE, FALSE, FALSE, FALSE, FALSE, FALSE, FALSE, FALSE, FALSE, FALSE], [FALSE, FALSE, FALSE, FALSE, FALSE, FALSE, FALSE, FALSE, FALSE, FALSE, FALSE, FALSE, FALSE], [FALSE, FALSE, FALSE, FALSE, FALSE, FALSE, FALSE, FALSE, FALSE, FALSE, FALSE, FALSE, FALSE], [FALSE, FALSE, FALSE, FALSE, FALSE, FALSE, FALSE, FALSE, FALSE, FALSE, FALSE, FALSE, FALSE], [FALSE, FALSE, FALSE, FALSE, FALSE, FALSE, FALSE, FALSE, FALSE, FALSE, FALSE, FALSE, FALSE], [FALSE, FALSE, FALSE, FALSE, FALSE, FALSE, FALSE, FALSE, FALSE, FALSE, FALSE, FALSE, FALSE], [FALSE, FALSE, FALSE, FALSE, FALSE, FALSE, FALSE, FALSE, FALSE, FALSE, FALSE, FALSE, FALSE], [FALSE, FALSE, FALSE, FALSE, FALSE, FALSE, FALSE, FALSE, FALSE, FALSE, FALSE, FALSE, FALSE], [FALSE, FALSE, FALSE, FALSE, FALSE, FALSE, FALSE, FALSE, FALSE, FALSE, FALSE, FALSE, FALSE]] ("Array 3")) -> ()  [unwired: 2 in, 2 out]
        n551 = property on="Boolean 63" class="Bool (strict)"("Visible"=w15) -> ()  [unwired: 2 in, 2 out]
        n552 = property on="Boolean 59" class="Bool (strict)"("Visible"=w15) -> ()  [unwired: 2 in, 2 out]
        n553 = property on="Boolean 60" class="Bool (strict)"("Visible"=w15) -> ()  [unwired: 2 in, 2 out]
        n554 = property on="Boolean 61" class="Bool (strict)"("Visible"=w15) -> ()  [unwired: 2 in, 2 out]
        n555 = property on="Boolean 69" class="Bool (strict)"("Visible"=w15) -> ()  [unwired: 2 in, 2 out]
        n556 = property on="Boolean 64" class="Bool (strict)"("Visible"=w15) -> ()  [unwired: 2 in, 2 out]
        n557 = property on="Boolean 65" class="Bool (strict)"("Visible"=w15) -> ()  [unwired: 2 in, 2 out]
        n558 = property on="Boolean 66" class="Bool (strict)"("Visible"=w15) -> ()  [unwired: 2 in, 2 out]
        n559 = property on="Boolean 67" class="Bool (strict)"("Visible"=w15) -> ()  [unwired: 2 in, 2 out]
        n560 = property on="OK Button 73" class="Bool (strict)"("Visible"=w15) -> ()  [unwired: 2 in, 2 out]
        n561 = property on="Boolean 62" class="Bool (strict)"("Visible"=w15) -> ()  [unwired: 2 in, 2 out]
        n562 = property on="Boolean 68" class="Bool (strict)"("Visible"=w15) -> ()  [unwired: 2 in, 2 out]
        n563 = property on="Boolean 63" class="Bool (strict)"("Value"=w14) -> ()  [unwired: 2 in, 2 out]
        n564 = property on="Boolean 59" class="Bool (strict)"("Value"=w14) -> ()  [unwired: 2 in, 2 out]
        n565 = property on="Boolean 60" class="Bool (strict)"("Value"=w14) -> ()  [unwired: 2 in, 2 out]
        n566 = property on="Boolean 61" class="Bool (strict)"("Value"=w14) -> ()  [unwired: 2 in, 2 out]
        n567 = property on="Boolean 69" class="Bool (strict)"("Value"=w14) -> ()  [unwired: 2 in, 2 out]
        n568 = property on="Boolean 64" class="Bool (strict)"("Value"=w14) -> ()  [unwired: 2 in, 2 out]
        n569 = property on="Boolean 65" class="Bool (strict)"("Value"=w14) -> ()  [unwired: 2 in, 2 out]
        n570 = property on="Boolean 66" class="Bool (strict)"("Value"=w14) -> ()  [unwired: 2 in, 2 out]
        n571 = property on="Boolean 67" class="Bool (strict)"("Value"=w14) -> ()  [unwired: 2 in, 2 out]
        n572 = property on="OK Button 73" class="Bool (strict)"("Value"=w14) -> ()  [unwired: 2 in, 2 out]
        n573 = property on="Boolean 62" class="Bool (strict)"("Value"=w14) -> ()  [unwired: 2 in, 2 out]
        n574 = property on="Boolean 68" class="Bool (strict)"("Value"=w14) -> ()  [unwired: 2 in, 2 out]
        n575 = property on="Boolean 74" class="Bool (strict)"("Visible"=w15) -> ()  [unwired: 2 in, 2 out]
        n576 = property on="Boolean 70" class="Bool (strict)"("Visible"=w15) -> ()  [unwired: 2 in, 2 out]
        n577 = property on="Boolean 71" class="Bool (strict)"("Visible"=w15) -> ()  [unwired: 2 in, 2 out]
        n578 = property on="Boolean 72" class="Bool (strict)"("Visible"=w15) -> ()  [unwired: 2 in, 2 out]
        n579 = property on="Boolean 75" class="Bool (strict)"("Visible"=w15) -> ()  [unwired: 2 in, 2 out]
        n580 = property on="Boolean 76" class="Bool (strict)"("Visible"=w15) -> ()  [unwired: 2 in, 2 out]
        n581 = property on="Boolean 77" class="Bool (strict)"("Visible"=w15) -> ()  [unwired: 2 in, 2 out]
        n582 = property on="Boolean 78" class="Bool (strict)"("Visible"=w15) -> ()  [unwired: 2 in, 2 out]
        n583 = property on="Boolean 73" class="Bool (strict)"("Visible"=w15) -> ()  [unwired: 2 in, 2 out]
        n584 = property on="Boolean 79" class="Bool (strict)"("Visible"=w15) -> ()  [unwired: 2 in, 2 out]
        n585 = property on="OK Button 118" class="Bool (strict)"("Value"=w8) -> ()  [unwired: 2 in, 2 out]
        n586 = property on="OK Button 76" class="Bool (strict)"("Visible"=w15) -> ()  [unwired: 2 in, 2 out]
        n587 = property on="OK Button 117" class="Bool (strict)"("Value"=w8) -> ()  [unwired: 2 in, 2 out]
        n588 = property on="OK Button 75" class="Bool (strict)"("Visible"=w15) -> ()  [unwired: 2 in, 2 out]
        n589 = property on="OK Button 108" class="Bool (strict)"("Value"=w8) -> ()  [unwired: 2 in, 2 out]
        n590 = property on="OK Button 145" class="Bool (strict)"("Value"=w8) -> ()  [unwired: 2 in, 2 out]
        n591 = property on="OK Button 107" class="Bool (strict)"("Value"=w8) -> ()  [unwired: 2 in, 2 out]
        n592 = property on="OK Button 114" class="Bool (strict)"("Value"=w8) -> ()  [unwired: 2 in, 2 out]
        n593 = property on="OK Button 116" class="Bool (strict)"("Value"=w8) -> ()  [unwired: 2 in, 2 out]
        n594 = property on="OK Button 164" class="Bool (strict)"("Value"=w8) -> ()  [unwired: 2 in, 2 out]
        n595 = property on="OK Button 115" class="Bool (strict)"("Value"=w8) -> ()  [unwired: 2 in, 2 out]
        n596 = property on="OK Button 133" class="Bool (strict)"("Value"=w8) -> ()  [unwired: 2 in, 2 out]
        n597 = property on="OK Button 156" class="Bool (strict)"("Value"=w8) -> ()  [unwired: 2 in, 2 out]
        n598 = property on="Boolean 74" class="Bool (strict)"("Value"=w14) -> ()  [unwired: 2 in, 2 out]
        n599 = property on="Boolean 70" class="Bool (strict)"("Value"=w14) -> ()  [unwired: 2 in, 2 out]
        n600 = property on="Boolean 71" class="Bool (strict)"("Value"=w14) -> ()  [unwired: 2 in, 2 out]
        n601 = property on="Boolean 72" class="Bool (strict)"("Value"=w14) -> ()  [unwired: 2 in, 2 out]
        n602 = property on="Boolean 75" class="Bool (strict)"("Value"=w14) -> ()  [unwired: 2 in, 2 out]
        n603 = property on="Boolean 76" class="Bool (strict)"("Value"=w14) -> ()  [unwired: 2 in, 2 out]
        n604 = property on="Boolean 77" class="Bool (strict)"("Value"=w14) -> ()  [unwired: 2 in, 2 out]
        n605 = property on="Boolean 78" class="Bool (strict)"("Value"=w14) -> ()  [unwired: 2 in, 2 out]
        n606 = property on="Boolean 73" class="Bool (strict)"("Value"=w14) -> ()  [unwired: 2 in, 2 out]
        n607 = property on="Boolean 79" class="Bool (strict)"("Value"=w14) -> ()  [unwired: 2 in, 2 out]
        n608 = property on="OK Button 126" class="Bool (strict)"("Value"=w8) -> ()  [unwired: 2 in, 2 out]
        n609 = property on="OK Button 149" class="Bool (strict)"("Value"=w8) -> ()  [unwired: 2 in, 2 out]
        n610 = property on="OK Button 138" class="Bool (strict)"("Value"=w8) -> ()  [unwired: 2 in, 2 out]
        n611 = property on="OK Button 76" class="Bool (strict)"("Value"=w14) -> ()  [unwired: 2 in, 2 out]
        n612 = property on="OK Button 75" class="Bool (strict)"("Value"=w14) -> ()  [unwired: 2 in, 2 out]
        n613 = property on="OK Button 111" class="Bool (strict)"("Value"=w8) -> ()  [unwired: 2 in, 2 out]
        n614 = property on="Boolean 85" class="Bool (strict)"("Visible"=w15) -> ()  [unwired: 2 in, 2 out]
        n615 = property on="Boolean 80" class="Bool (strict)"("Visible"=w15) -> ()  [unwired: 2 in, 2 out]
        n616 = property on="Boolean 81" class="Bool (strict)"("Visible"=w15) -> ()  [unwired: 2 in, 2 out]
        n617 = property on="Boolean 82" class="Bool (strict)"("Visible"=w15) -> ()  [unwired: 2 in, 2 out]
        n618 = property on="Boolean 83" class="Bool (strict)"("Visible"=w15) -> ()  [unwired: 2 in, 2 out]
        n619 = property on="Boolean 90" class="Bool (strict)"("Visible"=w15) -> ()  [unwired: 2 in, 2 out]
        n620 = property on="Boolean 86" class="Bool (strict)"("Visible"=w15) -> ()  [unwired: 2 in, 2 out]
        n621 = property on="Boolean 87" class="Bool (strict)"("Visible"=w15) -> ()  [unwired: 2 in, 2 out]
        n622 = property on="Boolean 88" class="Bool (strict)"("Visible"=w15) -> ()  [unwired: 2 in, 2 out]
        n623 = property on="Boolean 89" class="Bool (strict)"("Visible"=w15) -> ()  [unwired: 2 in, 2 out]
        n624 = property on="Boolean 84" class="Bool (strict)"("Visible"=w15) -> ()  [unwired: 2 in, 2 out]
        n625 = property on="Boolean 46" class="Bool (strict)"("Visible"=w15) -> ()  [unwired: 2 in, 2 out]
        n626 = property on="Boolean 85" class="Bool (strict)"("Value"=w14) -> ()  [unwired: 2 in, 2 out]
        n627 = property on="Boolean 80" class="Bool (strict)"("Value"=w14) -> ()  [unwired: 2 in, 2 out]
        n628 = property on="Boolean 81" class="Bool (strict)"("Value"=w14) -> ()  [unwired: 2 in, 2 out]
        n629 = property on="Boolean 82" class="Bool (strict)"("Value"=w14) -> ()  [unwired: 2 in, 2 out]
        n630 = property on="Boolean 83" class="Bool (strict)"("Value"=w14) -> ()  [unwired: 2 in, 2 out]
        n631 = property on="Boolean 90" class="Bool (strict)"("Value"=w14) -> ()  [unwired: 2 in, 2 out]
        n632 = property on="Boolean 86" class="Bool (strict)"("Value"=w14) -> ()  [unwired: 2 in, 2 out]
        n633 = property on="Boolean 87" class="Bool (strict)"("Value"=w14) -> ()  [unwired: 2 in, 2 out]
        n634 = property on="Boolean 88" class="Bool (strict)"("Value"=w14) -> ()  [unwired: 2 in, 2 out]
        n635 = property on="Boolean 89" class="Bool (strict)"("Value"=w14) -> ()  [unwired: 2 in, 2 out]
        n636 = property on="Boolean 84" class="Bool (strict)"("Value"=w14) -> ()  [unwired: 2 in, 2 out]
        n637 = property on="Boolean 46" class="Bool (strict)"("Value"=w14) -> ()  [unwired: 2 in, 2 out]
        n638 = property on="OK Button 122" class="Bool (strict)"("Value"=w8) -> ()  [unwired: 2 in, 2 out]
        n639 = property on="OK Button 119" class="Bool (strict)"("Value"=w8) -> ()  [unwired: 2 in, 2 out]
        n640 = property on="OK Button 121" class="Bool (strict)"("Value"=w8) -> ()  [unwired: 2 in, 2 out]
        n641 = property on="OK Button 99" class="Bool (strict)"("Value"=w8) -> ()  [unwired: 2 in, 2 out]
        n642 = property on="OK Button 120" class="Bool (strict)"("Value"=w8) -> ()  [unwired: 2 in, 2 out]
        n643 = property on="OK Button 123" class="Bool (strict)"("Value"=w8) -> ()  [unwired: 2 in, 2 out]
        n644 = property on="OK Button 135" class="Bool (strict)"("Value"=w8) -> ()  [unwired: 2 in, 2 out]
        n645 = property on="OK Button 147" class="Bool (strict)"("Value"=w8) -> ()  [unwired: 2 in, 2 out]
        n646 = property on="OK Button 84" class="Bool (strict)"("Value"=w8) -> ()  [unwired: 2 in, 2 out]
        n647 = property on="OK Button 158" class="Bool (strict)"("Value"=w8) -> ()  [unwired: 2 in, 2 out]
        n648 = property on="OK Button 150" class="Bool (strict)"("Value"=w8) -> ()  [unwired: 2 in, 2 out]
        n649 = property on="OK Button 139" class="Bool (strict)"("Value"=w8) -> ()  [unwired: 2 in, 2 out]
        n650 = property on="OK Button 160" class="Bool (strict)"("Value"=w8) -> ()  [unwired: 2 in, 2 out]
        n651 = property on="OK Button 127" class="Bool (strict)"("Value"=w8) -> ()  [unwired: 2 in, 2 out]
        n652 = property on="Boolean 96" class="Bool (strict)"("Visible"=w15) -> ()  [unwired: 2 in, 2 out]
        n653 = property on="Boolean 91" class="Bool (strict)"("Visible"=w15) -> ()  [unwired: 2 in, 2 out]
        n654 = property on="Boolean 92" class="Bool (strict)"("Visible"=w15) -> ()  [unwired: 2 in, 2 out]
        n655 = property on="Boolean 93" class="Bool (strict)"("Visible"=w15) -> ()  [unwired: 2 in, 2 out]
        n656 = property on="Boolean 94" class="Bool (strict)"("Visible"=w15) -> ()  [unwired: 2 in, 2 out]
        n657 = property on="OK Button 21" class="Bool (strict)"("Visible"=w15) -> ()  [unwired: 2 in, 2 out]
        n658 = property on="Boolean 97" class="Bool (strict)"("Visible"=w15) -> ()  [unwired: 2 in, 2 out]
        n659 = property on="Boolean 98" class="Bool (strict)"("Visible"=w15) -> ()  [unwired: 2 in, 2 out]
        n660 = property on="Boolean 99" class="Bool (strict)"("Visible"=w15) -> ()  [unwired: 2 in, 2 out]
        n661 = property on="OK Butto" class="Bool (strict)"("Visible"=w15) -> ()  [unwired: 2 in, 2 out]
        n662 = property on="Boolean 95" class="Bool (strict)"("Visible"=w15) -> ()  [unwired: 2 in, 2 out]
        n663 = property on="OK Button 17" class="Bool (strict)"("Visible"=w15) -> ()  [unwired: 2 in, 2 out]
        n664 = property on="Boolean 96" class="Bool (strict)"("Value"=w14) -> ()  [unwired: 2 in, 2 out]
        n665 = property on="Boolean 91" class="Bool (strict)"("Value"=w14) -> ()  [unwired: 2 in, 2 out]
        n666 = property on="Boolean 92" class="Bool (strict)"("Value"=w14) -> ()  [unwired: 2 in, 2 out]
        n667 = property on="Boolean 93" class="Bool (strict)"("Value"=w14) -> ()  [unwired: 2 in, 2 out]
        n668 = property on="Boolean 94" class="Bool (strict)"("Value"=w14) -> ()  [unwired: 2 in, 2 out]
        n669 = property on="OK Button 21" class="Bool (strict)"("Value"=w14) -> ()  [unwired: 2 in, 2 out]
        n670 = property on="Boolean 97" class="Bool (strict)"("Value"=w14) -> ()  [unwired: 2 in, 2 out]
        n671 = property on="Boolean 98" class="Bool (strict)"("Value"=w14) -> ()  [unwired: 2 in, 2 out]
        n672 = property on="Boolean 99" class="Bool (strict)"("Value"=w14) -> ()  [unwired: 2 in, 2 out]
        n673 = property on="OK Butto" class="Bool (strict)"("Value"=w14) -> ()  [unwired: 2 in, 2 out]
        n674 = property on="Boolean 95" class="Bool (strict)"("Value"=w14) -> ()  [unwired: 2 in, 2 out]
        n675 = property on="OK Button 17" class="Bool (strict)"("Value"=w14) -> ()  [unwired: 2 in, 2 out]
        n676 = property on="OK Button 109" class="Bool (strict)"("Value"=w8) -> ()  [unwired: 2 in, 2 out]
        n677 = property on="OK Button 27" class="Bool (strict)"("Visible"=w15) -> ()  [unwired: 2 in, 2 out]
        n678 = property on="OK Button 22" class="Bool (strict)"("Visible"=w15) -> ()  [unwired: 2 in, 2 out]
        n679 = property on="OK Button 23" class="Bool (strict)"("Visible"=w15) -> ()  [unwired: 2 in, 2 out]
        n680 = property on="OK Button 25" class="Bool (strict)"("Visible"=w15) -> ()  [unwired: 2 in, 2 out]
        n681 = property on="OK Button 24" class="Bool (strict)"("Visible"=w15) -> ()  [unwired: 2 in, 2 out]
        n682 = property on="OK Button 35" class="Bool (strict)"("Visible"=w15) -> ()  [unwired: 2 in, 2 out]
        n683 = property on="OK Button 28" class="Bool (strict)"("Visible"=w15) -> ()  [unwired: 2 in, 2 out]
        n684 = property on="OK Button 31" class="Bool (strict)"("Visible"=w15) -> ()  [unwired: 2 in, 2 out]
        n685 = property on="OK Button 32" class="Bool (strict)"("Visible"=w15) -> ()  [unwired: 2 in, 2 out]
        n686 = property on="OK Button 33" class="Bool (strict)"("Visible"=w15) -> ()  [unwired: 2 in, 2 out]
        n687 = property on="OK Button 26" class="Bool (strict)"("Visible"=w15) -> ()  [unwired: 2 in, 2 out]
        n688 = property on="OK Button 34" class="Bool (strict)"("Visible"=w15) -> ()  [unwired: 2 in, 2 out]
        n689 = property on="OK Button 87" class="Bool (strict)"("Value"=w8) -> ()  [unwired: 2 in, 2 out]
        n690 = property on="OK Button 27" class="Bool (strict)"("Value"=w14) -> ()  [unwired: 2 in, 2 out]
        n691 = property on="OK Button 86" class="Bool (strict)"("Value"=w8) -> ()  [unwired: 2 in, 2 out]
        n692 = property on="OK Button 22" class="Bool (strict)"("Value"=w14) -> ()  [unwired: 2 in, 2 out]
        n693 = property on="OK Button 23" class="Bool (strict)"("Value"=w14) -> ()  [unwired: 2 in, 2 out]
        n694 = property on="OK Button 25" class="Bool (strict)"("Value"=w14) -> ()  [unwired: 2 in, 2 out]
        n695 = property on="OK Button 24" class="Bool (strict)"("Value"=w14) -> ()  [unwired: 2 in, 2 out]
        n696 = property on="OK Button 35" class="Bool (strict)"("Value"=w14) -> ()  [unwired: 2 in, 2 out]
        n697 = property on="OK Button 88" class="Bool (strict)"("Value"=w8) -> ()  [unwired: 2 in, 2 out]
        n698 = property on="OK Button 28" class="Bool (strict)"("Value"=w14) -> ()  [unwired: 2 in, 2 out]
        n699 = property on="OK Button 31" class="Bool (strict)"("Value"=w14) -> ()  [unwired: 2 in, 2 out]
        n700 = property on="OK Button 32" class="Bool (strict)"("Value"=w14) -> ()  [unwired: 2 in, 2 out]
        n701 = property on="OK Button 33" class="Bool (strict)"("Value"=w14) -> ()  [unwired: 2 in, 2 out]
        n702 = property on="OK Button 26" class="Bool (strict)"("Value"=w14) -> ()  [unwired: 2 in, 2 out]
        n703 = property on="OK Button 34" class="Bool (strict)"("Value"=w14) -> ()  [unwired: 2 in, 2 out]
        n704 = property on="OK Button 85" class="Bool (strict)"("Value"=w8) -> ()  [unwired: 2 in, 2 out]
        n705 = property on="OK Button 91" class="Bool (strict)"("Value"=w8) -> ()  [unwired: 2 in, 2 out]
        n706 = property on="OK Button 89" class="Bool (strict)"("Value"=w8) -> ()  [unwired: 2 in, 2 out]
        n707 = property on="OK Button 90" class="Bool (strict)"("Value"=w8) -> ()  [unwired: 2 in, 2 out]
        n708 = property on="OK Button 159" class="Bool (strict)"("Value"=w8) -> ()  [unwired: 2 in, 2 out]
        n709 = property on="OK Button 134" class="Bool (strict)"("Value"=w8) -> ()  [unwired: 2 in, 2 out]
        n710 = property on="OK Button 151" class="Bool (strict)"("Value"=w8) -> ()  [unwired: 2 in, 2 out]
        n711 = property on="OK Button 140" class="Bool (strict)"("Value"=w8) -> ()  [unwired: 2 in, 2 out]
        n712 = property on="OK Button 146" class="Bool (strict)"("Value"=w8) -> ()  [unwired: 2 in, 2 out]
        n713 = property on="OK Button 157" class="Bool (strict)"("Value"=w8) -> ()  [unwired: 2 in, 2 out]
        n714 = property on="OK Button 128" class="Bool (strict)"("Value"=w8) -> ()  [unwired: 2 in, 2 out]
        n715 = property on="OK Button 55" class="Bool (strict)"("Visible"=w15) -> ()  [unwired: 2 in, 2 out]
        n716 = property on="OK Button 50" class="Bool (strict)"("Visible"=w15) -> ()  [unwired: 2 in, 2 out]
        n717 = property on="OK Button 51" class="Bool (strict)"("Visible"=w15) -> ()  [unwired: 2 in, 2 out]
        n718 = property on="OK Button 52" class="Bool (strict)"("Visible"=w15) -> ()  [unwired: 2 in, 2 out]
        n719 = property on="OK Button 53" class="Bool (strict)"("Visible"=w15) -> ()  [unwired: 2 in, 2 out]
        n720 = property on="OK Button 56" class="Bool (strict)"("Visible"=w15) -> ()  [unwired: 2 in, 2 out]
        n721 = property on="OK Button 57" class="Bool (strict)"("Visible"=w15) -> ()  [unwired: 2 in, 2 out]
        n722 = property on="OK Button 58" class="Bool (strict)"("Visible"=w15) -> ()  [unwired: 2 in, 2 out]
        n723 = property on="OK Button 59" class="Bool (strict)"("Visible"=w15) -> ()  [unwired: 2 in, 2 out]
        n724 = property on="OK Button 54" class="Bool (strict)"("Visible"=w15) -> ()  [unwired: 2 in, 2 out]
        n725 = property on="OK Button 60" class="Bool (strict)"("Visible"=w15) -> ()  [unwired: 2 in, 2 out]
        n726 = property on="OK Button 61" class="Bool (strict)"("Visible"=w15) -> ()  [unwired: 2 in, 2 out]
        n727 = property on="OK Button 104" class="Bool (strict)"("Value"=w8) -> ()  [unwired: 2 in, 2 out]
        n728 = property on="OK Button 55" class="Bool (strict)"("Value"=w14) -> ()  [unwired: 2 in, 2 out]
        n729 = property on="OK Button 130" class="Bool (strict)"("Value"=w8) -> ()  [unwired: 2 in, 2 out]
        n730 = property on="OK Button 50" class="Bool (strict)"("Value"=w14) -> ()  [unwired: 2 in, 2 out]
        n731 = property on="OK Button 51" class="Bool (strict)"("Value"=w14) -> ()  [unwired: 2 in, 2 out]
        n732 = property on="OK Button 52" class="Bool (strict)"("Value"=w14) -> ()  [unwired: 2 in, 2 out]
        n733 = property on="OK Button 53" class="Bool (strict)"("Value"=w14) -> ()  [unwired: 2 in, 2 out]
        n734 = property on="OK Button 142" class="Bool (strict)"("Value"=w8) -> ()  [unwired: 2 in, 2 out]
        n735 = property on="OK Button 56" class="Bool (strict)"("Value"=w14) -> ()  [unwired: 2 in, 2 out]
        n736 = property on="OK Button 57" class="Bool (strict)"("Value"=w14) -> ()  [unwired: 2 in, 2 out]
        n737 = property on="OK Button 58" class="Bool (strict)"("Value"=w14) -> ()  [unwired: 2 in, 2 out]
        n738 = property on="OK Button 59" class="Bool (strict)"("Value"=w14) -> ()  [unwired: 2 in, 2 out]
        n739 = property on="OK Button 101" class="Bool (strict)"("Value"=w8) -> ()  [unwired: 2 in, 2 out]
        n740 = property on="OK Button 113" class="Bool (strict)"("Value"=w8) -> ()  [unwired: 2 in, 2 out]
        n741 = property on="OK Button 54" class="Bool (strict)"("Value"=w14) -> ()  [unwired: 2 in, 2 out]
        n742 = property on="OK Button 153" class="Bool (strict)"("Value"=w8) -> ()  [unwired: 2 in, 2 out]
        n743 = property on="OK Button 102" class="Bool (strict)"("Value"=w8) -> ()  [unwired: 2 in, 2 out]
        n744 = property on="OK Button 60" class="Bool (strict)"("Value"=w14) -> ()  [unwired: 2 in, 2 out]
        n745 = property on="OK Button 161" class="Bool (strict)"("Value"=w8) -> ()  [unwired: 2 in, 2 out]
        n746 = property on="OK Button 103" class="Bool (strict)"("Value"=w8) -> ()  [unwired: 2 in, 2 out]
        n747 = property on="OK Button 105" class="Bool (strict)"("Value"=w8) -> ()  [unwired: 2 in, 2 out]
        n748 = property on="OK Button 152" class="Bool (strict)"("Value"=w8) -> ()  [unwired: 2 in, 2 out]
        n749 = property on="OK Button 61" class="Bool (strict)"("Value"=w14) -> ()  [unwired: 2 in, 2 out]
        n750 = property on="OK Button 141" class="Bool (strict)"("Value"=w8) -> ()  [unwired: 2 in, 2 out]
        n751 = property on="OK Button 129" class="Bool (strict)"("Value"=w8) -> ()  [unwired: 2 in, 2 out]
        n752 = property on="OK Button 100" class="Bool (strict)"("Value"=w8) -> ()  [unwired: 2 in, 2 out]
        n753 = property on="Boolean 142" class="Bool (strict)"("Visible"=w10) -> ()  [unwired: 2 in, 2 out]
        n754 = property on="Boolean 142" class="Bool (strict)"("Value"=w10) -> ()  [unwired: 2 in, 2 out]
        n755 = property on="Array" class="Arr (strict)"("Visible"=w10) -> ()  [unwired: 2 in, 2 out]
        n756 = property on="Array" class="Arr (strict)"("Value"=bool[][] [[FALSE, FALSE, FALSE, FALSE, FALSE, FALSE, FALSE, FALSE, FALSE, FALSE, FALSE, FALSE], [FALSE, FALSE, FALSE, FALSE, FALSE, FALSE, FALSE, FALSE, FALSE, FALSE, FALSE, FALSE], [FALSE, FALSE, FALSE, FALSE, FALSE, FALSE, FALSE, FALSE, FALSE, FALSE, FALSE, FALSE], [FALSE, FALSE, FALSE, FALSE, FALSE, FALSE, FALSE, FALSE, FALSE, FALSE, FALSE, FALSE], [FALSE, FALSE, FALSE, FALSE, FALSE, FALSE, FALSE, FALSE, FALSE, FALSE, FALSE, FALSE], [FALSE, FALSE, FALSE, FALSE, FALSE, FALSE, FALSE, FALSE, FALSE, FALSE, FALSE, FALSE], [FALSE, FALSE, FALSE, FALSE, FALSE, FALSE, FALSE, FALSE, FALSE, FALSE, FALSE, FALSE], [FALSE, FALSE, FALSE, FALSE, FALSE, FALSE, FALSE, FALSE, FALSE, FALSE, FALSE, FALSE], [FALSE, FALSE, FALSE, FALSE, FALSE, FALSE, FALSE, FALSE, FALSE, FALSE, FALSE, FALSE], [FALSE, FALSE, FALSE, FALSE, FALSE, FALSE, FALSE, FALSE, FALSE, FALSE, FALSE, FALSE], [FALSE, FALSE, FALSE, FALSE, FALSE, FALSE, FALSE, FALSE, FALSE, FALSE, FALSE, FALSE], [FALSE, FALSE, FALSE, FALSE, FALSE, FALSE, FALSE, FALSE, FALSE, FALSE, FALSE, FALSE], [FALSE, FALSE, FALSE, FALSE, FALSE, FALSE, FALSE, FALSE, FALSE, FALSE, FALSE, FALSE], [FALSE, FALSE, FALSE, FALSE, FALSE, FALSE, FALSE, FALSE, FALSE, FALSE, FALSE, FALSE], [FALSE, FALSE, FALSE, FALSE, FALSE, FALSE, FALSE, FALSE, FALSE, FALSE, FALSE, FALSE]] ("Array 3")) -> ()  [unwired: 2 in, 2 out]
      }
      frame "latwy" {
        n757 = Two Button Dialog(message="wybierz rozmiar planszy", 1:"11x9" ("message"), 2:"8x5" ("message")) -> (T button?=w31:bool)
        n758 = Select(t=T2."8x5", s=w31, f=T2."11x9") -> (s? t:f=w25:T2)
      }
      frame "trudny" {
        n759 = Two Button Dialog(message="wybierz rozmiar planszy", 1:"12x15" ("message"), 2:"13x14" ("message")) -> (T button?=w34:bool)
        n760 = Select(t=T2."13x14", s=w34, f=T2."12x15") -> (s? t:f=w33:T2)
      }
      frame "8x5" {
        w41 = TRUE
        n761 = Not(x="Boolean 42") -> (.not. x?=w73:bool)
        n762 = Not(x="Boolean 9") -> (.not. x?=w72:bool)
        n763 = Not(x="Boolean 25") -> (.not. x?=w71:bool)
        n764 = Not(x="Boolean 33") -> (.not. x?=w70:bool)
        n765 = Not(x="Boolean 2") -> (.not. x?=w69:bool)
        n766 = Not(x="Boolean 10") -> (.not. x?=w68:bool)
        n767 = Not(x="Boolean 26") -> (.not. x?=w67:bool)
        n768 = Not(x="Boolean 34") -> (.not. x?=w66:bool)
        n769 = Not(x="Boolean 4") -> (.not. x?=w65:bool)
        n770 = Not(x="Boolean 12") -> (.not. x?=w64:bool)
        n771 = Not(x="Boolean 20") -> (.not. x?=w63:bool)
        n772 = Not(x="Boolean 28") -> (.not. x?=w62:bool)
        n773 = Not(x="Boolean 36") -> (.not. x?=w61:bool)
        n774 = Not(x="Boolean 5") -> (.not. x?=w60:bool)
        n775 = Not(x="Boolean 13") -> (.not. x?=w59:bool)
        n776 = Not(x="Boolean 21") -> (.not. x?=w58:bool)
        n777 = Not(x="Boolean 29") -> (.not. x?=w57:bool)
        n778 = Not(x="Boolean 37") -> (.not. x?=w56:bool)
        n779 = Not(x="Boolean 15") -> (.not. x?=w54:bool)
        n780 = Not(x="Boolean 7") -> (.not. x?=w55:bool)
        n781 = Not(x="Boolean 30") -> (.not. x?=w49:bool)
        n782 = Not(x="Boolean 31") -> (.not. x?=w53:bool)
        n783 = Not(x="Boolean 39") -> (.not. x?=w52:bool)
        n784 = Not(x="Boolean 38") -> (.not. x?=w48:bool)
        n785 = Not(x="Boolean 6") -> (.not. x?=w51:bool)
        n786 = Not(x="Boolean 14") -> (.not. x?=w50:bool)
        n787 = Compound Arithmetic op=AND(w73, w72, w71, w70, w69, w68, w67, w66, w65, w64, w63, w62, w61, w60, w59, w58, w57, w56, w55, w54, w53, w52, w51, w50, w49, w48) -> (w43:bool)
        n788 = property on="Boolean 11" class="Bool (strict)"("Visible"=w41) -> ()  [unwired: 2 in, 2 out]
        n789 = property on="OK Button 10" class="Bool (strict)"("Visible"=w41) -> ()  [unwired: 2 in, 2 out]
        n790 = property on="Boolean 12" class="Bool (strict)"("Visible"=w41) -> ()  [unwired: 2 in, 2 out]
        n791 = property on="Boolean 14" class="Bool (strict)"("Visible"=w41) -> ()  [unwired: 2 in, 2 out]
        n792 = property on="OK Button" class="Bool (strict)"("Visible"=w41) -> ()  [unwired: 2 in, 2 out]
        n793 = property on="Boolean 10" class="Bool (strict)"("Visible"=w41) -> ()  [unwired: 2 in, 2 out]
        n794 = property on="Boolean 13" class="Bool (strict)"("Visible"=w41) -> ()  [unwired: 2 in, 2 out]
        n795 = Compound Arithmetic op=AND("Boolean 17", "Boolean 18", "Boolean 8", "Boolean 16", "Boolean 24", "Boolean 32", "Boolean 40", "Boolean 3", "Boolean 11", "Boolean 19", "Boolean 27", "Boolean 35", "Boolean 23", "Boolean 22", w43) -> (w40:bool)
        n796 = property on="OK Button 11" class="Bool (strict)"("Visible"=w41) -> ()  [unwired: 2 in, 2 out]
        n797 = property on="OK Button 13" class="Bool (strict)"("Visible"=w41) -> ()  [unwired: 2 in, 2 out]
        n798 = property on="Boolean 16" class="Bool (strict)"("Visible"=w41) -> ()  [unwired: 2 in, 2 out]
        n799 = property on="Boolean 17" class="Bool (strict)"("Visible"=w41) -> ()  [unwired: 2 in, 2 out]
        n800 = property on="Boolean 19" class="Bool (strict)"("Visible"=w41) -> ()  [unwired: 2 in, 2 out]
        n801 = property on="Boolean 15" class="Bool (strict)"("Visible"=w41) -> ()  [unwired: 2 in, 2 out]
        n802 = property on="Boolean 18" class="Bool (strict)"("Visible"=w41) -> ()  [unwired: 2 in, 2 out]
        n803 = property on="OK Button 12" class="Bool (strict)"("Visible"=w41) -> ()  [unwired: 2 in, 2 out]
        n804 = property on="OK Button 14" class="Bool (strict)"("Visible"=w41) -> ()  [unwired: 2 in, 2 out]
        n805 = property on="Boolean 20" class="Bool (strict)"("Visible"=w41) -> ()  [unwired: 2 in, 2 out]
        n806 = property on="Boolean 21" class="Bool (strict)"("Visible"=w41) -> ()  [unwired: 2 in, 2 out]
        n807 = property on="Boolean 23" class="Bool (strict)"("Visible"=w41) -> ()  [unwired: 2 in, 2 out]
        n808 = property on="Boolean 2" class="Bool (strict)"("Visible"=w41) -> ()  [unwired: 2 in, 2 out]
        n809 = property on="Boolean 22" class="Bool (strict)"("Visible"=w41) -> ()  [unwired: 2 in, 2 out]
        n810 = Select(t=T2."powrot", s=w40, f=T2."8x5") -> (s? t:f=w42:T2)
        n811 = case shown="True" w40 {
          selector: w40 -> [_ w114]
          frame False {
          }
          frame True {
            n812 = Wait (ms)(milliseconds to wait=u32 4000) -> ()  [unwired: 1 out]
            "Boolean 43" <- w114
          }
        }
        n813 = property on="OK Button 16" class="Bool (strict)"("Visible"=w41) -> ()  [unwired: 2 in, 2 out]
        n814 = property on="OK Button 15" class="Bool (strict)"("Visible"=w41) -> ()  [unwired: 2 in, 2 out]
        n815 = property on="Boolean 25" class="Bool (strict)"("Visible"=w41) -> ()  [unwired: 2 in, 2 out]
        n816 = property on="Boolean 26" class="Bool (strict)"("Visible"=w41) -> ()  [unwired: 2 in, 2 out]
        n817 = property on="Boolean 28" class="Bool (strict)"("Visible"=w41) -> ()  [unwired: 2 in, 2 out]
        n818 = property on="Boolean 24" class="Bool (strict)"("Visible"=w41) -> ()  [unwired: 2 in, 2 out]
        n819 = property on="Boolean 27" class="Bool (strict)"("Visible"=w41) -> ()  [unwired: 2 in, 2 out]
        n820 = property on="OK Button 3" class="Bool (strict)"("Visible"=w41) -> ()  [unwired: 2 in, 2 out]
        n821 = property on="OK Button 2" class="Bool (strict)"("Visible"=w41) -> ()  [unwired: 2 in, 2 out]
        n822 = property on="Boolean 3" class="Bool (strict)"("Visible"=w41) -> ()  [unwired: 2 in, 2 out]
        n823 = property on="Boolean 30" class="Bool (strict)"("Visible"=w41) -> ()  [unwired: 2 in, 2 out]
        n824 = property on="Boolean 32" class="Bool (strict)"("Visible"=w41) -> ()  [unwired: 2 in, 2 out]
        n825 = property on="Boolean 29" class="Bool (strict)"("Visible"=w41) -> ()  [unwired: 2 in, 2 out]
        n826 = property on="Boolean 31" class="Bool (strict)"("Visible"=w41) -> ()  [unwired: 2 in, 2 out]
        n827 = property on="OK Button 5" class="Bool (strict)"("Visible"=w41) -> ()  [unwired: 2 in, 2 out]
        n828 = property on="OK Button 4" class="Bool (strict)"("Visible"=w41) -> ()  [unwired: 2 in, 2 out]
        n829 = property on="Boolean 34" class="Bool (strict)"("Visible"=w41) -> ()  [unwired: 2 in, 2 out]
        n830 = property on="Boolean 35" class="Bool (strict)"("Visible"=w41) -> ()  [unwired: 2 in, 2 out]
        n831 = property on="Boolean 37" class="Bool (strict)"("Visible"=w41) -> ()  [unwired: 2 in, 2 out]
        n832 = property on="Boolean 33" class="Bool (strict)"("Visible"=w41) -> ()  [unwired: 2 in, 2 out]
        n833 = property on="Boolean 36" class="Bool (strict)"("Visible"=w41) -> ()  [unwired: 2 in, 2 out]
        n834 = property on="OK Button 7" class="Bool (strict)"("Visible"=w41) -> ()  [unwired: 2 in, 2 out]
        n835 = property on="OK Button 6" class="Bool (strict)"("Visible"=w41) -> ()  [unwired: 2 in, 2 out]
        n836 = property on="Boolean 39" class="Bool (strict)"("Visible"=w41) -> ()  [unwired: 2 in, 2 out]
        n837 = property on="Boolean 4" class="Bool (strict)"("Visible"=w41) -> ()  [unwired: 2 in, 2 out]
        n838 = property on="Boolean 9" class="Bool (strict)"("Visible"=w41) -> ()  [unwired: 2 in, 2 out]
        n839 = property on="Boolean 38" class="Bool (strict)"("Visible"=w41) -> ()  [unwired: 2 in, 2 out]
        n840 = property on="Boolean 40" class="Bool (strict)"("Visible"=w41) -> ()  [unwired: 2 in, 2 out]
        n841 = property on="OK Button 9" class="Bool (strict)"("Visible"=w41) -> ()  [unwired: 2 in, 2 out]
        n842 = property on="OK Button 8" class="Bool (strict)"("Visible"=w41) -> ()  [unwired: 2 in, 2 out]
        n843 = property on="Boolean 5" class="Bool (strict)"("Visible"=w41) -> ()  [unwired: 2 in, 2 out]
        n844 = property on="Boolean 6" class="Bool (strict)"("Visible"=w41) -> ()  [unwired: 2 in, 2 out]
        n845 = property on="Boolean 8" class="Bool (strict)"("Visible"=w41) -> ()  [unwired: 2 in, 2 out]
        n846 = property on="Boolean 42" class="Bool (strict)"("Visible"=w41) -> ()  [unwired: 2 in, 2 out]
        n847 = property on="Boolean 7" class="Bool (strict)"("Visible"=w41) -> ()  [unwired: 2 in, 2 out]
        n848 = property on="Boolean 43" class="Bool (strict)"("Visible"=w41) -> ()  [unwired: 2 in, 2 out]
      }
      frame "11x9" {
        w115 = TRUE
        n849 = property on="OK Button 70" class="Bool (strict)"("Visible"=w115) -> ()  [unwired: 2 in, 2 out]
        n850 = property on="Boolean 100" class="Bool (strict)"("Visible"=w115) -> ()  [unwired: 2 in, 2 out]
        n851 = property on="Boolean 101" class="Bool (strict)"("Visible"=w115) -> ()  [unwired: 2 in, 2 out]
        n852 = property on="Boolean 102" class="Bool (strict)"("Visible"=w115) -> ()  [unwired: 2 in, 2 out]
        n853 = property on="Boolean 103" class="Bool (strict)"("Visible"=w115) -> ()  [unwired: 2 in, 2 out]
        n854 = property on="Boolean 104" class="Bool (strict)"("Visible"=w115) -> ()  [unwired: 2 in, 2 out]
        n855 = property on="Boolean 105" class="Bool (strict)"("Visible"=w115) -> ()  [unwired: 2 in, 2 out]
        n856 = property on="Boolean 106" class="Bool (strict)"("Visible"=w115) -> ()  [unwired: 2 in, 2 out]
        n857 = property on="Boolean 107" class="Bool (strict)"("Visible"=w115) -> ()  [unwired: 2 in, 2 out]
        n858 = property on="Boolean 108" class="Bool (strict)"("Visible"=w115) -> ()  [unwired: 2 in, 2 out]
        n859 = property on="Boolean 109" class="Bool (strict)"("Visible"=w115) -> ()  [unwired: 2 in, 2 out]
        n860 = property on="Boolean 41" class="Bool (strict)"("Visible"=w115) -> ()  [unwired: 2 in, 2 out]
        n861 = property on="Boolean" class="Bool (strict)"("Visible"=w115) -> ()  [unwired: 2 in, 2 out]
        n862 = property on="Boolean 114" class="Bool (strict)"("Visible"=w115) -> ()  [unwired: 2 in, 2 out]
        n863 = property on="OK Button 36" class="Bool (strict)"("Visible"=w115) -> ()  [unwired: 2 in, 2 out]
        n864 = property on="Boolean 110" class="Bool (strict)"("Visible"=w115) -> ()  [unwired: 2 in, 2 out]
        n865 = property on="Boolean 111" class="Bool (strict)"("Visible"=w115) -> ()  [unwired: 2 in, 2 out]
        n866 = property on="Boolean 112" class="Bool (strict)"("Visible"=w115) -> ()  [unwired: 2 in, 2 out]
        n867 = property on="Boolean 115" class="Bool (strict)"("Visible"=w115) -> ()  [unwired: 2 in, 2 out]
        n868 = property on="Boolean 116" class="Bool (strict)"("Visible"=w115) -> ()  [unwired: 2 in, 2 out]
        n869 = property on="Boolean 117" class="Bool (strict)"("Visible"=w115) -> ()  [unwired: 2 in, 2 out]
        n870 = property on="Boolean 118" class="Bool (strict)"("Visible"=w115) -> ()  [unwired: 2 in, 2 out]
        n871 = property on="Boolean 113" class="Bool (strict)"("Visible"=w115) -> ()  [unwired: 2 in, 2 out]
        n872 = property on="Boolean 119" class="Bool (strict)"("Visible"=w115) -> ()  [unwired: 2 in, 2 out]
        n873 = property on="OK Button 37" class="Bool (strict)"("Visible"=w115) -> ()  [unwired: 2 in, 2 out]
        n874 = property on="Boolean 125" class="Bool (strict)"("Visible"=w115) -> ()  [unwired: 2 in, 2 out]
        n875 = property on="Boolean 120" class="Bool (strict)"("Visible"=w115) -> ()  [unwired: 2 in, 2 out]
        n876 = property on="Boolean 121" class="Bool (strict)"("Visible"=w115) -> ()  [unwired: 2 in, 2 out]
        n877 = property on="Boolean 122" class="Bool (strict)"("Visible"=w115) -> ()  [unwired: 2 in, 2 out]
        n878 = property on="Boolean 123" class="Bool (strict)"("Visible"=w115) -> ()  [unwired: 2 in, 2 out]
        n879 = property on="Boolean 126" class="Bool (strict)"("Visible"=w115) -> ()  [unwired: 2 in, 2 out]
        n880 = property on="Boolean 127" class="Bool (strict)"("Visible"=w115) -> ()  [unwired: 2 in, 2 out]
        n881 = property on="Boolean 128" class="Bool (strict)"("Visible"=w115) -> ()  [unwired: 2 in, 2 out]
        n882 = property on="Boolean 129" class="Bool (strict)"("Visible"=w115) -> ()  [unwired: 2 in, 2 out]
        n883 = property on="Boolean 124" class="Bool (strict)"("Visible"=w115) -> ()  [unwired: 2 in, 2 out]
        n884 = property on="Boolean 130" class="Bool (strict)"("Visible"=w115) -> ()  [unwired: 2 in, 2 out]
        n885 = property on="Boolean 45" class="Bool (strict)"("Visible"=w115) -> ()  [unwired: 2 in, 2 out]
        n886 = property on="Boolean 140" class="Bool (strict)"("Visible"=w115) -> ()  [unwired: 2 in, 2 out]
        n887 = property on="Boolean 136" class="Bool (strict)"("Visible"=w115) -> ()  [unwired: 2 in, 2 out]
        n888 = property on="Boolean 131" class="Bool (strict)"("Visible"=w115) -> ()  [unwired: 2 in, 2 out]
        n889 = property on="Boolean 132" class="Bool (strict)"("Visible"=w115) -> ()  [unwired: 2 in, 2 out]
        n890 = property on="Boolean 133" class="Bool (strict)"("Visible"=w115) -> ()  [unwired: 2 in, 2 out]
        n891 = property on="Boolean 134" class="Bool (strict)"("Visible"=w115) -> ()  [unwired: 2 in, 2 out]
        n892 = property on="Boolean 141" class="Bool (strict)"("Visible"=w115) -> ()  [unwired: 2 in, 2 out]
        n893 = property on="Boolean 137" class="Bool (strict)"("Visible"=w115) -> ()  [unwired: 2 in, 2 out]
        n894 = property on="Boolean 138" class="Bool (strict)"("Visible"=w115) -> ()  [unwired: 2 in, 2 out]
        n895 = property on="Boolean 139" class="Bool (strict)"("Visible"=w115) -> ()  [unwired: 2 in, 2 out]
        n896 = property on="Boolean 135" class="Bool (strict)"("Visible"=w115) -> ()  [unwired: 2 in, 2 out]
        n897 = property on="Boolean 44" class="Bool (strict)"("Visible"=w115) -> ()  [unwired: 2 in, 2 out]
        n898 = property on="OK Button 43" class="Bool (strict)"("Visible"=w115) -> ()  [unwired: 2 in, 2 out]
        n899 = property on="OK Button 38" class="Bool (strict)"("Visible"=w115) -> ()  [unwired: 2 in, 2 out]
        n900 = property on="OK Button 39" class="Bool (strict)"("Visible"=w115) -> ()  [unwired: 2 in, 2 out]
        n901 = property on="OK Button 40" class="Bool (strict)"("Visible"=w115) -> ()  [unwired: 2 in, 2 out]
        n902 = property on="OK Button 41" class="Bool (strict)"("Visible"=w115) -> ()  [unwired: 2 in, 2 out]
        n903 = property on="OK Button 44" class="Bool (strict)"("Visible"=w115) -> ()  [unwired: 2 in, 2 out]
        n904 = property on="OK Button 45" class="Bool (strict)"("Visible"=w115) -> ()  [unwired: 2 in, 2 out]
        n905 = property on="OK Button 46" class="Bool (strict)"("Visible"=w115) -> ()  [unwired: 2 in, 2 out]
        n906 = property on="OK Button 47" class="Bool (strict)"("Visible"=w115) -> ()  [unwired: 2 in, 2 out]
        n907 = property on="OK Button 42" class="Bool (strict)"("Visible"=w115) -> ()  [unwired: 2 in, 2 out]
        n908 = property on="OK Button 48" class="Bool (strict)"("Visible"=w115) -> ()  [unwired: 2 in, 2 out]
        n909 = property on="OK Button 49" class="Bool (strict)"("Visible"=w115) -> ()  [unwired: 2 in, 2 out]
        n910 = property on="OK Button 67" class="Bool (strict)"("Visible"=w115) -> ()  [unwired: 2 in, 2 out]
        n911 = property on="OK Button 62" class="Bool (strict)"("Visible"=w115) -> ()  [unwired: 2 in, 2 out]
        n912 = property on="OK Button 63" class="Bool (strict)"("Visible"=w115) -> ()  [unwired: 2 in, 2 out]
        n913 = property on="OK Button 64" class="Bool (strict)"("Visible"=w115) -> ()  [unwired: 2 in, 2 out]
        n914 = property on="OK Button 65" class="Bool (strict)"("Visible"=w115) -> ()  [unwired: 2 in, 2 out]
        n915 = property on="OK Button 68" class="Bool (strict)"("Visible"=w115) -> ()  [unwired: 2 in, 2 out]
        n916 = property on="OK Button 69" class="Bool (strict)"("Visible"=w115) -> ()  [unwired: 2 in, 2 out]
        n917 = property on="Boolean 70" class="Bool (strict)"("Visible"=w115) -> ()  [unwired: 2 in, 2 out]
        n918 = property on="OK Button 71" class="Bool (strict)"("Visible"=w115) -> ()  [unwired: 2 in, 2 out]
        n919 = property on="OK Button 66" class="Bool (strict)"("Visible"=w115) -> ()  [unwired: 2 in, 2 out]
        n920 = property on="OK Button 72" class="Bool (strict)"("Visible"=w115) -> ()  [unwired: 2 in, 2 out]
        n921 = property on="OK Button 74" class="Bool (strict)"("Visible"=w115) -> ()  [unwired: 2 in, 2 out]
        n922 = property on="Boolean 52" class="Bool (strict)"("Visible"=w115) -> ()  [unwired: 2 in, 2 out]
        n923 = property on="Boolean 48" class="Bool (strict)"("Visible"=w115) -> ()  [unwired: 2 in, 2 out]
        n924 = property on="Boolean 49" class="Bool (strict)"("Visible"=w115) -> ()  [unwired: 2 in, 2 out]
        n925 = property on="Boolean 47" class="Bool (strict)"("Visible"=w115) -> ()  [unwired: 2 in, 2 out]
        n926 = property on="Boolean 50" class="Bool (strict)"("Visible"=w115) -> ()  [unwired: 2 in, 2 out]
        n927 = property on="Boolean 58" class="Bool (strict)"("Visible"=w115) -> ()  [unwired: 2 in, 2 out]
        n928 = property on="Boolean 53" class="Bool (strict)"("Visible"=w115) -> ()  [unwired: 2 in, 2 out]
        n929 = property on="Boolean 54" class="Bool (strict)"("Visible"=w115) -> ()  [unwired: 2 in, 2 out]
        n930 = property on="Boolean 55" class="Bool (strict)"("Visible"=w115) -> ()  [unwired: 2 in, 2 out]
        n931 = property on="Boolean 56" class="Bool (strict)"("Visible"=w115) -> ()  [unwired: 2 in, 2 out]
        n932 = property on="Boolean 51" class="Bool (strict)"("Visible"=w115) -> ()  [unwired: 2 in, 2 out]
        n933 = property on="Boolean 57" class="Bool (strict)"("Visible"=w115) -> ()  [unwired: 2 in, 2 out]
        n934 = property on="Boolean 63" class="Bool (strict)"("Visible"=w115) -> ()  [unwired: 2 in, 2 out]
        n935 = property on="Boolean 59" class="Bool (strict)"("Visible"=w115) -> ()  [unwired: 2 in, 2 out]
        n936 = property on="Boolean 60" class="Bool (strict)"("Visible"=w115) -> ()  [unwired: 2 in, 2 out]
        n937 = property on="Boolean 61" class="Bool (strict)"("Visible"=w115) -> ()  [unwired: 2 in, 2 out]
        n938 = property on="Boolean 69" class="Bool (strict)"("Visible"=w115) -> ()  [unwired: 2 in, 2 out]
        n939 = property on="Boolean 64" class="Bool (strict)"("Visible"=w115) -> ()  [unwired: 2 in, 2 out]
        n940 = property on="Boolean 65" class="Bool (strict)"("Visible"=w115) -> ()  [unwired: 2 in, 2 out]
        n941 = property on="Boolean 66" class="Bool (strict)"("Visible"=w115) -> ()  [unwired: 2 in, 2 out]
        n942 = property on="Boolean 67" class="Bool (strict)"("Visible"=w115) -> ()  [unwired: 2 in, 2 out]
        n943 = property on="OK Button 73" class="Bool (strict)"("Visible"=w115) -> ()  [unwired: 2 in, 2 out]
        n944 = property on="Boolean 62" class="Bool (strict)"("Visible"=w115) -> ()  [unwired: 2 in, 2 out]
        n945 = property on="Boolean 68" class="Bool (strict)"("Visible"=w115) -> ()  [unwired: 2 in, 2 out]
        n946 = property on="Boolean 74" class="Bool (strict)"("Visible"=w115) -> ()  [unwired: 2 in, 2 out]
        n947 = property on="Boolean 70" class="Bool (strict)"("Visible"=w115) -> ()  [unwired: 2 in, 2 out]
        n948 = property on="Boolean 71" class="Bool (strict)"("Visible"=w115) -> ()  [unwired: 2 in, 2 out]
        n949 = property on="Boolean 72" class="Bool (strict)"("Visible"=w115) -> ()  [unwired: 2 in, 2 out]
        n950 = property on="Boolean 75" class="Bool (strict)"("Visible"=w115) -> ()  [unwired: 2 in, 2 out]
        n951 = property on="Boolean 76" class="Bool (strict)"("Visible"=w115) -> ()  [unwired: 2 in, 2 out]
        n952 = property on="Boolean 77" class="Bool (strict)"("Visible"=w115) -> ()  [unwired: 2 in, 2 out]
        n953 = property on="Boolean 78" class="Bool (strict)"("Visible"=w115) -> ()  [unwired: 2 in, 2 out]
        n954 = property on="Boolean 73" class="Bool (strict)"("Visible"=w115) -> ()  [unwired: 2 in, 2 out]
        n955 = property on="Boolean 79" class="Bool (strict)"("Visible"=w115) -> ()  [unwired: 2 in, 2 out]
        n956 = property on="OK Button 76" class="Bool (strict)"("Visible"=w115) -> ()  [unwired: 2 in, 2 out]
        n957 = property on="OK Button 75" class="Bool (strict)"("Visible"=w115) -> ()  [unwired: 2 in, 2 out]
        n958 = property on="Boolean 85" class="Bool (strict)"("Visible"=w115) -> ()  [unwired: 2 in, 2 out]
        n959 = property on="Boolean 80" class="Bool (strict)"("Visible"=w115) -> ()  [unwired: 2 in, 2 out]
        n960 = property on="Boolean 81" class="Bool (strict)"("Visible"=w115) -> ()  [unwired: 2 in, 2 out]
        n961 = property on="Boolean 82" class="Bool (strict)"("Visible"=w115) -> ()  [unwired: 2 in, 2 out]
        n962 = property on="Boolean 83" class="Bool (strict)"("Visible"=w115) -> ()  [unwired: 2 in, 2 out]
        n963 = property on="Boolean 90" class="Bool (strict)"("Visible"=w115) -> ()  [unwired: 2 in, 2 out]
        n964 = property on="Boolean 86" class="Bool (strict)"("Visible"=w115) -> ()  [unwired: 2 in, 2 out]
        n965 = property on="Boolean 87" class="Bool (strict)"("Visible"=w115) -> ()  [unwired: 2 in, 2 out]
        n966 = property on="Boolean 88" class="Bool (strict)"("Visible"=w115) -> ()  [unwired: 2 in, 2 out]
        n967 = property on="Boolean 89" class="Bool (strict)"("Visible"=w115) -> ()  [unwired: 2 in, 2 out]
        n968 = property on="Boolean 84" class="Bool (strict)"("Visible"=w115) -> ()  [unwired: 2 in, 2 out]
        n969 = property on="Boolean 46" class="Bool (strict)"("Visible"=w115) -> ()  [unwired: 2 in, 2 out]
        n970 = property on="Boolean 96" class="Bool (strict)"("Visible"=w115) -> ()  [unwired: 2 in, 2 out]
        n971 = property on="Boolean 91" class="Bool (strict)"("Visible"=w115) -> ()  [unwired: 2 in, 2 out]
        n972 = property on="Boolean 92" class="Bool (strict)"("Visible"=w115) -> ()  [unwired: 2 in, 2 out]
        n973 = property on="Boolean 93" class="Bool (strict)"("Visible"=w115) -> ()  [unwired: 2 in, 2 out]
        n974 = property on="Boolean 94" class="Bool (strict)"("Visible"=w115) -> ()  [unwired: 2 in, 2 out]
        n975 = property on="OK Button 21" class="Bool (strict)"("Visible"=w115) -> ()  [unwired: 2 in, 2 out]
        n976 = property on="Boolean 97" class="Bool (strict)"("Visible"=w115) -> ()  [unwired: 2 in, 2 out]
        n977 = property on="Boolean 98" class="Bool (strict)"("Visible"=w115) -> ()  [unwired: 2 in, 2 out]
        n978 = property on="Boolean 99" class="Bool (strict)"("Visible"=w115) -> ()  [unwired: 2 in, 2 out]
        n979 = property on="OK Butto" class="Bool (strict)"("Visible"=w115) -> ()  [unwired: 2 in, 2 out]
        n980 = property on="Boolean 95" class="Bool (strict)"("Visible"=w115) -> ()  [unwired: 2 in, 2 out]
        n981 = property on="OK Button 17" class="Bool (strict)"("Visible"=w115) -> ()  [unwired: 2 in, 2 out]
        n982 = property on="OK Button 27" class="Bool (strict)"("Visible"=w115) -> ()  [unwired: 2 in, 2 out]
        n983 = property on="OK Button 22" class="Bool (strict)"("Visible"=w115) -> ()  [unwired: 2 in, 2 out]
        n984 = property on="OK Button 23" class="Bool (strict)"("Visible"=w115) -> ()  [unwired: 2 in, 2 out]
        n985 = property on="OK Button 25" class="Bool (strict)"("Visible"=w115) -> ()  [unwired: 2 in, 2 out]
        n986 = property on="OK Button 24" class="Bool (strict)"("Visible"=w115) -> ()  [unwired: 2 in, 2 out]
        n987 = property on="OK Button 35" class="Bool (strict)"("Visible"=w115) -> ()  [unwired: 2 in, 2 out]
        n988 = property on="OK Button 28" class="Bool (strict)"("Visible"=w115) -> ()  [unwired: 2 in, 2 out]
        n989 = property on="OK Button 31" class="Bool (strict)"("Visible"=w115) -> ()  [unwired: 2 in, 2 out]
        n990 = property on="OK Button 32" class="Bool (strict)"("Visible"=w115) -> ()  [unwired: 2 in, 2 out]
        n991 = property on="OK Button 33" class="Bool (strict)"("Visible"=w115) -> ()  [unwired: 2 in, 2 out]
        n992 = property on="OK Button 26" class="Bool (strict)"("Visible"=w115) -> ()  [unwired: 2 in, 2 out]
        n993 = property on="OK Button 34" class="Bool (strict)"("Visible"=w115) -> ()  [unwired: 2 in, 2 out]
        n994 = property on="OK Button 55" class="Bool (strict)"("Visible"=w115) -> ()  [unwired: 2 in, 2 out]
        n995 = property on="OK Button 50" class="Bool (strict)"("Visible"=w115) -> ()  [unwired: 2 in, 2 out]
        n996 = property on="OK Button 51" class="Bool (strict)"("Visible"=w115) -> ()  [unwired: 2 in, 2 out]
        n997 = property on="OK Button 52" class="Bool (strict)"("Visible"=w115) -> ()  [unwired: 2 in, 2 out]
        n998 = property on="OK Button 53" class="Bool (strict)"("Visible"=w115) -> ()  [unwired: 2 in, 2 out]
        n999 = property on="OK Button 56" class="Bool (strict)"("Visible"=w115) -> ()  [unwired: 2 in, 2 out]
        n1000 = property on="OK Button 57" class="Bool (strict)"("Visible"=w115) -> ()  [unwired: 2 in, 2 out]
        n1001 = property on="OK Button 58" class="Bool (strict)"("Visible"=w115) -> ()  [unwired: 2 in, 2 out]
        n1002 = property on="OK Button 59" class="Bool (strict)"("Visible"=w115) -> ()  [unwired: 2 in, 2 out]
        n1003 = property on="OK Button 54" class="Bool (strict)"("Visible"=w115) -> ()  [unwired: 2 in, 2 out]
        n1004 = property on="OK Button 60" class="Bool (strict)"("Visible"=w115) -> ()  [unwired: 2 in, 2 out]
        n1005 = property on="OK Button 61" class="Bool (strict)"("Visible"=w115) -> ()  [unwired: 2 in, 2 out]
        n1006 = Compound Arithmetic op=OR("Boolean 96", "Boolean 84", "Boolean 95", "Boolean 106", "Boolean 61", "Boolean 72", "Boolean 116", "Boolean 127", "Boolean 60", "Boolean 126", "Boolean 48", "Boolean 81", "Boolean 92", "Boolean 103", "Boolean 114", "Boolean 136", "Boolean 47", "Boolean 80", "Boolean 102", "Boolean 135", "Boolean 46", "Boolean 79", "Boolean 90", "Boolean 101", "Boolean 112", "Boolean 134", "Boolean 56", "Boolean 122", "Boolean 55", "Boolean 66", "Boolean 110", "Boolean 121", "Boolean 76", "Boolean 87", "Boolean 98", "Boolean 86") -> (w117:bool)
        n1007 = Not(x=w117) -> (.not. x?=w116:bool)
        n1008 = Compound Arithmetic op=AND("Boolean 52", "Boolean 63", "Boolean 85", "Boolean 74", "Boolean 107", "Boolean 118", "Boolean 129", "Boolean 140", "Boolean 51", "Boolean 62", "Boolean 73", "Boolean 117", "Boolean 128", "Boolean 139", "Boolean 50", "Boolean 83", "Boolean 94", "Boolean 105", "Boolean 138", "Boolean 49", "Boolean 71", "Boolean 82", "Boolean 93", "Boolean 104", "Boolean 115", "Boolean 137", "Boolean 59", "Boolean 70", "Boolean 125", "Boolean 58", "Boolean 69", "Boolean 91", "Boolean 113", "Boolean 124", "Boolean 57", "Boolean 68", "Boolean 123", "Boolean 45", "Boolean 67", "Boolean 78", "Boolean 89", "Boolean 100", "Boolean 44", "Boolean 111", "Boolean 133", "Boolean 77", "Boolean 88", "Boolean 99", "Boolean 132", "Boolean 41", "Boolean 54", "Boolean 65", "Boolean 109", "Boolean 120", "Boolean 131", "Boolean", "Boolean 53", "Boolean 64", "Boolean 75", "Boolean 97", "Boolean 108", "Boolean 119", "Boolean 130", w116) -> (w118:bool)
        n1009 = case shown="True" w118 {
          selector: w118 -> [_ w223]
          frame False {
          }
          frame True {
            n1010 = Wait (ms)(milliseconds to wait=u32 4000) -> ()  [unwired: 1 out]
            "Boolean 141" <- w223
          }
        }
        n1011 = Select(t=T2."powrot", s=w118, f=T2."11x9") -> (s? t:f=w119:T2)
      }
      frame "12x15" {
        w224 = TRUE ("Visible")
        w225 = TRUE ("Visible")
        n1012 = property on="OK Button 109" class="Bool (strict)"("Visible"=w224) -> ()  [unwired: 2 in, 2 out]
        n1013 = property on="OK Button 81" class="Bool (strict)"("Visible"=w224) -> ()  [unwired: 2 in, 2 out]
        n1014 = property on="OK Button 83" class="Bool (strict)"("Visible"=w224) -> ()  [unwired: 2 in, 2 out]
        n1015 = property on="OK Button 77" class="Bool (strict)"("Visible"=w224) -> ()  [unwired: 2 in, 2 out]
        n1016 = property on="OK Button 80" class="Bool (strict)"("Visible"=w224) -> ()  [unwired: 2 in, 2 out]
        n1017 = property on="OK Button 79" class="Bool (strict)"("Visible"=w224) -> ()  [unwired: 2 in, 2 out]
        n1018 = property on="OK Button 143" class="Bool (strict)"("Visible"=w224) -> ()  [unwired: 2 in, 2 out]
        n1019 = property on="OK Button 131" class="Bool (strict)"("Visible"=w224) -> ()  [unwired: 2 in, 2 out]
        n1020 = property on="OK Button 144" class="Bool (strict)"("Visible"=w224) -> ()  [unwired: 2 in, 2 out]
        n1021 = property on="OK Button 82" class="Bool (strict)"("Visible"=w224) -> ()  [unwired: 2 in, 2 out]
        n1022 = property on="OK Button 78" class="Bool (strict)"("Visible"=w224) -> ()  [unwired: 2 in, 2 out]
        n1023 = property on="OK Button 162" class="Bool (strict)"("Visible"=w224) -> ()  [unwired: 2 in, 2 out]
        n1024 = property on="OK Button 154" class="Bool (strict)"("Visible"=w224) -> ()  [unwired: 2 in, 2 out]
        n1025 = property on="OK Button 124" class="Bool (strict)"("Visible"=w224) -> ()  [unwired: 2 in, 2 out]
        n1026 = property on="OK Button 136" class="Bool (strict)"("Visible"=w224) -> ()  [unwired: 2 in, 2 out]
        n1027 = property on="OK Button 110" class="Bool (strict)"("Visible"=w224) -> ()  [unwired: 2 in, 2 out]
        n1028 = property on="OK Button 92" class="Bool (strict)"("Visible"=w224) -> ()  [unwired: 2 in, 2 out]
        n1029 = property on="OK Button 96" class="Bool (strict)"("Visible"=w224) -> ()  [unwired: 2 in, 2 out]
        n1030 = property on="OK Button 132" class="Bool (strict)"("Visible"=w224) -> ()  [unwired: 2 in, 2 out]
        n1031 = property on="OK Button 95" class="Bool (strict)"("Visible"=w224) -> ()  [unwired: 2 in, 2 out]
        n1032 = property on="OK Button 93" class="Bool (strict)"("Visible"=w224) -> ()  [unwired: 2 in, 2 out]
        n1033 = property on="OK Button 97" class="Bool (strict)"("Visible"=w224) -> ()  [unwired: 2 in, 2 out]
        n1034 = property on="OK Button 148" class="Bool (strict)"("Visible"=w224) -> ()  [unwired: 2 in, 2 out]
        n1035 = property on="OK Button 163" class="Bool (strict)"("Visible"=w224) -> ()  [unwired: 2 in, 2 out]
        n1036 = property on="OK Button 155" class="Bool (strict)"("Visible"=w224) -> ()  [unwired: 2 in, 2 out]
        n1037 = property on="OK Button 137" class="Bool (strict)"("Visible"=w224) -> ()  [unwired: 2 in, 2 out]
        n1038 = property on="OK Button 165" class="Bool (strict)"("Visible"=w224) -> ()  [unwired: 2 in, 2 out]
        n1039 = property on="OK Button 125" class="Bool (strict)"("Visible"=w224) -> ()  [unwired: 2 in, 2 out]
        n1040 = property on="OK Button 111" class="Bool (strict)"("Visible"=w224) -> ()  [unwired: 2 in, 2 out]
        n1041 = property on="OK Button 118" class="Bool (strict)"("Visible"=w224) -> ()  [unwired: 2 in, 2 out]
        n1042 = property on="OK Button 117" class="Bool (strict)"("Visible"=w224) -> ()  [unwired: 2 in, 2 out]
        n1043 = property on="OK Button 108" class="Bool (strict)"("Visible"=w224) -> ()  [unwired: 2 in, 2 out]
        n1044 = property on="OK Button 107" class="Bool (strict)"("Visible"=w224) -> ()  [unwired: 2 in, 2 out]
        n1045 = property on="OK Button 114" class="Bool (strict)"("Visible"=w224) -> ()  [unwired: 2 in, 2 out]
        n1046 = property on="OK Button 116" class="Bool (strict)"("Visible"=w224) -> ()  [unwired: 2 in, 2 out]
        n1047 = property on="OK Button 115" class="Bool (strict)"("Visible"=w224) -> ()  [unwired: 2 in, 2 out]
        n1048 = property on="OK Button 145" class="Bool (strict)"("Visible"=w224) -> ()  [unwired: 2 in, 2 out]
        n1049 = property on="OK Button 164" class="Bool (strict)"("Visible"=w224) -> ()  [unwired: 2 in, 2 out]
        n1050 = property on="OK Button 133" class="Bool (strict)"("Visible"=w224) -> ()  [unwired: 2 in, 2 out]
        n1051 = property on="OK Button 156" class="Bool (strict)"("Visible"=w224) -> ()  [unwired: 2 in, 2 out]
        n1052 = property on="OK Button 126" class="Bool (strict)"("Visible"=w224) -> ()  [unwired: 2 in, 2 out]
        n1053 = property on="OK Button 149" class="Bool (strict)"("Visible"=w224) -> ()  [unwired: 2 in, 2 out]
        n1054 = property on="OK Button 138" class="Bool (strict)"("Visible"=w224) -> ()  [unwired: 2 in, 2 out]
        n1055 = property on="OK Button 112" class="Bool (strict)"("Visible"=w224) -> ()  [unwired: 2 in, 2 out]
        n1056 = property on="OK Button 122" class="Bool (strict)"("Visible"=w224) -> ()  [unwired: 2 in, 2 out]
        n1057 = property on="OK Button 119" class="Bool (strict)"("Visible"=w224) -> ()  [unwired: 2 in, 2 out]
        n1058 = property on="OK Button 121" class="Bool (strict)"("Visible"=w224) -> ()  [unwired: 2 in, 2 out]
        n1059 = property on="OK Button 99" class="Bool (strict)"("Visible"=w224) -> ()  [unwired: 2 in, 2 out]
        n1060 = property on="OK Button 120" class="Bool (strict)"("Visible"=w224) -> ()  [unwired: 2 in, 2 out]
        n1061 = property on="OK Button 123" class="Bool (strict)"("Visible"=w224) -> ()  [unwired: 2 in, 2 out]
        n1062 = property on="OK Button 84" class="Bool (strict)"("Visible"=w224) -> ()  [unwired: 2 in, 2 out]
        n1063 = property on="OK Button 135" class="Bool (strict)"("Visible"=w224) -> ()  [unwired: 2 in, 2 out]
        n1064 = property on="OK Button 147" class="Bool (strict)"("Visible"=w224) -> ()  [unwired: 2 in, 2 out]
        n1065 = property on="OK Button 158" class="Bool (strict)"("Visible"=w224) -> ()  [unwired: 2 in, 2 out]
        n1066 = property on="OK Button 150" class="Bool (strict)"("Visible"=w224) -> ()  [unwired: 2 in, 2 out]
        n1067 = property on="OK Button 139" class="Bool (strict)"("Visible"=w224) -> ()  [unwired: 2 in, 2 out]
        n1068 = property on="OK Button 160" class="Bool (strict)"("Visible"=w224) -> ()  [unwired: 2 in, 2 out]
        n1069 = property on="OK Button 127" class="Bool (strict)"("Visible"=w224) -> ()  [unwired: 2 in, 2 out]
        n1070 = property on="OK Button 113" class="Bool (strict)"("Visible"=w224) -> ()  [unwired: 2 in, 2 out]
        n1071 = property on="OK Button 87" class="Bool (strict)"("Visible"=w224) -> ()  [unwired: 2 in, 2 out]
        n1072 = property on="OK Button 86" class="Bool (strict)"("Visible"=w224) -> ()  [unwired: 2 in, 2 out]
        n1073 = property on="OK Button 88" class="Bool (strict)"("Visible"=w224) -> ()  [unwired: 2 in, 2 out]
        n1074 = property on="OK Button 85" class="Bool (strict)"("Visible"=w224) -> ()  [unwired: 2 in, 2 out]
        n1075 = property on="OK Button 91" class="Bool (strict)"("Visible"=w224) -> ()  [unwired: 2 in, 2 out]
        n1076 = property on="OK Button 89" class="Bool (strict)"("Visible"=w224) -> ()  [unwired: 2 in, 2 out]
        n1077 = property on="OK Button 90" class="Bool (strict)"("Visible"=w224) -> ()  [unwired: 2 in, 2 out]
        n1078 = property on="OK Button 159" class="Bool (strict)"("Visible"=w224) -> ()  [unwired: 2 in, 2 out]
        n1079 = property on="OK Button 134" class="Bool (strict)"("Visible"=w224) -> ()  [unwired: 2 in, 2 out]
        n1080 = property on="OK Button 151" class="Bool (strict)"("Visible"=w224) -> ()  [unwired: 2 in, 2 out]
        n1081 = property on="OK Button 140" class="Bool (strict)"("Visible"=w224) -> ()  [unwired: 2 in, 2 out]
        n1082 = property on="OK Button 146" class="Bool (strict)"("Visible"=w224) -> ()  [unwired: 2 in, 2 out]
        n1083 = property on="OK Button 157" class="Bool (strict)"("Visible"=w224) -> ()  [unwired: 2 in, 2 out]
        n1084 = property on="OK Button 128" class="Bool (strict)"("Visible"=w224) -> ()  [unwired: 2 in, 2 out]
        n1085 = for {
          N: 15 -> [_]
          tunnel: bool[][] [[TRUE, TRUE, FALSE, FALSE, FALSE, TRUE, TRUE, FALSE, FALSE, FALSE, TRUE, TRUE], [TRUE, TRUE, FALSE, FALSE, FALSE, TRUE, TRUE, FALSE, FALSE, FALSE, TRUE, TRUE], [TRUE, TRUE, TRUE, TRUE, TRUE, TRUE, TRUE, TRUE, TRUE, TRUE, TRUE, TRUE], [FALSE, TRUE, TRUE, TRUE, TRUE, FALSE, FALSE, TRUE, TRUE, TRUE, TRUE, FALSE], [FALSE, FALSE, TRUE, TRUE, FALSE, FALSE, FALSE, FALSE, TRUE, TRUE, FALSE, FALSE], [FALSE, FALSE, TRUE, FALSE, FALSE, FALSE, FALSE, FALSE, FALSE, TRUE, FALSE, FALSE], [TRUE, TRUE, TRUE, TRUE, TRUE, TRUE, TRUE, TRUE, TRUE, TRUE, TRUE, TRUE], [TRUE, FALSE, FALSE, FALSE, FALSE, FALSE, FALSE, FALSE, FALSE, FALSE, FALSE, TRUE], [TRUE, FALSE, TRUE, TRUE, TRUE, FALSE, TRUE, FALSE, FALSE, TRUE, FALSE, TRUE], [TRUE, FALSE, TRUE, FALSE, TRUE, FALSE, TRUE, FALSE, TRUE, FALSE, FALSE, TRUE], [TRUE, FALSE, TRUE, TRUE, TRUE, FALSE, TRUE, TRUE, FALSE, FALSE, FALSE, TRUE], [TRUE, FALSE, TRUE, FALSE, FALSE, FALSE, TRUE, FALSE, TRUE, FALSE, FALSE, TRUE], [TRUE, FALSE, TRUE, FALSE, FALSE, FALSE, TRUE, FALSE, FALSE, TRUE, FALSE, TRUE], [TRUE, FALSE, FALSE, FALSE, FALSE, FALSE, FALSE, FALSE, FALSE, FALSE, FALSE, TRUE], [TRUE, TRUE, TRUE, TRUE, TRUE, TRUE, TRUE, TRUE, TRUE, TRUE, TRUE, TRUE]] ("Array 3") -> [w239] mode=indexing
          tunnel: "Array" -> [w238] mode=indexing
          tunnel: [w237] -> w232 mode=indexing
          n1086 = for {
            N: 12 -> [_]
            tunnel: w239 -> [w243] mode=indexing
            tunnel: w238 -> [w242] mode=indexing
            tunnel: [w241] -> w237 mode=indexing
            n1087 = Not Exclusive Or(1:w242, 2:w243) -> (0:w241:bool)
          }
        }
        n1088 = property on="OK Button 104" class="Bool (strict)"("Visible"=w224) -> ()  [unwired: 2 in, 2 out]
        n1089 = property on="OK Button 101" class="Bool (strict)"("Visible"=w224) -> ()  [unwired: 2 in, 2 out]
        n1090 = property on="OK Button 102" class="Bool (strict)"("Visible"=w224) -> ()  [unwired: 2 in, 2 out]
        n1091 = property on="OK Button 103" class="Bool (strict)"("Visible"=w224) -> ()  [unwired: 2 in, 2 out]
        n1092 = property on="OK Button 105" class="Bool (strict)"("Visible"=w224) -> ()  [unwired: 2 in, 2 out]
        n1093 = property on="OK Button 100" class="Bool (strict)"("Visible"=w224) -> ()  [unwired: 2 in, 2 out]
        n1094 = property on="OK Button 130" class="Bool (strict)"("Visible"=w224) -> ()  [unwired: 2 in, 2 out]
        n1095 = property on="OK Button 142" class="Bool (strict)"("Visible"=w224) -> ()  [unwired: 2 in, 2 out]
        n1096 = property on="OK Button 153" class="Bool (strict)"("Visible"=w224) -> ()  [unwired: 2 in, 2 out]
        n1097 = property on="OK Button 161" class="Bool (strict)"("Visible"=w224) -> ()  [unwired: 2 in, 2 out]
        n1098 = property on="OK Button 152" class="Bool (strict)"("Visible"=w224) -> ()  [unwired: 2 in, 2 out]
        n1099 = property on="OK Button 141" class="Bool (strict)"("Visible"=w224) -> ()  [unwired: 2 in, 2 out]
        n1100 = property on="OK Button 129" class="Bool (strict)"("Visible"=w224) -> ()  [unwired: 2 in, 2 out]
        n1101 = And Array Elements(Boolean array=w232) -> (logical AND=w229:bool)
        n1102 = case shown="True" w229 {
          selector: w229 -> [_ w236]
          frame False {
          }
          frame True {
            n1103 = Wait (ms)(milliseconds to wait=u32 4000) -> ()  [unwired: 1 out]
            "Boolean 142" <- w236
          }
        }
        n1104 = Select(t=T2."powrot", s=w229, f=T2."12x15") -> (s? t:f=w228:T2)
        n1105 = property on="Boolean 142" class="Bool (strict)"("Visible"=w225) -> ()  [unwired: 2 in, 2 out]
        n1106 = property on="Array" class="Arr (strict)"("Visible"=w225) -> ()  [unwired: 2 in, 2 out]
      }
      frame "13x14" {
        w244 = TRUE ("Visible")
        w245 = TRUE ("Visible")
        n1107 = property on="aOK Button 22" class="Bool (strict)"("Visible"=w244) -> ()  [unwired: 2 in, 2 out]
        n1108 = property on="aOK Button 24" class="Bool (strict)"("Visible"=w244) -> ()  [unwired: 2 in, 2 out]
        n1109 = property on="aOK Button 21" class="Bool (strict)"("Visible"=w244) -> ()  [unwired: 2 in, 2 out]
        n1110 = property on="aOK Button 23" class="Bool (strict)"("Visible"=w244) -> ()  [unwired: 2 in, 2 out]
        n1111 = property on="aOK Button 14" class="Bool (strict)"("Visible"=w244) -> ()  [unwired: 2 in, 2 out]
        n1112 = property on="aOK Button 17" class="Bool (strict)"("Visible"=w244) -> ()  [unwired: 2 in, 2 out]
        n1113 = property on="aOK Button 13" class="Bool (strict)"("Visible"=w244) -> ()  [unwired: 2 in, 2 out]
        n1114 = property on="aOK Button 15" class="Bool (strict)"("Visible"=w244) -> ()  [unwired: 2 in, 2 out]
        n1115 = property on="aOK Button 19" class="Bool (strict)"("Visible"=w244) -> ()  [unwired: 2 in, 2 out]
        n1116 = property on="aOK Button 20" class="Bool (strict)"("Visible"=w244) -> ()  [unwired: 2 in, 2 out]
        n1117 = property on="aOK Button 18" class="Bool (strict)"("Visible"=w244) -> ()  [unwired: 2 in, 2 out]
        n1118 = property on="aOK Button 2" class="Bool (strict)"("Visible"=w244) -> ()  [unwired: 2 in, 2 out]
        n1119 = property on="aOK Button" class="Bool (strict)"("Visible"=w244) -> ()  [unwired: 2 in, 2 out]
        n1120 = property on="aOK Button 12" class="Bool (strict)"("Visible"=w244) -> ()  [unwired: 2 in, 2 out]
        n1121 = property on="aOK Button 10" class="Bool (strict)"("Visible"=w244) -> ()  [unwired: 2 in, 2 out]
        n1122 = property on="aOK Button 11" class="Bool (strict)"("Visible"=w244) -> ()  [unwired: 2 in, 2 out]
        n1123 = property on="aOK Button 37" class="Bool (strict)"("Visible"=w244) -> ()  [unwired: 2 in, 2 out]
        n1124 = property on="aOK Button 38" class="Bool (strict)"("Visible"=w244) -> ()  [unwired: 2 in, 2 out]
        n1125 = property on="aOK Button 36" class="Bool (strict)"("Visible"=w244) -> ()  [unwired: 2 in, 2 out]
        n1126 = property on="aOK Button 39" class="Bool (strict)"("Visible"=w244) -> ()  [unwired: 2 in, 2 out]
        n1127 = property on="aOK Button 3" class="Bool (strict)"("Visible"=w244) -> ()  [unwired: 2 in, 2 out]
        n1128 = property on="aOK Button 31" class="Bool (strict)"("Visible"=w244) -> ()  [unwired: 2 in, 2 out]
        n1129 = property on="aOK Button 29" class="Bool (strict)"("Visible"=w244) -> ()  [unwired: 2 in, 2 out]
        n1130 = property on="aOK Button 30" class="Bool (strict)"("Visible"=w244) -> ()  [unwired: 2 in, 2 out]
        n1131 = property on="aOK Button 33" class="Bool (strict)"("Visible"=w244) -> ()  [unwired: 2 in, 2 out]
        n1132 = property on="aOK Button 35" class="Bool (strict)"("Visible"=w244) -> ()  [unwired: 2 in, 2 out]
        n1133 = property on="aOK Button 32" class="Bool (strict)"("Visible"=w244) -> ()  [unwired: 2 in, 2 out]
        n1134 = property on="aOK Button 34" class="Bool (strict)"("Visible"=w244) -> ()  [unwired: 2 in, 2 out]
        n1135 = property on="aOK Button 26" class="Bool (strict)"("Visible"=w244) -> ()  [unwired: 2 in, 2 out]
        n1136 = property on="aOK Button 28" class="Bool (strict)"("Visible"=w244) -> ()  [unwired: 2 in, 2 out]
        n1137 = property on="aOK Button 25" class="Bool (strict)"("Visible"=w244) -> ()  [unwired: 2 in, 2 out]
        n1138 = property on="aOK Button 27" class="Bool (strict)"("Visible"=w244) -> ()  [unwired: 2 in, 2 out]
        n1139 = property on="aOK Button 52" class="Bool (strict)"("Visible"=w244) -> ()  [unwired: 2 in, 2 out]
        n1140 = property on="aOK Button 54" class="Bool (strict)"("Visible"=w244) -> ()  [unwired: 2 in, 2 out]
        n1141 = property on="aOK Button 51" class="Bool (strict)"("Visible"=w244) -> ()  [unwired: 2 in, 2 out]
        n1142 = property on="aOK Button 53" class="Bool (strict)"("Visible"=w244) -> ()  [unwired: 2 in, 2 out]
        n1143 = property on="aOK Button 45" class="Bool (strict)"("Visible"=w244) -> ()  [unwired: 2 in, 2 out]
        n1144 = property on="aOK Button 47" class="Bool (strict)"("Visible"=w244) -> ()  [unwired: 2 in, 2 out]
        n1145 = property on="aOK Button 44" class="Bool (strict)"("Visible"=w244) -> ()  [unwired: 2 in, 2 out]
        n1146 = property on="aOK Button 46" class="Bool (strict)"("Visible"=w244) -> ()  [unwired: 2 in, 2 out]
        n1147 = property on="aOK Button 49" class="Bool (strict)"("Visible"=w244) -> ()  [unwired: 2 in, 2 out]
        n1148 = property on="aOK Button 50" class="Bool (strict)"("Visible"=w244) -> ()  [unwired: 2 in, 2 out]
        n1149 = property on="aOK Button 48" class="Bool (strict)"("Visible"=w244) -> ()  [unwired: 2 in, 2 out]
        n1150 = property on="aOK Button 5" class="Bool (strict)"("Visible"=w244) -> ()  [unwired: 2 in, 2 out]
        n1151 = property on="aOK Button 40" class="Bool (strict)"("Visible"=w244) -> ()  [unwired: 2 in, 2 out]
        n1152 = property on="aOK Button 42" class="Bool (strict)"("Visible"=w244) -> ()  [unwired: 2 in, 2 out]
        n1153 = property on="aOK Button 4" class="Bool (strict)"("Visible"=w244) -> ()  [unwired: 2 in, 2 out]
        n1154 = property on="aOK Button 41" class="Bool (strict)"("Visible"=w244) -> ()  [unwired: 2 in, 2 out]
        n1155 = property on="aOK Button 68" class="Bool (strict)"("Visible"=w244) -> ()  [unwired: 2 in, 2 out]
        n1156 = property on="aOK Button 7" class="Bool (strict)"("Visible"=w244) -> ()  [unwired: 2 in, 2 out]
        n1157 = property on="aOK Button 67" class="Bool (strict)"("Visible"=w244) -> ()  [unwired: 2 in, 2 out]
        n1158 = property on="aOK Button 69" class="Bool (strict)"("Visible"=w244) -> ()  [unwired: 2 in, 2 out]
        n1159 = property on="aOK Button 60" class="Bool (strict)"("Visible"=w244) -> ()  [unwired: 2 in, 2 out]
        n1160 = property on="aOK Button 62" class="Bool (strict)"("Visible"=w244) -> ()  [unwired: 2 in, 2 out]
        n1161 = property on="aOK Button 6" class="Bool (strict)"("Visible"=w244) -> ()  [unwired: 2 in, 2 out]
        n1162 = property on="aOK Button 61" class="Bool (strict)"("Visible"=w244) -> ()  [unwired: 2 in, 2 out]
        n1163 = property on="aOK Button 64" class="Bool (strict)"("Visible"=w244) -> ()  [unwired: 2 in, 2 out]
        n1164 = property on="aOK Button 66" class="Bool (strict)"("Visible"=w244) -> ()  [unwired: 2 in, 2 out]
        n1165 = property on="aOK Button 63" class="Bool (strict)"("Visible"=w244) -> ()  [unwired: 2 in, 2 out]
        n1166 = property on="aOK Button 65" class="Bool (strict)"("Visible"=w244) -> ()  [unwired: 2 in, 2 out]
        n1167 = property on="aOK Button 56" class="Bool (strict)"("Visible"=w244) -> ()  [unwired: 2 in, 2 out]
        n1168 = property on="aOK Button 59" class="Bool (strict)"("Visible"=w244) -> ()  [unwired: 2 in, 2 out]
        n1169 = property on="aOK Button 55" class="Bool (strict)"("Visible"=w244) -> ()  [unwired: 2 in, 2 out]
        n1170 = property on="aOK Button 58" class="Bool (strict)"("Visible"=w244) -> ()  [unwired: 2 in, 2 out]
        n1171 = property on="aOK Button 75" class="Bool (strict)"("Visible"=w244) -> ()  [unwired: 2 in, 2 out]
        n1172 = property on="aOK Button 9" class="Bool (strict)"("Visible"=w244) -> ()  [unwired: 2 in, 2 out]
        n1173 = property on="aOK Button 74" class="Bool (strict)"("Visible"=w244) -> ()  [unwired: 2 in, 2 out]
        n1174 = property on="aOK Button 8" class="Bool (strict)"("Visible"=w244) -> ()  [unwired: 2 in, 2 out]
        n1175 = property on="aOK Button 71" class="Bool (strict)"("Visible"=w244) -> ()  [unwired: 2 in, 2 out]
        n1176 = property on="aOK Button 73" class="Bool (strict)"("Visible"=w244) -> ()  [unwired: 2 in, 2 out]
        n1177 = property on="aOK Button 70" class="Bool (strict)"("Visible"=w244) -> ()  [unwired: 2 in, 2 out]
        n1178 = property on="aOK Button 72" class="Bool (strict)"("Visible"=w244) -> ()  [unwired: 2 in, 2 out]
        n1179 = for {
          N: 14 -> [_]
          tunnel: bool[][] [[TRUE, TRUE, TRUE, TRUE, TRUE, FALSE, FALSE, FALSE, TRUE, TRUE, TRUE, TRUE, TRUE], [TRUE, TRUE, TRUE, TRUE, TRUE, TRUE, FALSE, FALSE, TRUE, FALSE, FALSE, FALSE, TRUE], [TRUE, TRUE, TRUE, TRUE, TRUE, FALSE, TRUE, FALSE, TRUE, TRUE, FALSE, FALSE, TRUE], [TRUE, TRUE, TRUE, TRUE, FALSE, TRUE, TRUE, TRUE, TRUE, FALSE, TRUE, FALSE, TRUE], [TRUE, TRUE, TRUE, TRUE, TRUE, TRUE, TRUE, TRUE, FALSE, TRUE, TRUE, TRUE, TRUE], [TRUE, TRUE, FALSE, TRUE, TRUE, TRUE, TRUE, FALSE, TRUE, TRUE, FALSE, TRUE, TRUE], [TRUE, TRUE, FALSE, FALSE, FALSE, TRUE, TRUE, TRUE, TRUE, TRUE, FALSE, TRUE, TRUE], [TRUE, TRUE, FALSE, FALSE, FALSE, FALSE, FALSE, TRUE, TRUE, TRUE, FALSE, TRUE, TRUE], [TRUE, TRUE, FALSE, FALSE, FALSE, FALSE, FALSE, FALSE, FALSE, TRUE, FALSE, TRUE, TRUE], [FALSE, FALSE, FALSE, FALSE, FALSE, FALSE, FALSE, FALSE, FALSE, FALSE, FALSE, FALSE, FALSE], [TRUE, TRUE, FALSE, FALSE, FALSE, FALSE, FALSE, FALSE, FALSE, TRUE, FALSE, TRUE, TRUE], [TRUE, TRUE, FALSE, FALSE, FALSE, FALSE, FALSE, TRUE, TRUE, TRUE, FALSE, TRUE, TRUE], [TRUE, TRUE, FALSE, FALSE, FALSE, TRUE, TRUE, TRUE, TRUE, TRUE, FALSE, TRUE, TRUE], [TRUE, TRUE, FALSE, TRUE, TRUE, TRUE, TRUE, TRUE, TRUE, TRUE, FALSE, TRUE, TRUE], [FALSE, FALSE, FALSE, FALSE, FALSE, FALSE, FALSE, FALSE, FALSE, FALSE, FALSE, FALSE, FALSE]] ("Array 3") -> [w259] mode=indexing
          tunnel: "Array 2" -> [w258] mode=indexing
          tunnel: [w257] -> w253 mode=indexing
          n1180 = for {
            N: 13 -> [_]
            tunnel: w259 -> [w263] mode=indexing
            tunnel: w258 -> [w262] mode=indexing
            tunnel: [w261] -> w257 mode=indexing
            n1181 = Not Exclusive Or(1:w262, 2:w263) -> (0:w261:bool)
          }
        }
        n1182 = And Array Elements(Boolean array=w253) -> (logical AND=w252:bool)
        n1183 = case shown="True" w252 {
          selector: w252 -> [_ w256]
          frame False {
          }
          frame True {
            n1184 = Wait (ms)(milliseconds to wait=u32 4000) -> ()  [unwired: 1 out]
            "Boolean 143" <- w256
          }
        }
        n1185 = Select(t=T2."powrot", s=w252, f=T2."13x14") -> (s? t:f=w247:T2)
        n1186 = property on="Array 2" class="Arr (strict)"("Visible"=w245) -> ()  [unwired: 2 in, 2 out]
        n1187 = property on="Boolean 143" class="Bool (strict)"("Visible"=w245) -> ()  [unwired: 2 in, 2 out]
      }
      frame "koniec" {
        w264 = FALSE ("Visible")
        w265 = FALSE ("Visible")
        w266 = FALSE ("Visible")
        w267 = FALSE ("Visible")
        w268 = FALSE
        w269 = FALSE
        n1188 = property on="Boolean 142" class="Bool (strict)"("Visible"=w267) -> ()  [unwired: 2 in, 2 out]
        n1189 = property on="Array" class="Arr (strict)"("Visible"=w267) -> ()  [unwired: 2 in, 2 out]
        n1190 = property on="OK Button 109" class="Bool (strict)"("Visible"=w266) -> ()  [unwired: 2 in, 2 out]
        n1191 = property on="OK Button 81" class="Bool (strict)"("Visible"=w266) -> ()  [unwired: 2 in, 2 out]
        n1192 = property on="OK Button 83" class="Bool (strict)"("Visible"=w266) -> ()  [unwired: 2 in, 2 out]
        n1193 = property on="OK Button 77" class="Bool (strict)"("Visible"=w266) -> ()  [unwired: 2 in, 2 out]
        n1194 = property on="OK Button 80" class="Bool (strict)"("Visible"=w266) -> ()  [unwired: 2 in, 2 out]
        n1195 = property on="OK Button 79" class="Bool (strict)"("Visible"=w266) -> ()  [unwired: 2 in, 2 out]
        n1196 = property on="OK Button 143" class="Bool (strict)"("Visible"=w266) -> ()  [unwired: 2 in, 2 out]
        n1197 = property on="OK Button 131" class="Bool (strict)"("Visible"=w266) -> ()  [unwired: 2 in, 2 out]
        n1198 = property on="OK Button 144" class="Bool (strict)"("Visible"=w266) -> ()  [unwired: 2 in, 2 out]
        n1199 = property on="OK Button 82" class="Bool (strict)"("Visible"=w266) -> ()  [unwired: 2 in, 2 out]
        n1200 = property on="OK Button 78" class="Bool (strict)"("Visible"=w266) -> ()  [unwired: 2 in, 2 out]
        n1201 = property on="OK Button 162" class="Bool (strict)"("Visible"=w266) -> ()  [unwired: 2 in, 2 out]
        n1202 = property on="OK Button 154" class="Bool (strict)"("Visible"=w266) -> ()  [unwired: 2 in, 2 out]
        n1203 = property on="OK Button 124" class="Bool (strict)"("Visible"=w266) -> ()  [unwired: 2 in, 2 out]
        n1204 = property on="OK Button 136" class="Bool (strict)"("Visible"=w266) -> ()  [unwired: 2 in, 2 out]
        n1205 = property on="Array 2" class="Arr (strict)"("Visible"=w265) -> ()  [unwired: 2 in, 2 out]
        n1206 = property on="Boolean 143" class="Bool (strict)"("Visible"=w265) -> ()  [unwired: 2 in, 2 out]
        n1207 = property on="OK Button 110" class="Bool (strict)"("Visible"=w266) -> ()  [unwired: 2 in, 2 out]
        n1208 = property on="OK Button 92" class="Bool (strict)"("Visible"=w266) -> ()  [unwired: 2 in, 2 out]
        n1209 = property on="OK Button 96" class="Bool (strict)"("Visible"=w266) -> ()  [unwired: 2 in, 2 out]
        n1210 = property on="OK Button 132" class="Bool (strict)"("Visible"=w266) -> ()  [unwired: 2 in, 2 out]
        n1211 = property on="OK Button 95" class="Bool (strict)"("Visible"=w266) -> ()  [unwired: 2 in, 2 out]
        n1212 = property on="OK Button 93" class="Bool (strict)"("Visible"=w266) -> ()  [unwired: 2 in, 2 out]
        n1213 = property on="OK Button 97" class="Bool (strict)"("Visible"=w266) -> ()  [unwired: 2 in, 2 out]
        n1214 = property on="OK Button 148" class="Bool (strict)"("Visible"=w266) -> ()  [unwired: 2 in, 2 out]
        n1215 = property on="OK Button 163" class="Bool (strict)"("Visible"=w266) -> ()  [unwired: 2 in, 2 out]
        n1216 = property on="OK Button 155" class="Bool (strict)"("Visible"=w266) -> ()  [unwired: 2 in, 2 out]
        n1217 = property on="OK Button 137" class="Bool (strict)"("Visible"=w266) -> ()  [unwired: 2 in, 2 out]
        n1218 = property on="OK Button 165" class="Bool (strict)"("Visible"=w266) -> ()  [unwired: 2 in, 2 out]
        n1219 = property on="OK Button 125" class="Bool (strict)"("Visible"=w266) -> ()  [unwired: 2 in, 2 out]
        n1220 = property on="OK Button 111" class="Bool (strict)"("Visible"=w266) -> ()  [unwired: 2 in, 2 out]
        n1221 = property on="OK Button 118" class="Bool (strict)"("Visible"=w266) -> ()  [unwired: 2 in, 2 out]
        n1222 = property on="OK Button 117" class="Bool (strict)"("Visible"=w266) -> ()  [unwired: 2 in, 2 out]
        n1223 = property on="OK Button 108" class="Bool (strict)"("Visible"=w266) -> ()  [unwired: 2 in, 2 out]
        n1224 = property on="OK Button 107" class="Bool (strict)"("Visible"=w266) -> ()  [unwired: 2 in, 2 out]
        n1225 = property on="OK Button 114" class="Bool (strict)"("Visible"=w266) -> ()  [unwired: 2 in, 2 out]
        n1226 = property on="OK Button 116" class="Bool (strict)"("Visible"=w266) -> ()  [unwired: 2 in, 2 out]
        n1227 = property on="OK Button 115" class="Bool (strict)"("Visible"=w266) -> ()  [unwired: 2 in, 2 out]
        n1228 = property on="OK Button 145" class="Bool (strict)"("Visible"=w266) -> ()  [unwired: 2 in, 2 out]
        n1229 = property on="OK Button 164" class="Bool (strict)"("Visible"=w266) -> ()  [unwired: 2 in, 2 out]
        n1230 = property on="OK Button 133" class="Bool (strict)"("Visible"=w266) -> ()  [unwired: 2 in, 2 out]
        n1231 = property on="OK Button 156" class="Bool (strict)"("Visible"=w266) -> ()  [unwired: 2 in, 2 out]
        n1232 = property on="OK Button 126" class="Bool (strict)"("Visible"=w266) -> ()  [unwired: 2 in, 2 out]
        n1233 = property on="OK Button 149" class="Bool (strict)"("Visible"=w266) -> ()  [unwired: 2 in, 2 out]
        n1234 = property on="OK Button 138" class="Bool (strict)"("Visible"=w266) -> ()  [unwired: 2 in, 2 out]
        n1235 = property on="OK Button 112" class="Bool (strict)"("Visible"=w266) -> ()  [unwired: 2 in, 2 out]
        n1236 = property on="OK Button 122" class="Bool (strict)"("Visible"=w266) -> ()  [unwired: 2 in, 2 out]
        n1237 = property on="OK Button 119" class="Bool (strict)"("Visible"=w266) -> ()  [unwired: 2 in, 2 out]
        n1238 = property on="OK Button 121" class="Bool (strict)"("Visible"=w266) -> ()  [unwired: 2 in, 2 out]
        n1239 = property on="OK Button 99" class="Bool (strict)"("Visible"=w266) -> ()  [unwired: 2 in, 2 out]
        n1240 = property on="OK Button 120" class="Bool (strict)"("Visible"=w266) -> ()  [unwired: 2 in, 2 out]
        n1241 = property on="OK Button 123" class="Bool (strict)"("Visible"=w266) -> ()  [unwired: 2 in, 2 out]
        n1242 = property on="OK Button 84" class="Bool (strict)"("Visible"=w266) -> ()  [unwired: 2 in, 2 out]
        n1243 = property on="OK Button 135" class="Bool (strict)"("Visible"=w266) -> ()  [unwired: 2 in, 2 out]
        n1244 = property on="OK Button 147" class="Bool (strict)"("Visible"=w266) -> ()  [unwired: 2 in, 2 out]
        n1245 = property on="OK Button 158" class="Bool (strict)"("Visible"=w266) -> ()  [unwired: 2 in, 2 out]
        n1246 = property on="OK Button 150" class="Bool (strict)"("Visible"=w266) -> ()  [unwired: 2 in, 2 out]
        n1247 = property on="OK Button 139" class="Bool (strict)"("Visible"=w266) -> ()  [unwired: 2 in, 2 out]
        n1248 = property on="OK Button 160" class="Bool (strict)"("Visible"=w266) -> ()  [unwired: 2 in, 2 out]
        n1249 = property on="OK Button 127" class="Bool (strict)"("Visible"=w266) -> ()  [unwired: 2 in, 2 out]
        n1250 = property on="OK Button 113" class="Bool (strict)"("Visible"=w266) -> ()  [unwired: 2 in, 2 out]
        n1251 = property on="OK Button 87" class="Bool (strict)"("Visible"=w266) -> ()  [unwired: 2 in, 2 out]
        n1252 = property on="OK Button 86" class="Bool (strict)"("Visible"=w266) -> ()  [unwired: 2 in, 2 out]
        n1253 = property on="OK Button 88" class="Bool (strict)"("Visible"=w266) -> ()  [unwired: 2 in, 2 out]
        n1254 = property on="OK Button 85" class="Bool (strict)"("Visible"=w266) -> ()  [unwired: 2 in, 2 out]
        n1255 = property on="OK Button 91" class="Bool (strict)"("Visible"=w266) -> ()  [unwired: 2 in, 2 out]
        n1256 = property on="OK Button 89" class="Bool (strict)"("Visible"=w266) -> ()  [unwired: 2 in, 2 out]
        n1257 = property on="OK Button 90" class="Bool (strict)"("Visible"=w266) -> ()  [unwired: 2 in, 2 out]
        n1258 = property on="OK Button 159" class="Bool (strict)"("Visible"=w266) -> ()  [unwired: 2 in, 2 out]
        n1259 = property on="OK Button 134" class="Bool (strict)"("Visible"=w266) -> ()  [unwired: 2 in, 2 out]
        n1260 = property on="OK Button 151" class="Bool (strict)"("Visible"=w266) -> ()  [unwired: 2 in, 2 out]
        n1261 = property on="OK Button 140" class="Bool (strict)"("Visible"=w266) -> ()  [unwired: 2 in, 2 out]
        n1262 = property on="OK Button 146" class="Bool (strict)"("Visible"=w266) -> ()  [unwired: 2 in, 2 out]
        n1263 = property on="OK Button 157" class="Bool (strict)"("Visible"=w266) -> ()  [unwired: 2 in, 2 out]
        n1264 = property on="OK Button 128" class="Bool (strict)"("Visible"=w266) -> ()  [unwired: 2 in, 2 out]
        n1265 = property on="OK Button 104" class="Bool (strict)"("Visible"=w266) -> ()  [unwired: 2 in, 2 out]
        n1266 = property on="OK Button 101" class="Bool (strict)"("Visible"=w266) -> ()  [unwired: 2 in, 2 out]
        n1267 = property on="OK Button 102" class="Bool (strict)"("Visible"=w266) -> ()  [unwired: 2 in, 2 out]
        n1268 = property on="OK Button 103" class="Bool (strict)"("Visible"=w266) -> ()  [unwired: 2 in, 2 out]
        n1269 = property on="OK Button 105" class="Bool (strict)"("Visible"=w266) -> ()  [unwired: 2 in, 2 out]
        n1270 = property on="OK Button 100" class="Bool (strict)"("Visible"=w266) -> ()  [unwired: 2 in, 2 out]
        n1271 = property on="OK Button 130" class="Bool (strict)"("Visible"=w266) -> ()  [unwired: 2 in, 2 out]
        n1272 = property on="OK Button 142" class="Bool (strict)"("Visible"=w266) -> ()  [unwired: 2 in, 2 out]
        n1273 = property on="OK Button 153" class="Bool (strict)"("Visible"=w266) -> ()  [unwired: 2 in, 2 out]
        n1274 = property on="OK Button 161" class="Bool (strict)"("Visible"=w266) -> ()  [unwired: 2 in, 2 out]
        n1275 = property on="OK Button 152" class="Bool (strict)"("Visible"=w266) -> ()  [unwired: 2 in, 2 out]
        n1276 = property on="OK Button 141" class="Bool (strict)"("Visible"=w266) -> ()  [unwired: 2 in, 2 out]
        n1277 = property on="OK Button 129" class="Bool (strict)"("Visible"=w266) -> ()  [unwired: 2 in, 2 out]
        n1278 = property on="Boolean 100" class="Bool (strict)"("Visible"=w268) -> ()  [unwired: 2 in, 2 out]
        n1279 = property on="Boolean 101" class="Bool (strict)"("Visible"=w268) -> ()  [unwired: 2 in, 2 out]
        n1280 = property on="Boolean 102" class="Bool (strict)"("Visible"=w268) -> ()  [unwired: 2 in, 2 out]
        n1281 = property on="Boolean 103" class="Bool (strict)"("Visible"=w268) -> ()  [unwired: 2 in, 2 out]
        n1282 = property on="Boolean 104" class="Bool (strict)"("Visible"=w268) -> ()  [unwired: 2 in, 2 out]
        n1283 = property on="Boolean 105" class="Bool (strict)"("Visible"=w268) -> ()  [unwired: 2 in, 2 out]
        n1284 = property on="Boolean 106" class="Bool (strict)"("Visible"=w268) -> ()  [unwired: 2 in, 2 out]
        n1285 = property on="Boolean 107" class="Bool (strict)"("Visible"=w268) -> ()  [unwired: 2 in, 2 out]
        n1286 = property on="Boolean 108" class="Bool (strict)"("Visible"=w268) -> ()  [unwired: 2 in, 2 out]
        n1287 = property on="Boolean 109" class="Bool (strict)"("Visible"=w268) -> ()  [unwired: 2 in, 2 out]
        n1288 = property on="Boolean 41" class="Bool (strict)"("Visible"=w268) -> ()  [unwired: 2 in, 2 out]
        n1289 = property on="Boolean" class="Bool (strict)"("Visible"=w268) -> ()  [unwired: 2 in, 2 out]
        n1290 = property on="OK Button 70" class="Bool (strict)"("Visible"=w268) -> ()  [unwired: 2 in, 2 out]
        n1291 = property on="Boolean 114" class="Bool (strict)"("Visible"=w268) -> ()  [unwired: 2 in, 2 out]
        n1292 = property on="OK Button 36" class="Bool (strict)"("Visible"=w268) -> ()  [unwired: 2 in, 2 out]
        n1293 = property on="Boolean 110" class="Bool (strict)"("Visible"=w268) -> ()  [unwired: 2 in, 2 out]
        n1294 = property on="Boolean 111" class="Bool (strict)"("Visible"=w268) -> ()  [unwired: 2 in, 2 out]
        n1295 = property on="Boolean 112" class="Bool (strict)"("Visible"=w268) -> ()  [unwired: 2 in, 2 out]
        n1296 = property on="Boolean 115" class="Bool (strict)"("Visible"=w268) -> ()  [unwired: 2 in, 2 out]
        n1297 = property on="Boolean 116" class="Bool (strict)"("Visible"=w268) -> ()  [unwired: 2 in, 2 out]
        n1298 = property on="Boolean 117" class="Bool (strict)"("Visible"=w268) -> ()  [unwired: 2 in, 2 out]
        n1299 = property on="Boolean 118" class="Bool (strict)"("Visible"=w268) -> ()  [unwired: 2 in, 2 out]
        n1300 = property on="Boolean 113" class="Bool (strict)"("Visible"=w268) -> ()  [unwired: 2 in, 2 out]
        n1301 = property on="Boolean 119" class="Bool (strict)"("Visible"=w268) -> ()  [unwired: 2 in, 2 out]
        n1302 = property on="OK Button 37" class="Bool (strict)"("Visible"=w268) -> ()  [unwired: 2 in, 2 out]
        n1303 = property on="Boolean 125" class="Bool (strict)"("Visible"=w268) -> ()  [unwired: 2 in, 2 out]
        n1304 = property on="Boolean 120" class="Bool (strict)"("Visible"=w268) -> ()  [unwired: 2 in, 2 out]
        n1305 = property on="Boolean 121" class="Bool (strict)"("Visible"=w268) -> ()  [unwired: 2 in, 2 out]
        n1306 = property on="Boolean 122" class="Bool (strict)"("Visible"=w268) -> ()  [unwired: 2 in, 2 out]
        n1307 = property on="Boolean 123" class="Bool (strict)"("Visible"=w268) -> ()  [unwired: 2 in, 2 out]
        n1308 = property on="Boolean 126" class="Bool (strict)"("Visible"=w268) -> ()  [unwired: 2 in, 2 out]
        n1309 = property on="Boolean 127" class="Bool (strict)"("Visible"=w268) -> ()  [unwired: 2 in, 2 out]
        n1310 = property on="Boolean 128" class="Bool (strict)"("Visible"=w268) -> ()  [unwired: 2 in, 2 out]
        n1311 = property on="Boolean 129" class="Bool (strict)"("Visible"=w268) -> ()  [unwired: 2 in, 2 out]
        n1312 = property on="Boolean 124" class="Bool (strict)"("Visible"=w268) -> ()  [unwired: 2 in, 2 out]
        n1313 = property on="Boolean 130" class="Bool (strict)"("Visible"=w268) -> ()  [unwired: 2 in, 2 out]
        n1314 = property on="Boolean 45" class="Bool (strict)"("Visible"=w268) -> ()  [unwired: 2 in, 2 out]
        n1315 = property on="Boolean 140" class="Bool (strict)"("Visible"=w268) -> ()  [unwired: 2 in, 2 out]
        n1316 = property on="Boolean 136" class="Bool (strict)"("Visible"=w268) -> ()  [unwired: 2 in, 2 out]
        n1317 = property on="Boolean 131" class="Bool (strict)"("Visible"=w268) -> ()  [unwired: 2 in, 2 out]
        n1318 = property on="Boolean 132" class="Bool (strict)"("Visible"=w268) -> ()  [unwired: 2 in, 2 out]
        n1319 = property on="Boolean 133" class="Bool (strict)"("Visible"=w268) -> ()  [unwired: 2 in, 2 out]
        n1320 = property on="Boolean 134" class="Bool (strict)"("Visible"=w268) -> ()  [unwired: 2 in, 2 out]
        n1321 = property on="Boolean 141" class="Bool (strict)"("Visible"=w268) -> ()  [unwired: 2 in, 2 out]
        n1322 = property on="Boolean 137" class="Bool (strict)"("Visible"=w268) -> ()  [unwired: 2 in, 2 out]
        n1323 = property on="Boolean 138" class="Bool (strict)"("Visible"=w268) -> ()  [unwired: 2 in, 2 out]
        n1324 = property on="Boolean 139" class="Bool (strict)"("Visible"=w268) -> ()  [unwired: 2 in, 2 out]
        n1325 = property on="Boolean 135" class="Bool (strict)"("Visible"=w268) -> ()  [unwired: 2 in, 2 out]
        n1326 = property on="Boolean 44" class="Bool (strict)"("Visible"=w268) -> ()  [unwired: 2 in, 2 out]
        n1327 = property on="OK Button 43" class="Bool (strict)"("Visible"=w268) -> ()  [unwired: 2 in, 2 out]
        n1328 = property on="OK Button 38" class="Bool (strict)"("Visible"=w268) -> ()  [unwired: 2 in, 2 out]
        n1329 = property on="OK Button 39" class="Bool (strict)"("Visible"=w268) -> ()  [unwired: 2 in, 2 out]
        n1330 = property on="OK Button 40" class="Bool (strict)"("Visible"=w268) -> ()  [unwired: 2 in, 2 out]
        n1331 = property on="OK Button 41" class="Bool (strict)"("Visible"=w268) -> ()  [unwired: 2 in, 2 out]
        n1332 = property on="OK Button 44" class="Bool (strict)"("Visible"=w268) -> ()  [unwired: 2 in, 2 out]
        n1333 = property on="OK Button 45" class="Bool (strict)"("Visible"=w268) -> ()  [unwired: 2 in, 2 out]
        n1334 = property on="OK Button 46" class="Bool (strict)"("Visible"=w268) -> ()  [unwired: 2 in, 2 out]
        n1335 = property on="OK Button 47" class="Bool (strict)"("Visible"=w268) -> ()  [unwired: 2 in, 2 out]
        n1336 = property on="OK Button 42" class="Bool (strict)"("Visible"=w268) -> ()  [unwired: 2 in, 2 out]
        n1337 = property on="OK Button 48" class="Bool (strict)"("Visible"=w268) -> ()  [unwired: 2 in, 2 out]
        n1338 = property on="OK Button 49" class="Bool (strict)"("Visible"=w268) -> ()  [unwired: 2 in, 2 out]
        n1339 = property on="Boolean 11" class="Bool (strict)"("Visible"=w269) -> ()  [unwired: 2 in, 2 out]
        n1340 = property on="OK Button 10" class="Bool (strict)"("Visible"=w269) -> ()  [unwired: 2 in, 2 out]
        n1341 = property on="Boolean 12" class="Bool (strict)"("Visible"=w269) -> ()  [unwired: 2 in, 2 out]
        n1342 = property on="Boolean 14" class="Bool (strict)"("Visible"=w269) -> ()  [unwired: 2 in, 2 out]
        n1343 = property on="OK Button" class="Bool (strict)"("Visible"=w269) -> ()  [unwired: 2 in, 2 out]
        n1344 = property on="Boolean 10" class="Bool (strict)"("Visible"=w269) -> ()  [unwired: 2 in, 2 out]
        n1345 = property on="Boolean 13" class="Bool (strict)"("Visible"=w269) -> ()  [unwired: 2 in, 2 out]
        n1346 = property on="OK Button 67" class="Bool (strict)"("Visible"=w268) -> ()  [unwired: 2 in, 2 out]
        n1347 = property on="OK Button 62" class="Bool (strict)"("Visible"=w268) -> ()  [unwired: 2 in, 2 out]
        n1348 = property on="OK Button 63" class="Bool (strict)"("Visible"=w268) -> ()  [unwired: 2 in, 2 out]
        n1349 = property on="OK Button 64" class="Bool (strict)"("Visible"=w268) -> ()  [unwired: 2 in, 2 out]
        n1350 = property on="OK Button 65" class="Bool (strict)"("Visible"=w268) -> ()  [unwired: 2 in, 2 out]
        n1351 = property on="OK Button 68" class="Bool (strict)"("Visible"=w268) -> ()  [unwired: 2 in, 2 out]
        n1352 = property on="OK Button 69" class="Bool (strict)"("Visible"=w268) -> ()  [unwired: 2 in, 2 out]
        n1353 = property on="Boolean 70" class="Bool (strict)"("Visible"=w268) -> ()  [unwired: 2 in, 2 out]
        n1354 = property on="OK Button 71" class="Bool (strict)"("Visible"=w268) -> ()  [unwired: 2 in, 2 out]
        n1355 = property on="OK Button 66" class="Bool (strict)"("Visible"=w268) -> ()  [unwired: 2 in, 2 out]
        n1356 = property on="OK Button 72" class="Bool (strict)"("Visible"=w268) -> ()  [unwired: 2 in, 2 out]
        n1357 = property on="OK Button 74" class="Bool (strict)"("Visible"=w268) -> ()  [unwired: 2 in, 2 out]
        n1358 = property on="OK Button 11" class="Bool (strict)"("Visible"=w269) -> ()  [unwired: 2 in, 2 out]
        n1359 = property on="OK Button 13" class="Bool (strict)"("Visible"=w269) -> ()  [unwired: 2 in, 2 out]
        n1360 = property on="Boolean 16" class="Bool (strict)"("Visible"=w269) -> ()  [unwired: 2 in, 2 out]
        n1361 = property on="Boolean 17" class="Bool (strict)"("Visible"=w269) -> ()  [unwired: 2 in, 2 out]
        n1362 = property on="Boolean 19" class="Bool (strict)"("Visible"=w269) -> ()  [unwired: 2 in, 2 out]
        n1363 = property on="Boolean 15" class="Bool (strict)"("Visible"=w269) -> ()  [unwired: 2 in, 2 out]
        n1364 = property on="Boolean 18" class="Bool (strict)"("Visible"=w269) -> ()  [unwired: 2 in, 2 out]
        n1365 = property on="Boolean 52" class="Bool (strict)"("Visible"=w268) -> ()  [unwired: 2 in, 2 out]
        n1366 = property on="Boolean 48" class="Bool (strict)"("Visible"=w268) -> ()  [unwired: 2 in, 2 out]
        n1367 = property on="Boolean 49" class="Bool (strict)"("Visible"=w268) -> ()  [unwired: 2 in, 2 out]
        n1368 = property on="Boolean 47" class="Bool (strict)"("Visible"=w268) -> ()  [unwired: 2 in, 2 out]
        n1369 = property on="Boolean 50" class="Bool (strict)"("Visible"=w268) -> ()  [unwired: 2 in, 2 out]
        n1370 = property on="Boolean 58" class="Bool (strict)"("Visible"=w268) -> ()  [unwired: 2 in, 2 out]
        n1371 = property on="Boolean 53" class="Bool (strict)"("Visible"=w268) -> ()  [unwired: 2 in, 2 out]
        n1372 = property on="Boolean 54" class="Bool (strict)"("Visible"=w268) -> ()  [unwired: 2 in, 2 out]
        n1373 = property on="Boolean 55" class="Bool (strict)"("Visible"=w268) -> ()  [unwired: 2 in, 2 out]
        n1374 = property on="Boolean 56" class="Bool (strict)"("Visible"=w268) -> ()  [unwired: 2 in, 2 out]
        n1375 = property on="Boolean 51" class="Bool (strict)"("Visible"=w268) -> ()  [unwired: 2 in, 2 out]
        n1376 = property on="Boolean 57" class="Bool (strict)"("Visible"=w268) -> ()  [unwired: 2 in, 2 out]
        n1377 = property on="OK Button 12" class="Bool (strict)"("Visible"=w269) -> ()  [unwired: 2 in, 2 out]
        n1378 = property on="OK Button 14" class="Bool (strict)"("Visible"=w269) -> ()  [unwired: 2 in, 2 out]
        n1379 = property on="Boolean 20" class="Bool (strict)"("Visible"=w269) -> ()  [unwired: 2 in, 2 out]
        n1380 = property on="Boolean 21" class="Bool (strict)"("Visible"=w269) -> ()  [unwired: 2 in, 2 out]
        n1381 = property on="Boolean 23" class="Bool (strict)"("Visible"=w269) -> ()  [unwired: 2 in, 2 out]
        n1382 = property on="Boolean 2" class="Bool (strict)"("Visible"=w269) -> ()  [unwired: 2 in, 2 out]
        n1383 = property on="Boolean 22" class="Bool (strict)"("Visible"=w269) -> ()  [unwired: 2 in, 2 out]
        n1384 = property on="Boolean 63" class="Bool (strict)"("Visible"=w268) -> ()  [unwired: 2 in, 2 out]
        n1385 = property on="Boolean 59" class="Bool (strict)"("Visible"=w268) -> ()  [unwired: 2 in, 2 out]
        n1386 = property on="Boolean 60" class="Bool (strict)"("Visible"=w268) -> ()  [unwired: 2 in, 2 out]
        n1387 = property on="Boolean 61" class="Bool (strict)"("Visible"=w268) -> ()  [unwired: 2 in, 2 out]
        n1388 = property on="Boolean 69" class="Bool (strict)"("Visible"=w268) -> ()  [unwired: 2 in, 2 out]
        n1389 = property on="Boolean 64" class="Bool (strict)"("Visible"=w268) -> ()  [unwired: 2 in, 2 out]
        n1390 = property on="Boolean 65" class="Bool (strict)"("Visible"=w268) -> ()  [unwired: 2 in, 2 out]
        n1391 = property on="Boolean 66" class="Bool (strict)"("Visible"=w268) -> ()  [unwired: 2 in, 2 out]
        n1392 = property on="Boolean 67" class="Bool (strict)"("Visible"=w268) -> ()  [unwired: 2 in, 2 out]
        n1393 = property on="OK Button 73" class="Bool (strict)"("Visible"=w268) -> ()  [unwired: 2 in, 2 out]
        n1394 = property on="Boolean 62" class="Bool (strict)"("Visible"=w268) -> ()  [unwired: 2 in, 2 out]
        n1395 = property on="Boolean 68" class="Bool (strict)"("Visible"=w268) -> ()  [unwired: 2 in, 2 out]
        n1396 = property on="aOK Button 22" class="Bool (strict)"("Visible"=w264) -> ()  [unwired: 2 in, 2 out]
        n1397 = property on="aOK Button 24" class="Bool (strict)"("Visible"=w264) -> ()  [unwired: 2 in, 2 out]
        n1398 = property on="aOK Button 21" class="Bool (strict)"("Visible"=w264) -> ()  [unwired: 2 in, 2 out]
        n1399 = property on="aOK Button 23" class="Bool (strict)"("Visible"=w264) -> ()  [unwired: 2 in, 2 out]
        n1400 = property on="aOK Button 14" class="Bool (strict)"("Visible"=w264) -> ()  [unwired: 2 in, 2 out]
        n1401 = property on="aOK Button 17" class="Bool (strict)"("Visible"=w264) -> ()  [unwired: 2 in, 2 out]
        n1402 = property on="aOK Button 13" class="Bool (strict)"("Visible"=w264) -> ()  [unwired: 2 in, 2 out]
        n1403 = property on="aOK Button 15" class="Bool (strict)"("Visible"=w264) -> ()  [unwired: 2 in, 2 out]
        n1404 = property on="aOK Button 19" class="Bool (strict)"("Visible"=w264) -> ()  [unwired: 2 in, 2 out]
        n1405 = property on="aOK Button 20" class="Bool (strict)"("Visible"=w264) -> ()  [unwired: 2 in, 2 out]
        n1406 = property on="aOK Button 18" class="Bool (strict)"("Visible"=w264) -> ()  [unwired: 2 in, 2 out]
        n1407 = property on="aOK Button 2" class="Bool (strict)"("Visible"=w264) -> ()  [unwired: 2 in, 2 out]
        n1408 = property on="aOK Button" class="Bool (strict)"("Visible"=w264) -> ()  [unwired: 2 in, 2 out]
        n1409 = property on="aOK Button 12" class="Bool (strict)"("Visible"=w264) -> ()  [unwired: 2 in, 2 out]
        n1410 = property on="aOK Button 10" class="Bool (strict)"("Visible"=w264) -> ()  [unwired: 2 in, 2 out]
        n1411 = property on="aOK Button 11" class="Bool (strict)"("Visible"=w264) -> ()  [unwired: 2 in, 2 out]
        n1412 = property on="OK Button 16" class="Bool (strict)"("Visible"=w269) -> ()  [unwired: 2 in, 2 out]
        n1413 = property on="OK Button 15" class="Bool (strict)"("Visible"=w269) -> ()  [unwired: 2 in, 2 out]
        n1414 = property on="Boolean 25" class="Bool (strict)"("Visible"=w269) -> ()  [unwired: 2 in, 2 out]
        n1415 = property on="Boolean 26" class="Bool (strict)"("Visible"=w269) -> ()  [unwired: 2 in, 2 out]
        n1416 = property on="Boolean 28" class="Bool (strict)"("Visible"=w269) -> ()  [unwired: 2 in, 2 out]
        n1417 = property on="Boolean 24" class="Bool (strict)"("Visible"=w269) -> ()  [unwired: 2 in, 2 out]
        n1418 = property on="Boolean 27" class="Bool (strict)"("Visible"=w269) -> ()  [unwired: 2 in, 2 out]
        n1419 = property on="Boolean 74" class="Bool (strict)"("Visible"=w268) -> ()  [unwired: 2 in, 2 out]
        n1420 = property on="Boolean 70" class="Bool (strict)"("Visible"=w268) -> ()  [unwired: 2 in, 2 out]
        n1421 = property on="Boolean 71" class="Bool (strict)"("Visible"=w268) -> ()  [unwired: 2 in, 2 out]
        n1422 = property on="Boolean 72" class="Bool (strict)"("Visible"=w268) -> ()  [unwired: 2 in, 2 out]
        n1423 = property on="Boolean 75" class="Bool (strict)"("Visible"=w268) -> ()  [unwired: 2 in, 2 out]
        n1424 = property on="Boolean 76" class="Bool (strict)"("Visible"=w268) -> ()  [unwired: 2 in, 2 out]
        n1425 = property on="Boolean 77" class="Bool (strict)"("Visible"=w268) -> ()  [unwired: 2 in, 2 out]
        n1426 = property on="Boolean 78" class="Bool (strict)"("Visible"=w268) -> ()  [unwired: 2 in, 2 out]
        n1427 = property on="Boolean 73" class="Bool (strict)"("Visible"=w268) -> ()  [unwired: 2 in, 2 out]
        n1428 = property on="Boolean 79" class="Bool (strict)"("Visible"=w268) -> ()  [unwired: 2 in, 2 out]
        n1429 = property on="OK Button 76" class="Bool (strict)"("Visible"=w268) -> ()  [unwired: 2 in, 2 out]
        n1430 = property on="OK Button 75" class="Bool (strict)"("Visible"=w268) -> ()  [unwired: 2 in, 2 out]
        n1431 = property on="aOK Button 37" class="Bool (strict)"("Visible"=w264) -> ()  [unwired: 2 in, 2 out]
        n1432 = property on="aOK Button 38" class="Bool (strict)"("Visible"=w264) -> ()  [unwired: 2 in, 2 out]
        n1433 = property on="aOK Button 36" class="Bool (strict)"("Visible"=w264) -> ()  [unwired: 2 in, 2 out]
        n1434 = property on="aOK Button 39" class="Bool (strict)"("Visible"=w264) -> ()  [unwired: 2 in, 2 out]
        n1435 = property on="aOK Button 3" class="Bool (strict)"("Visible"=w264) -> ()  [unwired: 2 in, 2 out]
        n1436 = property on="aOK Button 31" class="Bool (strict)"("Visible"=w264) -> ()  [unwired: 2 in, 2 out]
        n1437 = property on="aOK Button 29" class="Bool (strict)"("Visible"=w264) -> ()  [unwired: 2 in, 2 out]
        n1438 = property on="aOK Button 30" class="Bool (strict)"("Visible"=w264) -> ()  [unwired: 2 in, 2 out]
        n1439 = property on="aOK Button 33" class="Bool (strict)"("Visible"=w264) -> ()  [unwired: 2 in, 2 out]
        n1440 = property on="aOK Button 35" class="Bool (strict)"("Visible"=w264) -> ()  [unwired: 2 in, 2 out]
        n1441 = property on="aOK Button 32" class="Bool (strict)"("Visible"=w264) -> ()  [unwired: 2 in, 2 out]
        n1442 = property on="aOK Button 34" class="Bool (strict)"("Visible"=w264) -> ()  [unwired: 2 in, 2 out]
        n1443 = property on="aOK Button 26" class="Bool (strict)"("Visible"=w264) -> ()  [unwired: 2 in, 2 out]
        n1444 = property on="aOK Button 28" class="Bool (strict)"("Visible"=w264) -> ()  [unwired: 2 in, 2 out]
        n1445 = property on="aOK Button 25" class="Bool (strict)"("Visible"=w264) -> ()  [unwired: 2 in, 2 out]
        n1446 = property on="aOK Button 27" class="Bool (strict)"("Visible"=w264) -> ()  [unwired: 2 in, 2 out]
        n1447 = property on="OK Button 3" class="Bool (strict)"("Visible"=w269) -> ()  [unwired: 2 in, 2 out]
        n1448 = property on="OK Button 2" class="Bool (strict)"("Visible"=w269) -> ()  [unwired: 2 in, 2 out]
        n1449 = property on="Boolean 3" class="Bool (strict)"("Visible"=w269) -> ()  [unwired: 2 in, 2 out]
        n1450 = property on="Boolean 30" class="Bool (strict)"("Visible"=w269) -> ()  [unwired: 2 in, 2 out]
        n1451 = property on="Boolean 32" class="Bool (strict)"("Visible"=w269) -> ()  [unwired: 2 in, 2 out]
        n1452 = property on="Boolean 29" class="Bool (strict)"("Visible"=w269) -> ()  [unwired: 2 in, 2 out]
        n1453 = property on="Boolean 31" class="Bool (strict)"("Visible"=w269) -> ()  [unwired: 2 in, 2 out]
        n1454 = property on="Boolean 85" class="Bool (strict)"("Visible"=w268) -> ()  [unwired: 2 in, 2 out]
        n1455 = property on="Boolean 80" class="Bool (strict)"("Visible"=w268) -> ()  [unwired: 2 in, 2 out]
        n1456 = property on="Boolean 81" class="Bool (strict)"("Visible"=w268) -> ()  [unwired: 2 in, 2 out]
        n1457 = property on="Boolean 82" class="Bool (strict)"("Visible"=w268) -> ()  [unwired: 2 in, 2 out]
        n1458 = property on="Boolean 83" class="Bool (strict)"("Visible"=w268) -> ()  [unwired: 2 in, 2 out]
        n1459 = property on="Boolean 90" class="Bool (strict)"("Visible"=w268) -> ()  [unwired: 2 in, 2 out]
        n1460 = property on="Boolean 86" class="Bool (strict)"("Visible"=w268) -> ()  [unwired: 2 in, 2 out]
        n1461 = property on="Boolean 87" class="Bool (strict)"("Visible"=w268) -> ()  [unwired: 2 in, 2 out]
        n1462 = property on="Boolean 88" class="Bool (strict)"("Visible"=w268) -> ()  [unwired: 2 in, 2 out]
        n1463 = property on="Boolean 89" class="Bool (strict)"("Visible"=w268) -> ()  [unwired: 2 in, 2 out]
        n1464 = property on="Boolean 84" class="Bool (strict)"("Visible"=w268) -> ()  [unwired: 2 in, 2 out]
        n1465 = property on="Boolean 46" class="Bool (strict)"("Visible"=w268) -> ()  [unwired: 2 in, 2 out]
        n1466 = property on="aOK Button 52" class="Bool (strict)"("Visible"=w264) -> ()  [unwired: 2 in, 2 out]
        n1467 = property on="aOK Button 54" class="Bool (strict)"("Visible"=w264) -> ()  [unwired: 2 in, 2 out]
        n1468 = property on="aOK Button 51" class="Bool (strict)"("Visible"=w264) -> ()  [unwired: 2 in, 2 out]
        n1469 = property on="aOK Button 53" class="Bool (strict)"("Visible"=w264) -> ()  [unwired: 2 in, 2 out]
        n1470 = property on="aOK Button 45" class="Bool (strict)"("Visible"=w264) -> ()  [unwired: 2 in, 2 out]
        n1471 = property on="aOK Button 47" class="Bool (strict)"("Visible"=w264) -> ()  [unwired: 2 in, 2 out]
        n1472 = property on="aOK Button 44" class="Bool (strict)"("Visible"=w264) -> ()  [unwired: 2 in, 2 out]
        n1473 = property on="aOK Button 46" class="Bool (strict)"("Visible"=w264) -> ()  [unwired: 2 in, 2 out]
        n1474 = property on="aOK Button 49" class="Bool (strict)"("Visible"=w264) -> ()  [unwired: 2 in, 2 out]
        n1475 = property on="aOK Button 50" class="Bool (strict)"("Visible"=w264) -> ()  [unwired: 2 in, 2 out]
        n1476 = property on="aOK Button 48" class="Bool (strict)"("Visible"=w264) -> ()  [unwired: 2 in, 2 out]
        n1477 = property on="aOK Button 5" class="Bool (strict)"("Visible"=w264) -> ()  [unwired: 2 in, 2 out]
        n1478 = property on="aOK Button 40" class="Bool (strict)"("Visible"=w264) -> ()  [unwired: 2 in, 2 out]
        n1479 = property on="aOK Button 42" class="Bool (strict)"("Visible"=w264) -> ()  [unwired: 2 in, 2 out]
        n1480 = property on="aOK Button 4" class="Bool (strict)"("Visible"=w264) -> ()  [unwired: 2 in, 2 out]
        n1481 = property on="aOK Button 41" class="Bool (strict)"("Visible"=w264) -> ()  [unwired: 2 in, 2 out]
        n1482 = property on="OK Button 5" class="Bool (strict)"("Visible"=w269) -> ()  [unwired: 2 in, 2 out]
        n1483 = property on="OK Button 4" class="Bool (strict)"("Visible"=w269) -> ()  [unwired: 2 in, 2 out]
        n1484 = property on="Boolean 34" class="Bool (strict)"("Visible"=w269) -> ()  [unwired: 2 in, 2 out]
        n1485 = property on="Boolean 35" class="Bool (strict)"("Visible"=w269) -> ()  [unwired: 2 in, 2 out]
        n1486 = property on="Boolean 37" class="Bool (strict)"("Visible"=w269) -> ()  [unwired: 2 in, 2 out]
        n1487 = property on="Boolean 33" class="Bool (strict)"("Visible"=w269) -> ()  [unwired: 2 in, 2 out]
        n1488 = property on="Boolean 36" class="Bool (strict)"("Visible"=w269) -> ()  [unwired: 2 in, 2 out]
        n1489 = property on="Boolean 96" class="Bool (strict)"("Visible"=w268) -> ()  [unwired: 2 in, 2 out]
        n1490 = property on="Boolean 91" class="Bool (strict)"("Visible"=w268) -> ()  [unwired: 2 in, 2 out]
        n1491 = property on="Boolean 92" class="Bool (strict)"("Visible"=w268) -> ()  [unwired: 2 in, 2 out]
        n1492 = property on="Boolean 93" class="Bool (strict)"("Visible"=w268) -> ()  [unwired: 2 in, 2 out]
        n1493 = property on="Boolean 94" class="Bool (strict)"("Visible"=w268) -> ()  [unwired: 2 in, 2 out]
        n1494 = property on="OK Button 21" class="Bool (strict)"("Visible"=w268) -> ()  [unwired: 2 in, 2 out]
        n1495 = property on="Boolean 97" class="Bool (strict)"("Visible"=w268) -> ()  [unwired: 2 in, 2 out]
        n1496 = property on="Boolean 98" class="Bool (strict)"("Visible"=w268) -> ()  [unwired: 2 in, 2 out]
        n1497 = property on="Boolean 99" class="Bool (strict)"("Visible"=w268) -> ()  [unwired: 2 in, 2 out]
        n1498 = property on="OK Butto" class="Bool (strict)"("Visible"=w268) -> ()  [unwired: 2 in, 2 out]
        n1499 = property on="Boolean 95" class="Bool (strict)"("Visible"=w268) -> ()  [unwired: 2 in, 2 out]
        n1500 = property on="OK Button 17" class="Bool (strict)"("Visible"=w268) -> ()  [unwired: 2 in, 2 out]
        n1501 = property on="aOK Button 68" class="Bool (strict)"("Visible"=w264) -> ()  [unwired: 2 in, 2 out]
        n1502 = property on="aOK Button 7" class="Bool (strict)"("Visible"=w264) -> ()  [unwired: 2 in, 2 out]
        n1503 = property on="aOK Button 67" class="Bool (strict)"("Visible"=w264) -> ()  [unwired: 2 in, 2 out]
        n1504 = property on="aOK Button 69" class="Bool (strict)"("Visible"=w264) -> ()  [unwired: 2 in, 2 out]
        n1505 = property on="aOK Button 60" class="Bool (strict)"("Visible"=w264) -> ()  [unwired: 2 in, 2 out]
        n1506 = property on="aOK Button 62" class="Bool (strict)"("Visible"=w264) -> ()  [unwired: 2 in, 2 out]
        n1507 = property on="aOK Button 6" class="Bool (strict)"("Visible"=w264) -> ()  [unwired: 2 in, 2 out]
        n1508 = property on="aOK Button 61" class="Bool (strict)"("Visible"=w264) -> ()  [unwired: 2 in, 2 out]
        n1509 = property on="aOK Button 64" class="Bool (strict)"("Visible"=w264) -> ()  [unwired: 2 in, 2 out]
        n1510 = property on="aOK Button 66" class="Bool (strict)"("Visible"=w264) -> ()  [unwired: 2 in, 2 out]
        n1511 = property on="aOK Button 63" class="Bool (strict)"("Visible"=w264) -> ()  [unwired: 2 in, 2 out]
        n1512 = property on="aOK Button 65" class="Bool (strict)"("Visible"=w264) -> ()  [unwired: 2 in, 2 out]
        n1513 = property on="aOK Button 56" class="Bool (strict)"("Visible"=w264) -> ()  [unwired: 2 in, 2 out]
        n1514 = property on="aOK Button 59" class="Bool (strict)"("Visible"=w264) -> ()  [unwired: 2 in, 2 out]
        n1515 = property on="aOK Button 55" class="Bool (strict)"("Visible"=w264) -> ()  [unwired: 2 in, 2 out]
        n1516 = property on="aOK Button 58" class="Bool (strict)"("Visible"=w264) -> ()  [unwired: 2 in, 2 out]
        n1517 = property on="OK Button 7" class="Bool (strict)"("Visible"=w269) -> ()  [unwired: 2 in, 2 out]
        n1518 = property on="OK Button 6" class="Bool (strict)"("Visible"=w269) -> ()  [unwired: 2 in, 2 out]
        n1519 = property on="OK Button 27" class="Bool (strict)"("Visible"=w268) -> ()  [unwired: 2 in, 2 out]
        n1520 = property on="OK Button 22" class="Bool (strict)"("Visible"=w268) -> ()  [unwired: 2 in, 2 out]
        n1521 = property on="OK Button 23" class="Bool (strict)"("Visible"=w268) -> ()  [unwired: 2 in, 2 out]
        n1522 = property on="OK Button 25" class="Bool (strict)"("Visible"=w268) -> ()  [unwired: 2 in, 2 out]
        n1523 = property on="OK Button 24" class="Bool (strict)"("Visible"=w268) -> ()  [unwired: 2 in, 2 out]
        n1524 = property on="OK Button 35" class="Bool (strict)"("Visible"=w268) -> ()  [unwired: 2 in, 2 out]
        n1525 = property on="OK Button 28" class="Bool (strict)"("Visible"=w268) -> ()  [unwired: 2 in, 2 out]
        n1526 = property on="OK Button 31" class="Bool (strict)"("Visible"=w268) -> ()  [unwired: 2 in, 2 out]
        n1527 = property on="OK Button 32" class="Bool (strict)"("Visible"=w268) -> ()  [unwired: 2 in, 2 out]
        n1528 = property on="OK Button 33" class="Bool (strict)"("Visible"=w268) -> ()  [unwired: 2 in, 2 out]
        n1529 = property on="OK Button 26" class="Bool (strict)"("Visible"=w268) -> ()  [unwired: 2 in, 2 out]
        n1530 = property on="OK Button 34" class="Bool (strict)"("Visible"=w268) -> ()  [unwired: 2 in, 2 out]
        n1531 = property on="Boolean 39" class="Bool (strict)"("Visible"=w269) -> ()  [unwired: 2 in, 2 out]
        n1532 = property on="Boolean 4" class="Bool (strict)"("Visible"=w269) -> ()  [unwired: 2 in, 2 out]
        n1533 = property on="Boolean 9" class="Bool (strict)"("Visible"=w269) -> ()  [unwired: 2 in, 2 out]
        n1534 = property on="Boolean 38" class="Bool (strict)"("Visible"=w269) -> ()  [unwired: 2 in, 2 out]
        n1535 = property on="Boolean 40" class="Bool (strict)"("Visible"=w269) -> ()  [unwired: 2 in, 2 out]
        n1536 = property on="aOK Button 75" class="Bool (strict)"("Visible"=w264) -> ()  [unwired: 2 in, 2 out]
        n1537 = property on="aOK Button 9" class="Bool (strict)"("Visible"=w264) -> ()  [unwired: 2 in, 2 out]
        n1538 = property on="aOK Button 74" class="Bool (strict)"("Visible"=w264) -> ()  [unwired: 2 in, 2 out]
        n1539 = property on="aOK Button 8" class="Bool (strict)"("Visible"=w264) -> ()  [unwired: 2 in, 2 out]
        n1540 = property on="aOK Button 71" class="Bool (strict)"("Visible"=w264) -> ()  [unwired: 2 in, 2 out]
        n1541 = property on="aOK Button 73" class="Bool (strict)"("Visible"=w264) -> ()  [unwired: 2 in, 2 out]
        n1542 = property on="aOK Button 70" class="Bool (strict)"("Visible"=w264) -> ()  [unwired: 2 in, 2 out]
        n1543 = property on="aOK Button 72" class="Bool (strict)"("Visible"=w264) -> ()  [unwired: 2 in, 2 out]
        n1544 = property on="OK Button 9" class="Bool (strict)"("Visible"=w269) -> ()  [unwired: 2 in, 2 out]
        n1545 = property on="OK Button 8" class="Bool (strict)"("Visible"=w269) -> ()  [unwired: 2 in, 2 out]
        n1546 = property on="Boolean 5" class="Bool (strict)"("Visible"=w269) -> ()  [unwired: 2 in, 2 out]
        n1547 = property on="Boolean 6" class="Bool (strict)"("Visible"=w269) -> ()  [unwired: 2 in, 2 out]
        n1548 = property on="Boolean 8" class="Bool (strict)"("Visible"=w269) -> ()  [unwired: 2 in, 2 out]
        n1549 = property on="OK Button 55" class="Bool (strict)"("Visible"=w268) -> ()  [unwired: 2 in, 2 out]
        n1550 = property on="Boolean 42" class="Bool (strict)"("Visible"=w269) -> ()  [unwired: 2 in, 2 out]
        n1551 = property on="Boolean 7" class="Bool (strict)"("Visible"=w269) -> ()  [unwired: 2 in, 2 out]
        n1552 = property on="OK Button 50" class="Bool (strict)"("Visible"=w268) -> ()  [unwired: 2 in, 2 out]
        n1553 = property on="OK Button 51" class="Bool (strict)"("Visible"=w268) -> ()  [unwired: 2 in, 2 out]
        n1554 = property on="OK Button 52" class="Bool (strict)"("Visible"=w268) -> ()  [unwired: 2 in, 2 out]
        n1555 = property on="OK Button 53" class="Bool (strict)"("Visible"=w268) -> ()  [unwired: 2 in, 2 out]
        n1556 = property on="OK Button 56" class="Bool (strict)"("Visible"=w268) -> ()  [unwired: 2 in, 2 out]
        n1557 = property on="OK Button 57" class="Bool (strict)"("Visible"=w268) -> ()  [unwired: 2 in, 2 out]
        n1558 = property on="OK Button 58" class="Bool (strict)"("Visible"=w268) -> ()  [unwired: 2 in, 2 out]
        n1559 = property on="OK Button 59" class="Bool (strict)"("Visible"=w268) -> ()  [unwired: 2 in, 2 out]
        n1560 = property on="OK Button 54" class="Bool (strict)"("Visible"=w268) -> ()  [unwired: 2 in, 2 out]
        n1561 = property on="OK Button 60" class="Bool (strict)"("Visible"=w268) -> ()  [unwired: 2 in, 2 out]
        n1562 = property on="OK Button 61" class="Bool (strict)"("Visible"=w268) -> ()  [unwired: 2 in, 2 out]
        n1563 = property on="Boolean 43" class="Bool (strict)"("Visible"=w269) -> ()  [unwired: 2 in, 2 out]
      }
      frame "powrot" {
        n1564 = Two Button Dialog(message="Wygrałeś!!!", 1:"zakończ" ("button name (\"OK\")"), 2:"zagraj jeszcze raz" ("button name (\"OK\")")) -> (T button?=w276:bool)
        n1565 = Select(t=T1."menu", s=w276, f=T1."koniec") -> (s? t:f=w273:T1)
      }
    }
  }
